vi "UNITEST MAIN v01.2.vi"() -> ()   [LabVIEW 2025]
uses:
  controls/LAB-IQ UI Data.ctl
  HEAVE vi's/Heave Write enum.ctl
  487e97dd-ad82-4ea8-9260-f35915b83a37.vi
  fdf22e40-24ec-4bd6-b058-052306f15f2c.vi
  02c5850b-52e8-4ed5-91f8-6f0ad62f4994.vi
  1223eb78-e4c4-4b69-bf80-185c82055158.vi
  e5651a45-6a49-4a3f-b503-ff1eaf449b4a.vi
  support/Message Queue/Enqueue Message (Single).vi
  <vilib>/Utility/error.llb/Error Cluster From Error Code.vi
  <vilib>/ErrorRing/Error Ring.xnode
  support/Message Queue/LAB-IQ Message Queue.lvlib
  support/User Event - Stop/LAB-IQ User Event - Stop.lvlib
  d081153b-36ca-4bc4-8478-749476f82ba4.vi
  HEAVE vi's/Heave Right enum.ctl
panel:
  in  "seconds to wait":dbl=0.0001 format="%#_6p"
  out "error out":errorcluster
  in  "error in (no error)":errorcluster
  out "Heave and Surge Read":string
  in  "min_finetune_floor":dbl=0.15
  in  "min_deadband_floor":dbl=0.05
  in  "fine_tune_pct":dbl=100.0
  out "Start Test Temp":bool
  in  "STOP":bool
  in  "AppLoadSeq scratch":bool
  out "Pulse delta":dbl
  in  "Fine Tune Zone":dbl=10.0
  in  "PID Delay (sec)":dbl=1.0 format="%#_6p"
  in  "Max_pos_limit":dbl=50000000.0
  in  "Min_pos_limit":dbl
  in  "i_limit":dbl=10.0
  in  "Max Step Linit":dbl=10.0
  in  "Init Step":dbl=10.0
  in  "pct_scale":dbl=100.0
  in  "Deadband":dbl=0.1
  in  "Kd":dbl
  in  "Ki":dbl
  in  "Kp":dbl=1.0
  out "Current Position":dbl
  in  "Set Load":dbl
  in  "Current Load":dbl
  in  "Manual Write Heave & Surge":bool
  out "Heave and Surge Write":string
  in  "Heave Loop Delay":dbl
  in  "Heave PID Speed":dbl=15.0
  in  "Surge Jog Speed":dbl=1.0 format="%.4f"
  in  "Heave Jog Speed":dbl=15.0
  in  "SPARE 4":u8
  in  "SPARE 3":u8
  in  "SPARE 2":u8
  in  "SPARE 1":u8
  out "Spare 15":u8
  out "Spare 14":u8
  out "Spare 13":u8
  out "Spare 12":u8
  out "Spare 11":u8
  out "Spare 10":u8
  out "Spare 9":u8
  out "Spare 8":u8
  out "Spare 7":u8
  out "Spare 6":u8
  out "Spare 5":u8
  out "Spare 4":u8
  out "Spare 3":u8
  out "Spare 2":u8
  out "Spare 1":u8
  out "Node Id":u8
  out "Read Heave Temp":bool
  out "fwMinor":u8
  out "fwMajor":u8
  out "faultCode":u16
  out "SURGE POSE":sgl format="%#.6f"
  out "HEAVE POSE":sgl format="%#.6f"
  out "Homed":u8
  out "State":u8
  out "Ack ID":u16
  in  "SPEED":sgl=10000.0
  in  "Distance":sgl=10000.0
  in  "Mode Command":u8=2
  out "Sequence ID":u16
  out "error out Read":errorcluster
  out "error out Write":errorcluster
  out "Heave and Surge Read":string
  out "Load Cell Temp":bool
  in  "Stop Scratch":bool
  in  "Enter Fixed SRR 2":dbl min=0.0 max=0.0 format="%.3f"
  in  "E.Velocity 2":bool=TRUE caption="SRR"
  out "Message":string="Load Entered is out of range!!!"
  in  "Tab Control 3":T1(tab)
  in  "Tab Control 5":enum32{""}(tab)
  in  "Tab Control 14":T2(tab)=enum."Motor Load"
  in  "Ramp MulFac":dbl=2.0
  in  "pulses LoadDiffRamp(2..10)":dbl=9.0
  in  "PulseControlRamp(diff<=3N)":dbl=5.0 min=1.0 max=1000.0 step=1.0 format="%#.1f"
  in  "SetLoadDeadband(%) Load(0-10N)":dbl=0.1 min=0.0001 max=100.0 step=0.0001 format="%#.6f"
  in  "PID gains out delay (microForce)":T3={"proportional gain (Kc)"=300.0, "integral time (Ti, min)"=0.00011, "derivative time (Td, min)"=0.0} {"derivative time (Td, min)" format="%.3f"; "integral time (Ti, min)" min=1e-05 max=100.0 step=1e-06 format="%.6f"; "proportional gain (Kc)" format="%.3f"}
  in  "Ramp":bool
  in  "Gain 2":dbl=0.016
  in  "pulses LoadDiff(2..10)":dbl=10.0
  in  "pulses LoadDiff(11..50)":dbl=40.0
  in  "PulseControl(diff<=3N)":dbl=1.0 min=1.0 max=1000.0 step=1.0 format="%#.1f"
  out "SetLoadDeadband(%)  2":dbl=1.0 min=0.001 max=100.0 step=0.001 format="%#.6f"
  in  "Dummy Run":bool
  out "Vertical load (N)":dbl format="%#.3f"
  in  "AutoTune":bool
  in  "Offset  3":dbl=1.5
  in  "apply load":bool
  in  "Enter ByPass Load":dbl
  in  "reinit 3":bool=TRUE
  in  "output range delay":cluster{"output high":dbl, "output low":dbl}={"output high"=100.0, "output low"=-100.0} {"output low" format="%.2f"; "output high" format="%.2f"}
  in  "PID gains out delay":T3={"proportional gain (Kc)"=30.0, "integral time (Ti, min)"=0.00101, "derivative time (Td, min)"=0.0} {"derivative time (Td, min)" format="%.3f"; "integral time (Ti, min)" min=1e-05 max=100.0 step=0.0001 format="%.4f"; "proportional gain (Kc)" format="%.3f"}
  in  "Bypass Load":bool
  in  "pulsesSent":dbl=200.0
  out "pulses":dbl
  out "actpid":dbl
  out "gFF Rot 7":cluster{dbl, dbl, dbl}(graph)
  in  "pulses LoadDiff(21..1000)":dbl=40.0
  in  "Delay":dbl=1.5 min=0.001 max=5.0 step=0.001 format="%#.6f"
  in  "deadband":dbl=0.2
  in  "Tab Control 26":enum32{"Page 1", "Page 2"}(tab)
  in  "ClearAll":bool
  out "Mz(Nm)":dbl[](array[numeric])
  out "My(Nm)":dbl[](array[numeric])
  out "Mx(Nm)":dbl[](array[numeric])
  in  "Save Dwell":dbl=0.015 caption="Save Dwell (sec)" min=0.0 max=5.0 step=0.001 format="%.3f"
  out "Mx":dbl[](graph)
  out "My":dbl[](graph)
  out "Mz":dbl[](graph)
  out "Fx(N)":dbl[](graph)
  out "Fy(N)":dbl[](graph)
  out "Fz(N)":dbl[](graph)
  in  "ZeroAll":bool
  in  "Acq Delay (ms)":dbl=10.0
  in  "Burst Delay (ms)":dbl=10.0
  out "model":string
  out "SN":i32
  out "FFx(N)":dbl[](array[numeric])
  in  "Sensor IP":string="192.168.1.100"
  in  "Port":i32=8080
  out "FFy(N)":dbl[](array[numeric])
  out "Load(N)":dbl[](array[numeric])
  out "AE":bool
  in  "delete Handle":bool
  in  "Create Handle":bool=TRUE
  out "ft_data":dbl[](array[numeric])=[1.0, 1.0, 1.0, 1.0, 1.0, 1.0]
  out "ft_range":dbl[](array[numeric])=[1.0, 1.0, 1.0, 1.0, 1.0, 1.0]
  in  "stop 6":bool
  out "running_flag":bool
  out "ft_udp_handle":i32
  out "get-data-return":i32
  out "get-range-return":i32
  out "zero-return":i32
  out "filter-return":i32
  out "initial-return":i32
  out "deleteHandle-result":i32
  in  "Tab Control 19":enum32{"Platform COM", "Config ", "DevInfo"}(tab)=enum."Config "
  in  "SAMPLES":dbl=100.0
  in  "Re-initilaize":bool
  in  "Filter ON/OFF":bool=TRUE
  in  "TracHomeSurgeOffsetCounts 10MM":dbl=505100.0
  in  "TracHomeSwayOffsetCounts 10MM":dbl=1432.0
  in  "Acoustic Emission:":dbl=1.0 min=0.0001 max=200.0 step=0.0001 format="%.4f"
  in  "Apply Filter (FF)":bool
  in  "Filter% 2":dbl=50.0 min=50.0 max=100.0 step=0.1 format="%.1f"
  in  "Apply Filter (Load)":bool=TRUE
  in  "Filter%":dbl=80.0 min=50.0 max=100.0 step=0.1 format="%.1f"
  in  "Sway distance (mm)":dbl=245.0
  in  "Surge distance (mm)":dbl=370.0
  in  "DataSavingLoopDelay(ms)":dbl=15.0
  in  "SAVE  2":bool
  in  "Enter Distance":bool caption="Enter Counts"
  in  "Sway Counts:":dbl=100.0 min=0.0 max=100000000.0 step=1.0 format="%.2f"
  in  "Distance (mm): 3":dbl=100.0 caption="Distance (mm):" min=0.0 max=1500.0 step=0.001 format="%.5f"
  in  "Surge Counts:":dbl=100.0 min=0.0 max=100000000.0 step=1.0 format="%.1f"
  in  "Distance (mm): 2":dbl=100.0 caption="Distance (mm):" min=0.0 max=1500.0 step=0.0001 format="%.3f"
  in  "Distance (mm):":dbl=100.0 min=0.0 max=1500.0 step=0.001 format="%.5f"
  in  "Heave Counts:":dbl=100.0 min=0.0 max=100000000.0 step=1.0
  in  "LRMHomeSurgeOffsetCounts":dbl=307197.0
  in  "LRMHomeSwayOffsetCounts":dbl=26880.0
  in  "TracHomeSurgeOffsetCounts 20MM":dbl=505100.0
  in  "TracHomeSwayOffsetCounts 20MM":dbl=1432.0
  in  "RotHomeSwayOffsetCounts":dbl=14656.0
  in  "RotHomeSurgeOffsetCounts":dbl=311465.0
  in  "Heave distance":dbl=340.0
  out "Zmm":dbl=1600.0
  out "Heave Pulses/mm":dbl=1600.0
  out "Surge Pulses/mm":dbl=1600.0
  out "Sway Pulses/mm":dbl=320.0
  in  "Heave Pitch":dbl=4.0
  in  "Surge Pitch":dbl=3.0
  in  "Sway Pitch":dbl=2.0
  in  "Heave PPR":dbl=6400.0
  in  "Surge PPR":dbl=6400.0
  in  "Sway PPR":dbl=6400.0
  in  "GUI":T4(tab)
  in  "Platform Settings":bool caption="Password"
  in  "Configure":bool caption="Password"
  in  "Home":bool caption="Password"
  in  "EXIT":bool
  in  "Analysis":bool caption="Password"
  in  "service 2":bool caption="Password"
  in  "MainPage":T5(tab)=enum."HOME"
  in  "Select Load Head":bool
  in  "Notes :":string
  in  "FILE":string
  in  "Sample ID :":string
  in  "Operator ID :":string
  in  "Operator Name :":string
  in  "Auto":bool caption="Power Status"
  out "mm/s  Surge":dbl=7.0 caption="Jog" min=0.001 max=50.0 step=0.0001 format="%.2f"
  in  "Update Surge Speed":bool
  out "Drive Error":string
  in  "Disable Axis Jog Soft Limits":bool
  out "mm/s  Sway":dbl=7.0 caption="Jog" min=0.001 max=50.0 step=0.0001 format="%.2f"
  out "Sway and Surge COM Status":bool=TRUE caption="Load COM Status"
  out "Heave COM Status":bool=TRUE caption="Load COM Status"
  in  "Enable Platform":bool
  in  "Surge Forward Main":bool
  in  "Surge Backward Main":bool
  in  "Sway Right Main":bool
  in  "Sway Left Main":bool
  in  "Heave Down Main":bool
  in  "Heave Up main":bool
  in  "Update Sway Speed":bool
  in  "Update Heave Speed":bool
  out "mm/s Heave":dbl=7.0 caption="Jog" min=0.001 max=30.0 step=0.0001 format="%.2f"
  in  "mm/sec":dbl=1.0 caption="Jog" min=0.001 max=50.0 step=0.001 format="%.2f"
  in  "mm":dbl=0.001 caption="Jog" min=0.001 max=200.0 step=0.0001 format="%#.3f"
  in  "Surface Analysis":bool
  in  "Imaging":bool
  in  "Image Analysis":bool
  in  "Post Analysis":bool
  in  "SSP 0.75":bool
  in  "SSP 0.5":bool
  in  "SSP 0.3":bool
  in  "Warning":enum32{"Page 2"}(tab)
  in  "gui GIF":enum32{"Check", "Deca", "kilo", "Micro"}(tab)
  out "Communication is established":bool=TRUE caption="Load COM Status"
  in  "Reference Sample":u16(ring) items=["None", "Brass", "Aluminium", "Mild Steel"]
  out "Load Cell Communication Slide":u8(slide)=1 min=1 max=10 step=1 scale=0.0..10.0
  in  "com 3":bool
  out "com":bool
  out "DecaForce COM Status":bool caption="Load COM Status"
  in  "Loading Mode":u16(ring) items=["Constant", "Ramp", "Steps", "Indentation"]
  in  "Enter the CoF Trip":dbl=1.0
  in  "Enter the Friction Force Trip":dbl=520.0 min=500.0 max=500.0 step=1.0 format="%#.1f"
  in  "Enter the Normal load Trip":dbl=520.0 min=500.0 max=500.0 step=0.001 format="%.3f"
  in  "KiloForce":bool
  in  "DecaForce":bool
  in  "MicroForce":bool
  in  "LHBack":bool
  in  "LHNext":bool
  in  "Load Selection":T6(tab)
  in  "Enter the Load  (N)":dbl=2.0 min=2.0 max=50.0 step=0.1 format="%#.4f"
  in  "Enter the Final Load (N)":dbl=1.0 min=0.0 max=500.0 step=1.0 format="%#.0f"
  in  "Update":bool
  in  "Enter the Loading Rate (N/min)":dbl=60.0 min=60.0 max=1200.0 step=0.1 format="%.2f"
  out "Warning 2":bool
  in  "Stribeck Table  For loading":string[][](table)=[["", "", ""], ["", "", ""], ["", "", ""], ["", "", ""]]
  in  "Stribeck table":bool
  in  "seq":bool=TRUE
  in  "Clear 3":bool
  in  "Indentation":string[][](table)=[["Detection", "5", "2"], ["Unload", "0", "5"], ["Load", "10", "2"], ["Unload", "0", "5"], ["Detection", "5", "2"], ["Unload", "0", "5"]]
  in  "Multipoint":bool caption="Singlepoint"
  in  "AppLoad 4":bool
  in  "zNL":bool
  out "NL disp":dbl caption="Normal Load ( N )" min=-2000.0 max=2000.0 step=0.0001 format="%.1f"
  in  "Traction":bool
  in  "Surge Forward MM":bool
  in  "Surge Backward MM":bool
  in  "M3 Image":enum32{"Page 1", "Page 2"}(tab)
  in  "String 39":string="Jog heave to bring the upper sample closer to the lower sample within 1mm."
  in  "Sway Left MM":bool
  in  "Sway Right MM":bool
  in  "Disable Axis Jog Soft Limits":bool
  in  "mm":dbl=0.001 caption="Jog" min=0.001 max=5.0 step=0.0001 format="%#.3f"
  in  "Heave Down MM":bool
  in  "Heave Up MM":bool
  in  "Wear Track Diameter (mm)":dbl=5.0 caption="Wear Track Diameter (mm):" min=1.0 max=30.0 step=1.0 format="%.2f"
  in  "Set WTD":bool
  in  "HomeScratch":bool
  in  "HomeRot":bool
  in  "PlaceModule":bool
  in  "Motion Mode:":u16(ring) items=["Uniform Rotation", "Angular Oscillation", "Stribeck ", "Steps"]
  in  "LR Sway":bool
  in  "Rot Hor":bool
  in  "Rot Ver":bool
  in  "Scratch":bool
  in  "LR Cam":bool
  in  "MMBack":bool
  in  "MMNext":bool
  in  "Rotary Module Selection":T7(tab)
  in  "SPEED SELECTION :":enum32{"Speed in RPM", "Speed in m/sec"}(radio)=enum."Speed in m/sec"
  in  "TEST SELECTION":enum32{"Time", "Cycle"}(radio)
  in  "Enter the Speed(mm/sec)":dbl=1.0 min=0.1 max=10.0 step=0.1 format="%.1f"
  in  "Enter the Speed(RPM)":dbl=45.0 min=5.0 max=300.0 step=1.0
  in  "Enter the Frequency (Hz)":dbl=1.0 min=0.1 max=10.0 step=0.1 format="%.1f"
  in  "Enter the Angle (Deg)":dbl=45.0 min=5.0 max=300.0 step=1.0
  in  "Angular Oscillation Set":bool
  in  "Rotary Tab":enum32{"Page 1", "Page 2"}(tab)
  out "e.v/ssr 2":enum32{"E.V", "SSR"}(tab)
  in  "Enter the Final E.Velocity (m/s) 2":dbl=1.0 min=0.001 max=4.0 step=0.001 format="%.3f"
  in  "Enter initial E.Velocity (m/s) 2":dbl=2.0 min=0.001 max=4.0 step=0.001 format="%.3f"
  in  "Enter Fixed E.Velocity 2":dbl=1.0 min=0.001 max=2.0 step=0.001 format="%.3f"
  in  "Enter Final SRR 2":dbl=1.0 min=0.001 max=1.0 step=0.001 format="%.2f"
  in  "Enter initial SRR 2":dbl=1.0 min=0.001 max=1.0 step=0.001 format="%.2f"
  out "Final Speed (RPM) 3":dbl=1.0 min=0.1 max=3000.0 step=0.1 format="%.1f"
  out "Initial Speed (RPM) 2":dbl=100.0 min=0.1 max=3000.0 step=0.1 format="%.1f"
  in  "Enter the Final Velocity (m/s) 3":dbl=1.0 min=0.001 max=2.0 step=0.001 format="%.3f"
  in  "Enter initial Velocity (m/s)  3":dbl=2.0 min=0.001 max=2.0 step=0.001 format="%.3f"
  out "Ramp Up 2":bool caption="Ramp Down"
  in  "File Path :  2":path
  in  "Import 2":bool
  in  "Save 2":bool
  in  "SPEED SELECTION : rotary":enum32{"Speed in Rpm", "Speed in m/sec"}(radio)=enum."Speed in m/sec"
  in  "calculate rotary":bool
  in  "String 45":string="File Path Location : C:-->LAB-IQ 150 --> User Defined\n                                       Protocol-->File.txt"
  in  "Step Speed":enum32{"Step Speed", "Step (load-Speed)"}(tab)
  in  "StepTable For Speed":string[][](table)=[["", "", ""], ["", "", ""], ["", "", ""], ["", "", ""]]
  in  "StepTable For Load-Speed":string[][](table)=[["", "", ""], ["", "", ""], ["", "", ""], ["", "", ""]]
  in  "StepTable For Speed 3":string[][](table)=[["", "", ""], ["", "", ""], ["", "", ""], ["", "", ""]]
  in  "Motion Direction:  3":u16(ring) items=["Clockwise", "Counter Clockwise"]
  out "Humidity  Status  3":bool caption="Communication Status"
  out "Low Temp  Status  2":bool caption="Communication Status"
  out "TK4 status 2":bool caption="Communication Status"
  in  "String 40":string="Before selecting Acoustic make sure the sensor output pin is connected to A4."
  in  "Stage Temperature":dbl[](array[numeric])=[150.0, 230.0, 300.0, 350.0, 400.0, 450.0, 500.0]
  in  "Sample Temperature":dbl[](array[numeric])=[100.0, 150.0, 200.0, 250.0, 300.0, 350.0, 400.0]
  in  "Humidity (Amb)":bool
  in  "Clear List":bool
  out "Sensors Picked":string
  in  "Add to list":bool
  in  "Wear":bool
  in  "Vibration":bool
  in  "Humidity (Chamber)":bool
  in  "Temperature (Chamber)":bool
  in  "ECR":bool
  in  "Temperature (Amb)":bool
  in  "Microphone":bool
  in  "Acoustic Emission 3":bool
  in  "SNext":bool
  in  "APBack":bool
  in  "Enter the Temperature (°C):":dbl
  in  "Enter the Stage \nTemperature (°C):":dbl=20.0 min=20.0 max=150.0 step=1.0 format="%#.0f"
  in  "Enter the Humidity (%Rh):":dbl=30.0 min=30.0 max=85.0 step=1.0
  in  "Low Temp":bool
  in  "High Temp":bool
  in  "Humidity":bool
  in  "Main Screen Tab":T8(tab)
  in  "ClrLog":bool
  out "Trip Log":string
  in  "Start Test":bool
  out "Test status":bool caption="Test Status"
  out "AR Led":bool caption="AR"
  out "Data":bool=TRUE
  out "Health":bool=TRUE
  out "Sway COM Status":bool=TRUE caption="Load COM Status"
  out "Heave COM Status":bool=TRUE caption="Load COM Status"
  in  "Grp Tab":enum32{"Rot/LRM", "FBT"}(tab)
  in  "Sub Graph":T9(tab)
  in  "Speed Reset Graph":bool
  in  "Speed Tab":enum32{" Rotary Disc", "MTM Ball", "MTM Disc"}(tab)
  out "speed mm/sec":dbl(graph)=0.13298760003255525
  out "MTM BALL SPEED":dbl(graph)=0.13298760003255525
  out "MTM DISC  SPEED":dbl(graph)=0.13298760003255525
  in  "Temperature Reset":bool
  out "Temperature (deg c)":dbl(graph)=0.13298760003255525
  in  "ECR RESET":bool
  out "ECR":dbl(graph)=0.13298760003255525
  out "Acoustic Emission (mV)":dbl min=0.0 max=5000.0 step=0.1
  in  "Aqucostic Reset Graph":bool
  out "gACQUOS":dbl(graph)=0.13298760003255525
  in  "Humidity Reset Graph":bool
  out "HumrGp":dbl(graph)=0.13298760003255525
  out "SD (mm)":dbl caption="Sliding Distance ( mm )" min=-200.0 max=200.0 step=0.1 format="%.4f"
  in  "Siliding distance Reset Graph":bool
  out "SDGp":dbl(graph)=0.13298760003255525
  out "Hymidity":bool
  in  "Humidity Disable trip":bool=TRUE
  in  "CoF Trip  2":dbl=540.0 min=100.0 max=540.0 step=1.0
  out "Depth Trip":dbl=600.0
  in  "Depth Trip":bool=TRUE
  out "Weart Deapth":bool
  in  "Depth Reset Graph":bool
  out "Weart":bool
  in  "Depthz":bool
  out "Depth (µm)":dbl min=-200.0 max=200.0 step=0.1 format="%.1f"
  out "WearGp":dbl(graph)=0.13298760003255525
  out "NL Trip 2":dbl=600.0
  out "Load pid":bool
  in  "Load Disable Trip":bool=TRUE
  in  "Load Reset Graph":bool
  out "NL Display 4":dbl caption="Normal Load ( N )" min=-2000.0 max=2000.0 step=0.0001 format="%.1f"
  out "Main Chart 3":cluster{dbl, "NL disp":dbl, dbl}(graph)
  in  "FF Tab":T10(tab)
  in  "COF Reset Graph":bool
  in  "COF Disable Trip":bool=TRUE
  out "COF TRIP":dbl=600.0
  out "COF MAIN CHART":cluster{dbl, "NL disp":dbl, dbl}(graph)
  out "Friction Force (N)":dbl min=-2000.0 max=2000.0 step=0.0001 format="%.1f"
  in  "FF Reset Graph":bool
  in  "FF Disable Trip":bool=TRUE
  out "FF TRIP":dbl=600.0
  out "FF MAIN CHART":cluster{dbl, "NL disp":dbl, dbl}(graph)
  in  "BACK":bool
  out "Ambient \nTemperature":dbl min=0.0 max=5000.0 step=0.1 format="%.1f"
  out "Ambient\n Humidity":dbl min=0.0 max=5000.0 step=0.1 format="%.2f"
  out "NL disp 2":dbl caption="Normal Load ( N )" min=-2000.0 max=2000.0 step=0.0001 format="%.1f"
  out "Set Humidity":dbl caption="Set Humidity  (% Rh)" min=-2000.0 max=2000.0 step=1.0 format="%.1f"
  out "humidity disp":dbl caption="Humidity (% Rh)" min=-2000.0 max=2000.0 step=1.0 format="%.1f"
  in  "Humidity On":bool
  in  "zNL 2":bool
  out "NLt":bool
  in  "Load En":bool
  out "Freq (Hz)":dbl min=0.0 max=5000.0 step=0.1 format="%.4f"
  out "HumCOMStatus":bool caption="Communication Status"
  out "Load Communication":bool
  in  "Temp Tabs":enum32{"Low Temp", "High Temp"}(tab)=enum."High Temp"
  out "Controller  Status":bool
  out "ChamberTemp":dbl format="%#.1f"
  in  "SetTmp":dbl=-190.0 caption="Set Temperature (Deg C)" min=-190.0 max=100.0 step=1.0 format="%.1f"
  in  "Cooling":bool
  in  "Heater":bool
  out "TK4 status":bool caption="Controller  Status"
  out "ChamberTemp":dbl format="%#.1f"
  in  "SetTmp":dbl caption="Set Temperature (Deg C)" min=0.0 max=1000.0 step=1.0 format="%.1f"
  in  "Set Load (N)":dbl=100.0 min=0.01 max=1500.0 step=0.01 format="%.1f"
  in  "Time Tab":enum32{"cycles", "duration"}(tab)=enum."duration"
  out "Test Duration 4":dbl=600.0 caption="Test Duration\n(HH:MM:SS)" min=0.0083 max=180000.0 step=0.0001 format="%<%H:%M:%S>t"
  out "TEST CYCLE":dbl min=0.0 max=5000.0 step=0.01 format="%.2f"
  in  "TOTAL CYCLES":dbl min=0.0 max=5000.0 step=0.1 format="%.4f"
  out "Time ( HH:MM:SS ) 2":dbl min=0.0 max=144000.0 step=1.0 format="%<%H:%M:%S>t"
  in  "Test Duration":dbl=600.0 caption="Test Duration\n(HH:MM:SS)" min=0.0083 max=180000.0 step=0.0001 format="%<%H:%M:%S>t"
  in  "Main Speed Tab":enum32{"ROTARY", "TRACTION"}(tab)
  in  "SPEED TAB":enum32{"RPM", "m/sec"}(tab)
  out "Speed (RPM)":dbl min=0.0 max=5000.0 step=0.1 format="%.1f"
  out "Set Speed":dbl caption="Set Speed (RPM)" min=0.0 max=1500.0 step=0.1 format="%.1f"
  out "Speed (m/sec)":dbl min=0.0 max=5000.0 step=0.001 format="%.4f"
  out "Set Speed (m/sec)":dbl min=0.0 max=1500.0 step=0.001 format="%.4f"
  in  "MTM MOTOR DISPLAY":enum32{"MTM RPM", "MTM m/sec"}(tab)
  out "Disc Speed (RPM)":dbl min=0.0 max=1500.0 step=0.1 format="%.1f"
  out "Ball Speed (RPM)":dbl min=0.0 max=1500.0 step=0.1 format="%.1f"
  out "Disc Speed (m/sec)":dbl min=0.0 max=1500.0 step=0.1 format="%.1f"
  out "Ball Speed (m/sec)":dbl min=0.0 max=1500.0 step=0.1 format="%.1f"
  in  "Angle and Frequency":enum32{"angular", "lrm"}(tab)
  out "Angle (Deg)":dbl min=0.0 max=5000.0 step=0.01 format="%.2f"
  out "Stroke (mm)":dbl min=0.0 max=5000.0 step=0.01 format="%.2f"
  in  "Analysis Home":bool
  in  "Password":string
  in  "Home Service":bool
  in  "Advanced Setting":bool
  in  "About Tab":enum32{"Primary"}(tab)
  in  "ECR Port:":refnum<visa-resource-name>="COM10"
  in  "Ramp Port:":refnum<visa-resource-name>="COM10"
  in  "Installation/Replacement completed":bool
  in  "Loahead":bool
  in  "Heave and Surge COM Port:":refnum<visa-resource-name>="COM9"
  in  "Sway COM Port:":refnum<visa-resource-name>="COM10"
  in  "Temp Modbus:":refnum<visa-resource-name>="COM14"
  in  "Humidity Port:":refnum<visa-resource-name>="COM10"
  in  "Edit Gain Constants":bool
  in  "Save Gain Constants":bool
  in  "Service About":bool
  # "load Aquisition off"
  # "load Aquisition On"
  # "Configuration"
  # "Limits for Heave Surge and Sway"
  # "Modules Offset Parameters"
  # "Counts-Distance Calculator"
  # "File Name :"
  # "Ensure the traction module is aligned\n horizontally with the stage before ENABLE."
  # "SET JOG SPEED"
  # "JOG MODE"
  # "Module Selection"
  # "Positioning Control"
  # "Connect the controller\ncable to M3"
  # "Environment"
  # "Sensors"
  # "Data Points"
  # "Data Points"
  # "Data Points"
  # "Data Points"
  # "ohms"
  # "Data Points"
  # "Data Points"
  # "Data Points"
  # "LAB-IQ 150 / UNITEST / WO2456 / UT150  v05 / AUGUST 2025"
  # "NOTE: This operation needs to be done only when the machine is ON."
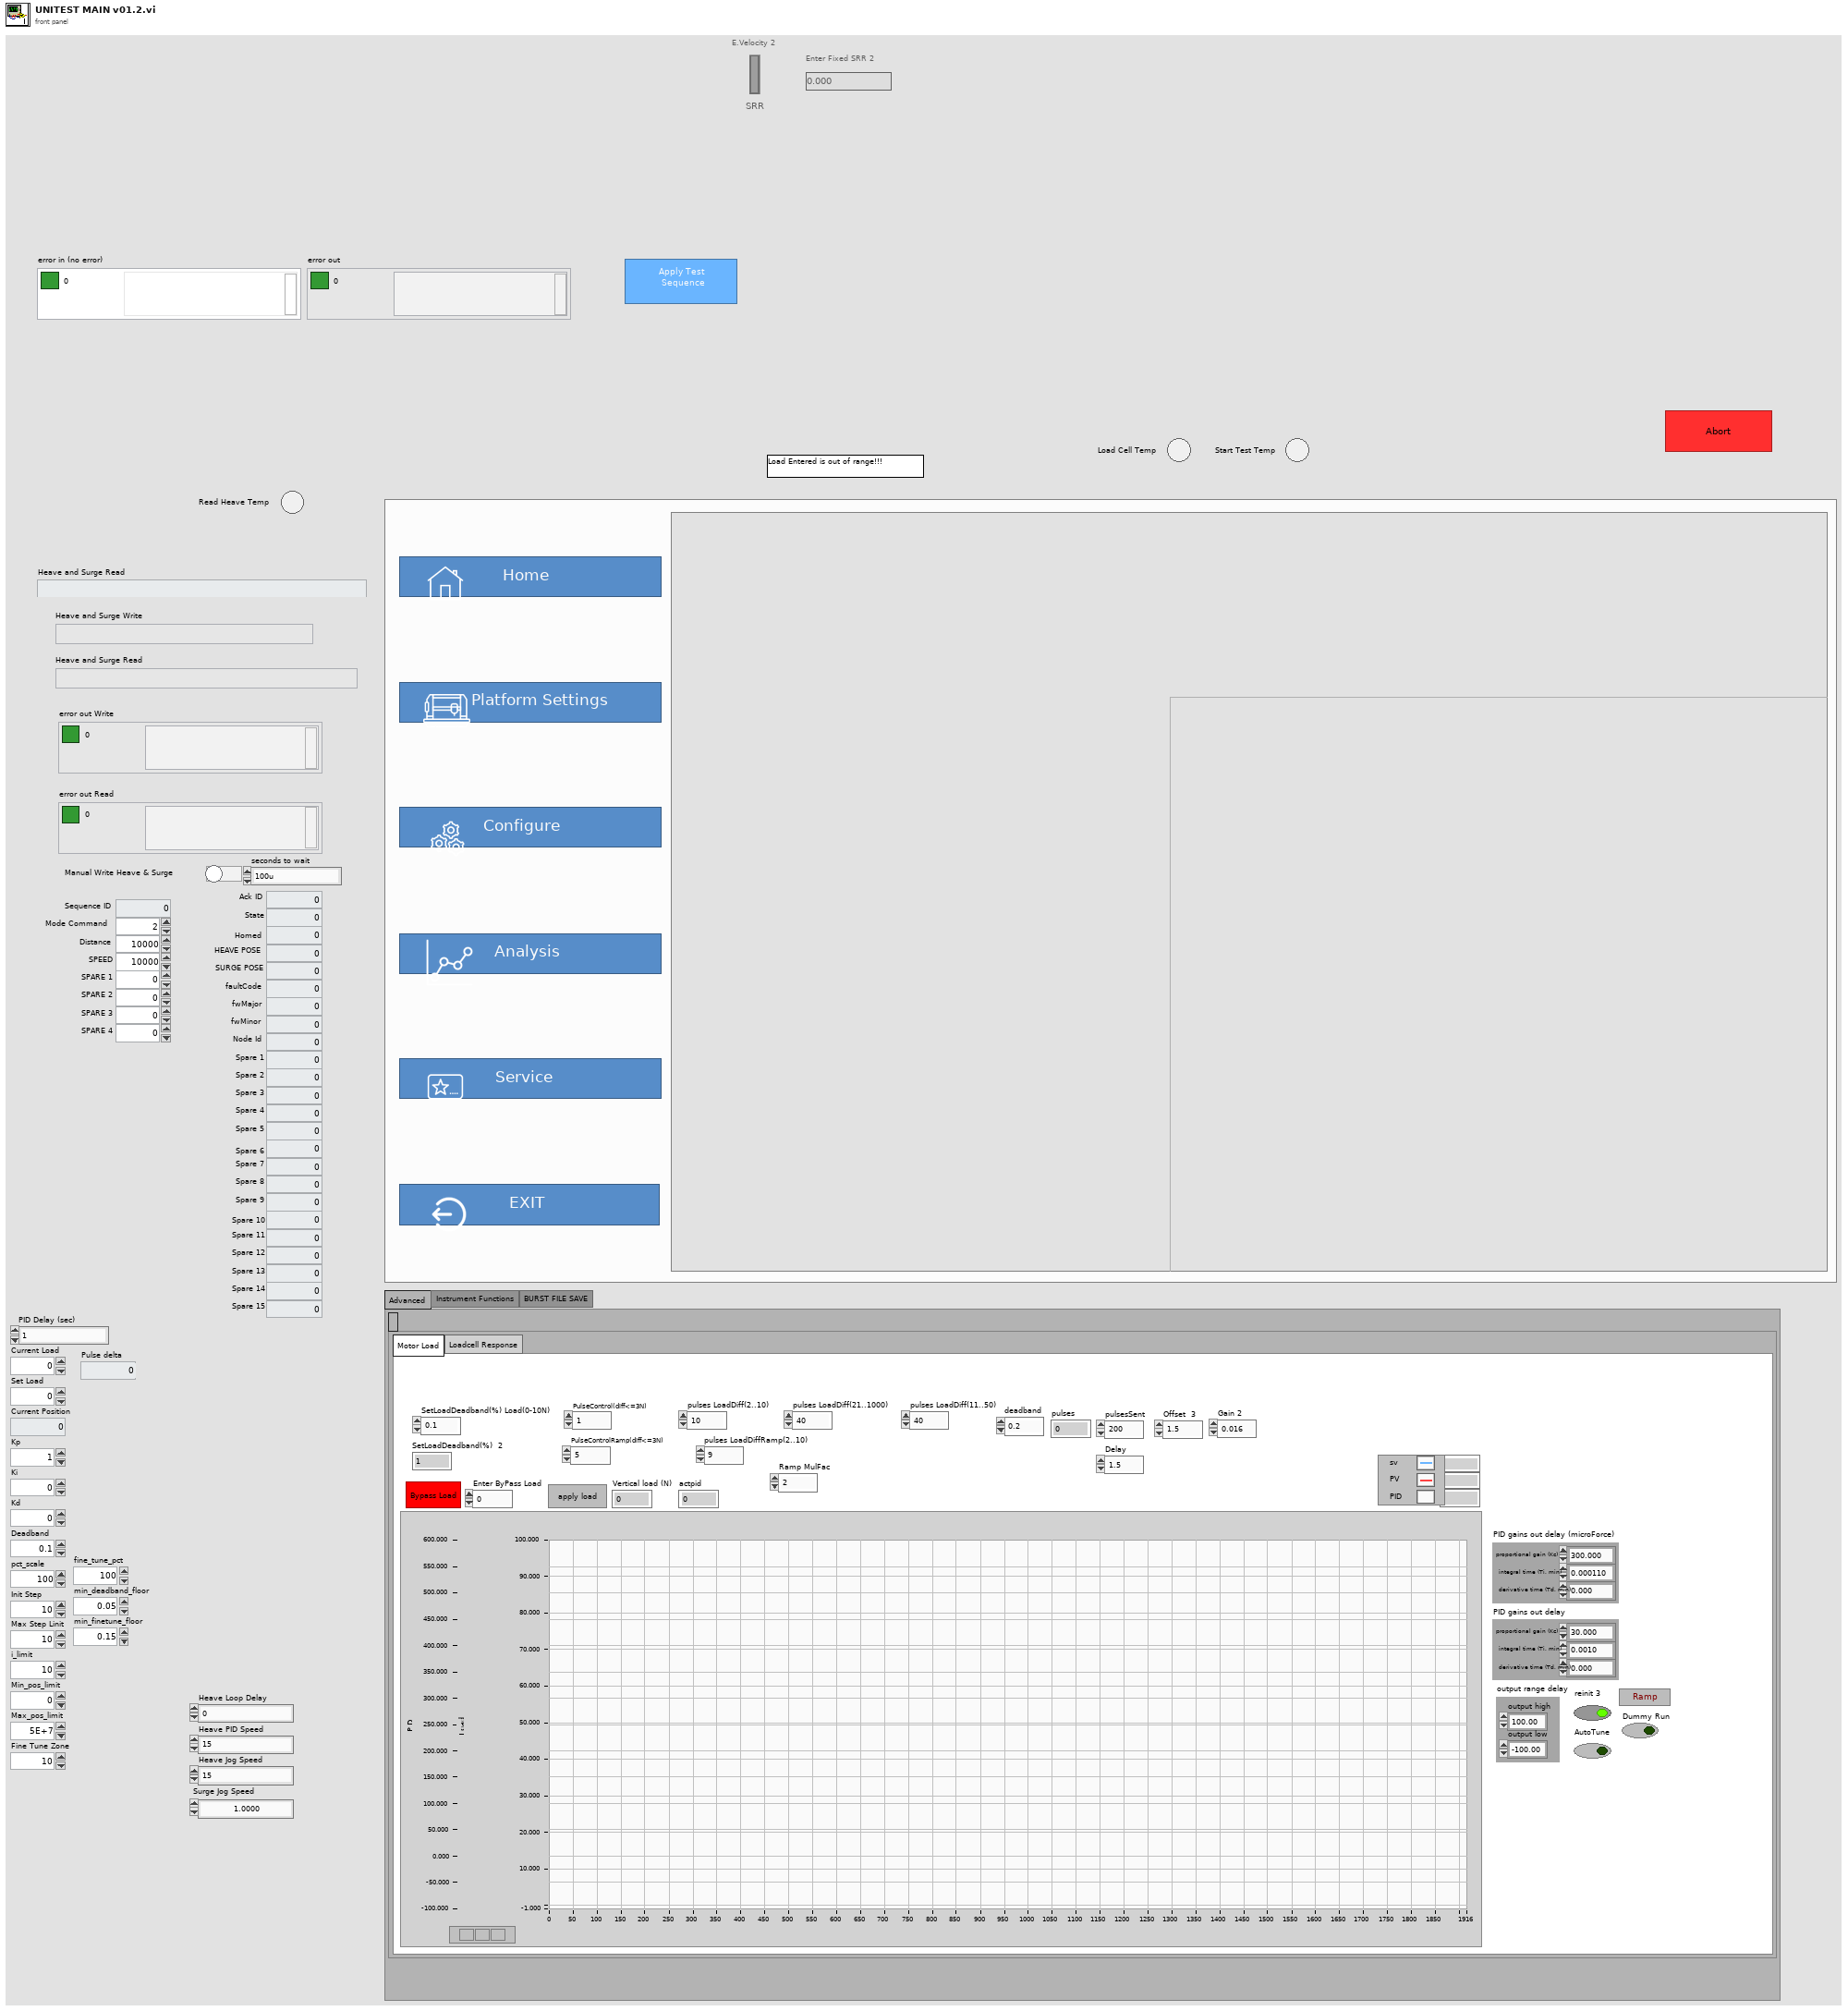
[diagram p1: front panel]
types:
  T1 = enum32{"Advanced", "Motor", "Depth_graph", "UIO Communicator", "Add to list parametrs", "Instrument Functions", "BURST FILE SAVE"}
  T2 = enum32{"LRM heating", "FBT_Heating", "Motor Load", "Loadcell Response", "Voice Load", "Step loading and speed ", "Depth"}
  T3 = cluster{"proportional gain (Kc)":dbl, "integral time (Ti, min)":dbl, "derivative time (Td, min)":dbl}
  T4 = enum32{"Setup", "Load Head", "Motion Module", "Environment", "Begin"}
  T5 = enum32{"Details", "PlatformSetting", "Analysis", "HOME"}
  T6 = enum32{"Constant", "Ramp", "Step", "Indentation"}
  T7 = enum32{"Uniform Rotation", "Angular Oscillation", "Speed Ramp", "Speed Step"}
  T8 = enum32{"  Acquire  ", "Compare Files Rot", "About", "Service"}
  T9 = enum32{"Speed", "Temperature", "ECR", "Acoustic Emission", "Humidity", "Sliding Distance"}
  T10 = enum32{"Coefficient of Friction ", "Friction Force (N)"}
  T11 = typedef "Heave Write enum.ctl" = enum16{"INIT", "WRITE", "CLOSE", "REINIT"}
  T12 = typedef "LAB-IQ UI Data.ctl" = cluster{"Main Home Screen":cluster{"GUI":refnum<vi>, "Platform Settings":refnum<vi>, "Configure":refnum<vi>, "Home":refnum<vi>, "EXIT":refnum<vi>, "service 2":refnum<vi>, "MainPage":refnum<vi>, "Analysis":refnum<vi>}, "Platform Settings":cluster{"mm/s  Surge":refnum<vi>, "Update Surge Speed":refnum<vi>, "Drive Error":refnum<vi>, "Disable Axis Jog Soft Limits":refnum<vi>, "mm/s  Sway":refnum<vi>, "Sway and Surge COM Status":refnum<vi>, "Heave COM Status":refnum<vi>, "Enable Platform":refnum<vi>, "Surge Forward Main":refnum<vi>, "Sway Right Main":refnum<vi>, "Sway Left Main":refnum<vi>, "Heave Down Main":refnum<vi>, "Heave Up main":refnum<vi>, "Update Sway Speed":refnum<vi>, "Update Heave Speed":refnum<vi>, "mm/s Heave":refnum<vi>, "mm/sec":refnum<vi>, "mm":refnum<vi>, "Surge Backward Main":refnum<vi>}, "Analysis Screen":cluster{"Analysis Home":refnum<vi>, "Surface Analysis":refnum<vi>, "Imaging":refnum<vi>, "Image Analysis":refnum<vi>, "Post Analysis":refnum<vi>}, "Config Screen":cluster{"Select Load Head":refnum<vi>, "Notes :":refnum<vi>, "FILE":refnum<vi>, "Sample ID :":refnum<vi>, "Operator ID :":refnum<vi>, "Operator Name :":refnum<vi>, "Auto":refnum<vi>}, "Motion Module":cluster{"zNL":refnum<vi>, "NL disp":refnum<vi>, "Rotary Tab":refnum<vi>, "Motion Direction:  3":refnum<vi>, "E.Velocity 2":refnum<vi>, "e.v/ssr 2":refnum<vi>, "Enter Fixed E.Velocity 2":refnum<vi>, "Enter Final SRR 2":refnum<vi>, "Enter initial SRR 2":refnum<vi>, "Enter Fixed SRR 2":refnum<vi>, "Enter the Final E.Velocity (m/s) 2":refnum<vi>, "Enter initial E.Velocity (m/s) 2":refnum<vi>, "Final Speed (RPM) 3":refnum<vi>, "Initial Speed (RPM) 2":refnum<vi>, "Enter the Final Velocity (m/s) 3":refnum<vi>, "Enter initial Velocity (m/s)  3":refnum<vi>, "Ramp Up 2":refnum<vi>, "TEST SELECTION":refnum<vi>, "SPEED SELECTION : ":refnum<vi>, "Angular Oscillation Set":refnum<vi>, "Traction":refnum<vi>, "Step Speed":refnum<vi>, "StepTable For Load-Speed":refnum<vi>, "StepTable For Speed":refnum<vi>, "Surge Forward MM":refnum<vi>, "Surge Backward MM":refnum<vi>, "M3 Image":refnum<vi>, "String 39":refnum<vi>, "Sway Left MM":refnum<vi>, "Sway Right MM":refnum<vi>, "Disable Axis Jog Soft Limits":refnum<vi>, "mm":refnum<vi>, "Heave Down MM":refnum<vi>, "Heave Up MM":refnum<vi>, "Wear Track Diameter (mm)":refnum<vi>, "Set WTD":refnum<vi>, "HomeScratch":refnum<vi>, "HomeRot":refnum<vi>, "PlaceModule":refnum<vi>, "Enter the Angle (Deg)":refnum<vi>, "Enter the Frequency (Hz)":refnum<vi>, "Motion Mode:":refnum<vi>, "LR Sway":refnum<vi>, "Rot Hor":refnum<vi>, "Scratch":refnum<vi>, "LR Cam":refnum<vi>, "MMBack":refnum<vi>, "MMNext":refnum<vi>, "Rot Ver":refnum<vi>, "Rotary Module Selection":refnum<vi>, "calculate rotary":refnum<vi>, "SPEED SELECTION : rotary":refnum<vi>, "Import 2":refnum<vi>, "Save 2":refnum<vi>, "File Path :  2":refnum<vi>, "String 45":refnum<vi>, "StepTable For Speed 3":refnum<vi>, "Enter the Speed(mm/sec)":refnum<vi>, "Enter the Speed(RPM)":refnum<vi>}, "Environmental control":cluster{"Humidity  Status  3":refnum<vi>, "Low Temp  Status  2":refnum<vi>, "TK4 status 2":refnum<vi>, "Stage Temperature":refnum<vi>, "Sample Temperature":refnum<vi>, "Humidity (Amb)":refnum<vi>, "Clear List":refnum<vi>, "Add to list":refnum<vi>, "Wear":refnum<vi>, "Vibration":refnum<vi>, "Humidity (Chamber)":refnum<vi>, "Temperature (Chamber)":refnum<vi>, "ECR ":refnum<vi>, "Temperature (Amb)":refnum<vi>, "Microphone":refnum<vi>, "Acoustic Emission 3":refnum<vi>, "SNext":refnum<vi>, "APBack":refnum<vi>, "Enter the Temperature (°C):":refnum<vi>, "Enter the Stage \nTemperature (°C):":refnum<vi>, "Enter the Humidity (%Rh):":refnum<vi>, "Low Temp":refnum<vi>, "High Temp":refnum<vi>, "Humidity":refnum<vi>, "Sensors Picked":refnum<vi>}, "About Screen":cluster{"Password":refnum<vi>, "Home Service":refnum<vi>, "Advanced Setting":refnum<vi>, "About Tab":refnum<vi>, "ECR Port:":refnum<vi>, "Ramp Port:":refnum<vi>, "Installation/Replacement completed":refnum<vi>, "Loahead":refnum<vi>, "Heave and Surge COM Port:":refnum<vi>, "Sway COM Port:":refnum<vi>, "Temp Modbus:":refnum<vi>, "Humidity Port:":refnum<vi>, "Edit Gain Constants":refnum<vi>, "Save Gain Constants":refnum<vi>}, "Main Screen":cluster{"Main Screen Tab":refnum<vi>, "Angle and Frequency":refnum<vi>, "Stroke (mm)":refnum<vi>, "Angle (Deg)":refnum<vi>, "Main Speed Tab":refnum<vi>, "MTM MOTOR DISPLAY":refnum<vi>, "Disc Speed (m/sec)":refnum<vi>, "Ball Speed (m/sec)":refnum<vi>, "Disc Speed (RPM)":refnum<vi>, "Ball Speed (RPM)":refnum<vi>, "SPEED TAB":refnum<vi>, "Speed (m/sec)":refnum<vi>, "Set Speed (m/sec)":refnum<vi>, "Speed (RPM)":refnum<vi>, "Set Speed":refnum<vi>, "Time Tab":refnum<vi>, "Time ( HH:MM:SS ) 2":refnum<vi>, "Test Duration":refnum<vi>, "Test Duration 4":refnum<vi>, "TEST CYCLE":refnum<vi>, "TOTAL CYCLES":refnum<vi>, "Set Load (N)":refnum<vi>, "Temp Tabs":refnum<vi>, "Heater":refnum<vi>, "TK4 status":refnum<vi>, "ChamberTemp":refnum<vi>, "SetTmp":refnum<vi>, "Controller  Status":refnum<vi>, "ChamberTemp 2":refnum<vi>, "SetTmp 2":refnum<vi>, "Controller  Status 2":refnum<vi>, "ChamberTemp 3":refnum<vi>, "SetTmp 3":refnum<vi>, "Cooling":refnum<vi>, "Load Communication":refnum<vi>, "Ambient \nTemperature":refnum<vi>, "HumCOMStatus":refnum<vi>, "Ambient\n Humidity":refnum<vi>, "Freq (Hz)":refnum<vi>, "Load En":refnum<vi>, "NLt":refnum<vi>, "zNL 2":refnum<vi>, "Humidity On":refnum<vi>, "humidity disp":refnum<vi>, "Set Humidity":refnum<vi>, "NL disp 2":refnum<vi>, "Humidity On 2":refnum<vi>, "humidity disp 2":refnum<vi>, "Set Humidity 2":refnum<vi>, "NL disp 3":refnum<vi>, "AppLoadSeq scratch":refnum<vi>, "Stop Scratch":refnum<vi>, "ClrLog":refnum<vi>, "Trip Log":refnum<vi>, "STOP":refnum<vi>, "Start Test":refnum<vi>, "Test status":refnum<vi>, "AR Led":refnum<vi>, "Data":refnum<vi>, "Health":refnum<vi>, "Sway COM Status":refnum<vi>, "Heave COM Status":refnum<vi>, "Grp Tab":refnum<vi>, "Sub Graph":refnum<vi>, "SD (mm)":refnum<vi>, "Siliding distance Reset Graph":refnum<vi>, "SDGp":refnum<vi>, "Humidity Reset Graph":refnum<vi>, "HumrGp":refnum<vi>, "Acoustic Emission (mV)":refnum<vi>, "Aqucostic Reset Graph":refnum<vi>, "gACQUOS":refnum<vi>, "ECR RESET":refnum<vi>, "ECR":refnum<vi>, "Temperature Reset":refnum<vi>, "Acoustic Emission (mV) 2":refnum<vi>, "Aqucostic Reset Graph 2":refnum<vi>, "gACQUOS 2":refnum<vi>, "ECR RESET 2":refnum<vi>, "ECR 2":refnum<vi>, "Temperature Reset 2":refnum<vi>, "Temperature (deg c)":refnum<vi>, "Speed Reset Graph":refnum<vi>, "Speed Tab":refnum<vi>, "MTM DISC  SPEED":refnum<vi>, "MTM BALL SPEED":refnum<vi>, "speed mm/sec":refnum<vi>, "Hymidity":refnum<vi>, "Humidity Disable trip":refnum<vi>, "CoF Trip  2":refnum<vi>, "Depth Trip":refnum<vi>, "Weart Deapth":refnum<vi>, "Depth Reset Graph":refnum<vi>, "Weart":refnum<vi>, "Depthz":refnum<vi>, "Depth (µm)":refnum<vi>, "WearGp":refnum<vi>, "NL Trip 2":refnum<vi>, "Load pid":refnum<vi>, "Load Disable Trip":refnum<vi>, "Load Reset Graph":refnum<vi>, "NL Display 4":refnum<vi>, "Main Chart 3":refnum<vi>, "BACK":refnum<vi>, "Depth Trip 2":refnum<vi>, "COF TRIP ":refnum<vi>, "Friction Force (N)":refnum<vi>, "FF Reset Graph":refnum<vi>, "FF Disable Trip":refnum<vi>, "FF TRIP":refnum<vi>, "FF MAIN CHART":refnum<vi>, "COF Disable Trip":refnum<vi>, "COF Reset Graph":refnum<vi>, "COF MAIN CHART":refnum<vi>, "FF Tab":refnum<vi>, "Start Test Temp":refnum<vi>}, "Loading":cluster{"Indentation":refnum<vi>, "Reference Sample":refnum<vi>, "Load Cell Communication Slide":refnum<vi>, "com 3":refnum<vi>, "com":refnum<vi>, "DecaForce COM Status":refnum<vi>, "Update":refnum<vi>, "Clear 3":refnum<vi>, "seq":refnum<vi>, "Stribeck table":refnum<vi>, "Stribeck Table  For loading":refnum<vi>, "Loading Mode":refnum<vi>, "Enter the Final Load (N)":refnum<vi>, "Enter the CoF Trip":refnum<vi>, "Enter the Friction Force Trip":refnum<vi>, "Enter the Normal load Trip":refnum<vi>, "Enter the Load  (N)":refnum<vi>, "KiloForce":refnum<vi>, "DecaForce ":refnum<vi>, "MicroForce":refnum<vi>, "LHBack":refnum<vi>, "LHNext":refnum<vi>, "Enter the Loading Rate (N/min)":refnum<vi>, "Message":refnum<vi>, "Warning 2":refnum<vi>, "SSP 0.75":refnum<vi>, "SSP 0.5":refnum<vi>, "SSP 0.3":refnum<vi>, "Warning":refnum<vi>, "gui GIF":refnum<vi>, "Communication is established":refnum<vi>, "AppLoad 4":refnum<vi>, "Multipoint":refnum<vi>, "Load Selection":refnum<vi>}, "PID":cluster{"Ramp MulFac":refnum<vi>, "pulses LoadDiffRamp(2..10)":refnum<vi>, "PulseControlRamp(diff<=3N)":refnum<vi>, "SetLoadDeadband(%) Load(0-10N)":refnum<vi>, "PID gains out delay (microForce)":refnum<vi>, "Ramp":refnum<vi>, "Gain 2":refnum<vi>, "pulses LoadDiff(2..10)":refnum<vi>, "pulses LoadDiff(11..50)":refnum<vi>, "PulseControl(diff<=3N)":refnum<vi>, "SetLoadDeadband(%)  2":refnum<vi>, "Dummy Run":refnum<vi>, "Vertical load (N)":refnum<vi>, "AutoTune":refnum<vi>, "Offset 3 ":refnum<vi>, "apply load":refnum<vi>, "Offset  3":refnum<vi>, "apply load 2":refnum<vi>, "Enter ByPass Load":refnum<vi>, "reinit 3":refnum<vi>, "output range delay":refnum<vi>, "PID gains out delay":refnum<vi>, "Bypass Load":refnum<vi>, "pulsesSent":refnum<vi>, "pulses ":refnum<vi>, "actpid":refnum<vi>, "gFF Rot":refnum<vi>, "pulses LoadDiff(21..1000)":refnum<vi>, "Delay":refnum<vi>, "deadband":refnum<vi>}, "Config Parameters":cluster{"Tab Control 3":refnum<vi>, "Tab Control 19":refnum<vi>, "SAMPLES":refnum<vi>, "Re-initilaize":refnum<vi>, "Filter ON/OFF":refnum<vi>, "TracHomeSurgeOffsetCounts 10MM":refnum<vi>, "TracHomeSwayOffsetCounts 10MM":refnum<vi>, "Acoustic Emission:":refnum<vi>, "Apply Filter (FF)":refnum<vi>, "Filter% 2":refnum<vi>, "Apply Filter (Load)":refnum<vi>, "Filter% ":refnum<vi>, "Sway distance (mm)":refnum<vi>, "Surge distance (mm)":refnum<vi>, "DataSavingLoopDelay(ms)":refnum<vi>, "SAVE 2":refnum<vi>, "Enter Distance":refnum<vi>, "Sway Counts:":refnum<vi>, "Distance (mm): 3":refnum<vi>, "Surge Counts:":refnum<vi>, "Distance (mm): 2":refnum<vi>, "Distance (mm):":refnum<vi>, "Heave Counts:":refnum<vi>, "LRMHomeSurgeOffsetCounts":refnum<vi>, "LRMHomeSwayOffsetCounts":refnum<vi>, "TracHomeSurgeOffsetCounts 20MM":refnum<vi>, "TracHomeSwayOffsetCounts 20MM":refnum<vi>, "RotHomeSwayOffsetCounts":refnum<vi>, "RotHomeSurgeOffsetCounts":refnum<vi>, "Heave distance":refnum<vi>, "Zmm":refnum<vi>, "Heave Pulses/mm":refnum<vi>, "Surge Pulses/mm":refnum<vi>, "Sway Pulses/mm":refnum<vi>, "Heave Pitch":refnum<vi>, "Surge Pitch":refnum<vi>, "Sway Pitch":refnum<vi>, "Heave PPR":refnum<vi>, "Surge PPR":refnum<vi>, "Sway PPR":refnum<vi>, "Tab Control 5":refnum<vi>, "Tab Control 14":refnum<vi>, "Tab Control 26":refnum<vi>, "AE":refnum<vi>, "Heave Loop Delay":refnum<vi>, "Heave PID Speed":refnum<vi>, "Surge Jog Speed":refnum<vi>, "Heave Jog Speed":refnum<vi>}, "Loading Com Port":cluster{"ClearAll":refnum<vi>, "Mz(Nm)":refnum<vi>, "My(Nm)":refnum<vi>, "Mx(Nm)":refnum<vi>, "Save Dwell":refnum<vi>, "Mx ":refnum<vi>, "My ":refnum<vi>, "Mz":refnum<vi>, "Fx(N)":refnum<vi>, "Fy(N)":refnum<vi>, "Fz(N)":refnum<vi>, "ZeroAll":refnum<vi>, "Acq Delay (ms)":refnum<vi>, "Burst Delay (ms)":refnum<vi>, "model":refnum<vi>, "SN":refnum<vi>, "FFx(N)":refnum<vi>, "Sensor IP":refnum<vi>, "Port":refnum<vi>, "FFy(N)":refnum<vi>, "Load(N)":refnum<vi>, "delete Handle":refnum<vi>, "Create Handle":refnum<vi>, "ft_data":refnum<vi>, "ft_range":refnum<vi>, "ft_data 2":refnum<vi>, "stop 6":refnum<vi>, "running_flag":refnum<vi>, "ft_udp_handle":refnum<vi>, "get-data-return":refnum<vi>, "get-range-return":refnum<vi>, "zero-return":refnum<vi>, "filter-return":refnum<vi>, "initial-return":refnum<vi>, "deleteHandle-result":refnum<vi>, "Load Cell Temp":refnum<vi>}, "Heave AND Surge":cluster{"SURGE POSE":refnum<vi>, "error out Read":refnum<vi>, "HEAVE POSE":refnum<vi>, "State":refnum<vi>, "Homed":refnum<vi>, "Sequence ID":refnum<vi>, "error out Write":refnum<vi>, "faultCode":refnum<vi>, "Ack ID":refnum<vi>, "SPEED":refnum<vi>, "Distance":refnum<vi>, "Mode Command":refnum<vi>, "Heave and Surge Read":refnum<vi>, "Read Heave Temp":refnum<vi>, "Spare 15":refnum<vi>, "Spare 14":refnum<vi>, "Spare 13":refnum<vi>, "Spare 12":refnum<vi>, "Spare 11":refnum<vi>, "Spare 10":refnum<vi>, "Spare 9":refnum<vi>, "Spare 8":refnum<vi>, "Spare 7":refnum<vi>, "Spare 6":refnum<vi>, "Spare 5":refnum<vi>, "Spare 4":refnum<vi>, "Spare 2":refnum<vi>, "Spare 1":refnum<vi>, "Node Id":refnum<vi>, "Spare 3":refnum<vi>, "SPARE 4":refnum<vi>, "SPARE 3":refnum<vi>, "SPARE 2":refnum<vi>, "SPARE 1":refnum<vi>, "fwMajor":refnum<vi>, "fwMinor":refnum<vi>, "Manual Write":refnum<vi>, "Heave and Surge Write":refnum<vi>}, "New PID LOGIC":cluster{"Fine Tune Zone":refnum<vi>, "PID SDelay":refnum<vi>, "Max_pos_limit":refnum<vi>, "Min_pos_limit":refnum<vi>, "i_limit":refnum<vi>, "pct_scale":refnum<vi>, "Deadband":refnum<vi>, "Kd":refnum<vi>, "Ki":refnum<vi>, "Kp":refnum<vi>, "Current Position":refnum<vi>, "Set Load":refnum<vi>, "Current Load":refnum<vi>, "Pulse delta":refnum<vi>, "Init Step":refnum<vi>, "Max Step Linit":refnum<vi>}}
  T13 = typedef "init queue out loop.ctl" = cluster{"UI Loop":refnum<queue>, "LOAD COM LOOP ":refnum<queue>, "SWAY MOTOR COM LOOP":refnum<queue>, "HEAVE MOTOR COM LOOP":refnum<queue>, "TEMPERATURE COM LOOP":refnum<queue>, "RAMP MOTOR COM LOOP":refnum<queue>, "ECR PORT":refnum<queue>, "HUMIDITY COM PORT":refnum<queue>, "PROGRAM LOOP":refnum<queue>, "MONITOR LOOP":refnum<queue>, "REPORT":refnum<queue>, "LOAD PID":refnum<queue>}
  T14 = typedef "Heave Right enum.ctl" = enum16{"INIT", "READ", "CLOSE", "REINIT", ""}
  T15 = enum8{"Enabled", "Disabled", "Disabled and Grayed Out"}
  T16 = enum16{"INIT", "SETLOWPASSFILTER", "SETZERO", "GETSENSORINFO", "GETRANGE", "ZEROALL", "READDATA", "UNINITIAL", "DELETEHANDLE"}
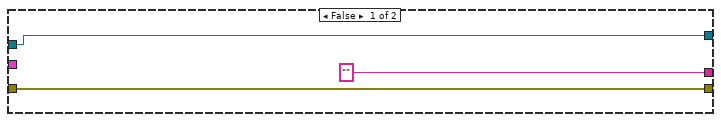
[diagram p2: hidden frame]
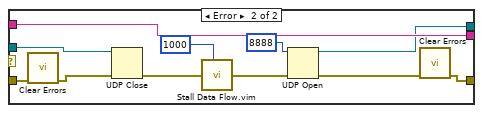
[diagram p3: hidden frame]
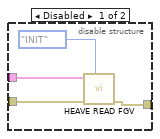
[diagram p4: hidden frame]
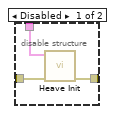
[diagram p5: hidden frame]
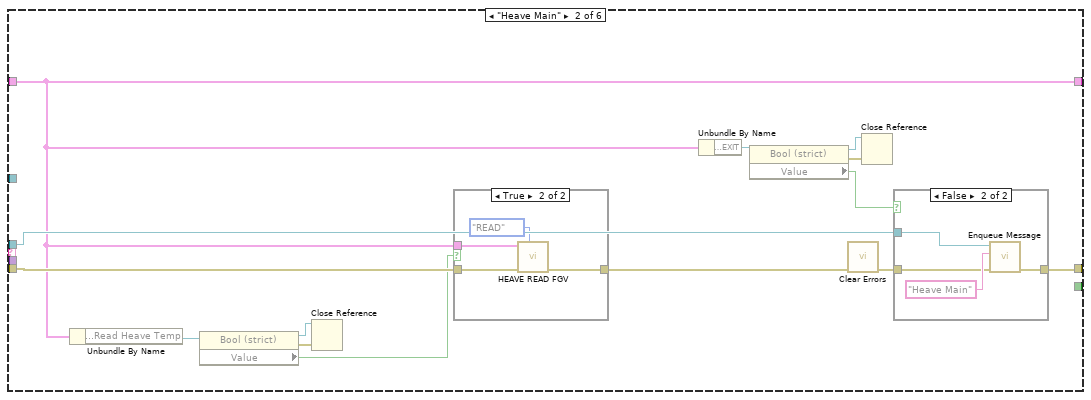
[diagram p6: hidden frame]
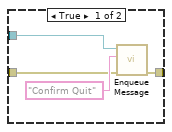
[diagram p8: hidden frame]
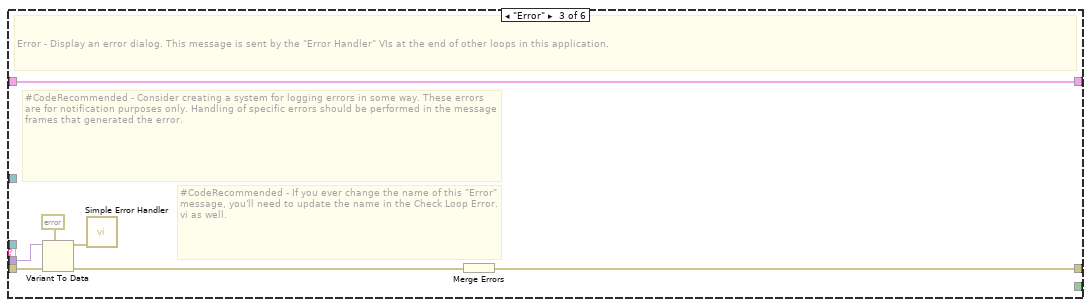
[diagram p9: hidden frame]
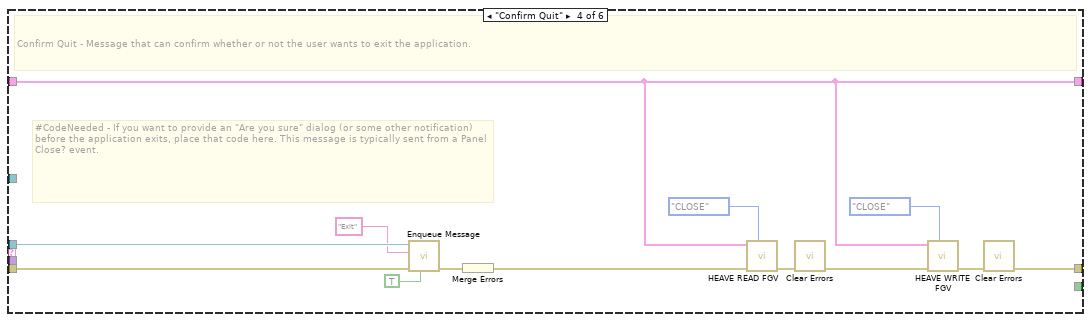
[diagram p10: hidden frame]
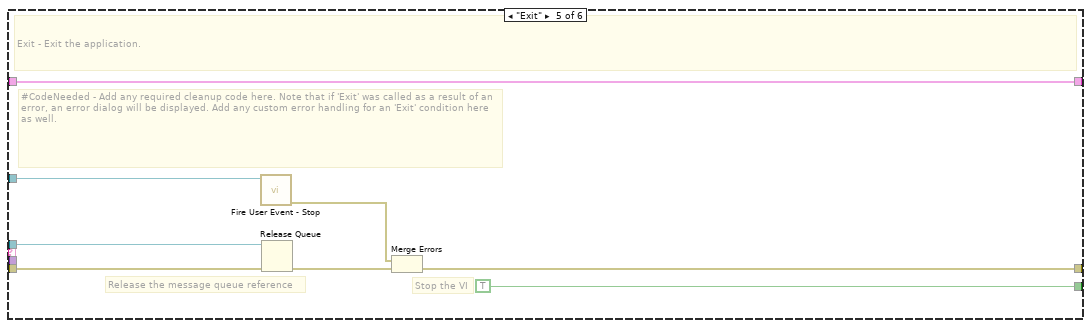
[diagram p11: hidden frame]
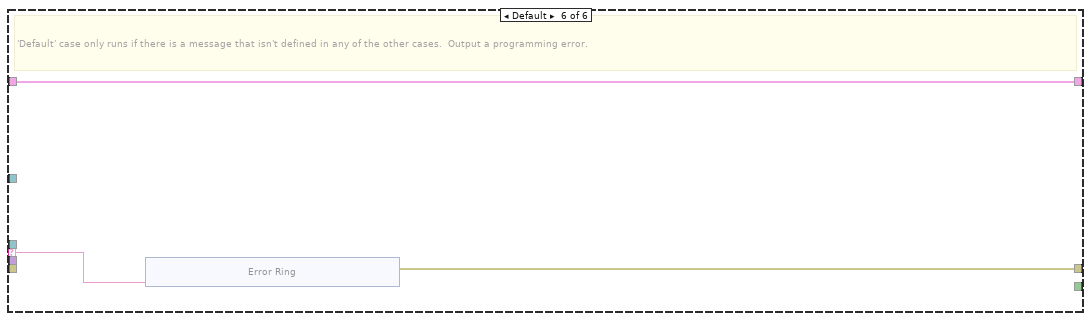
[diagram p12: hidden frame]
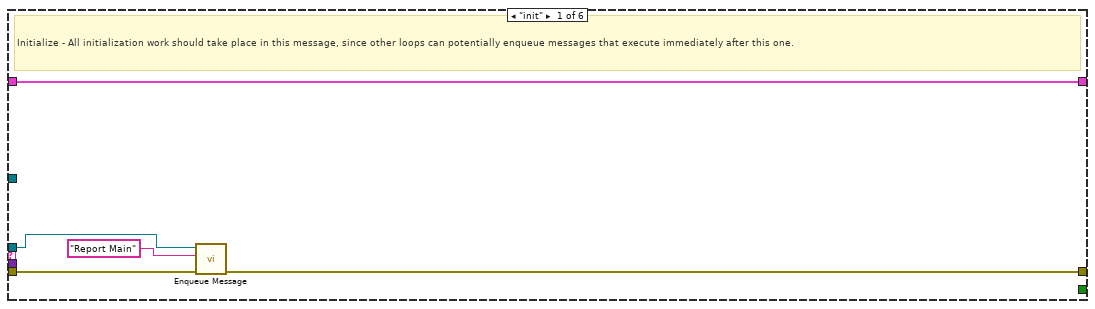
[diagram p14: hidden frame]
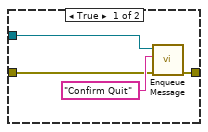
[diagram p15: hidden frame]
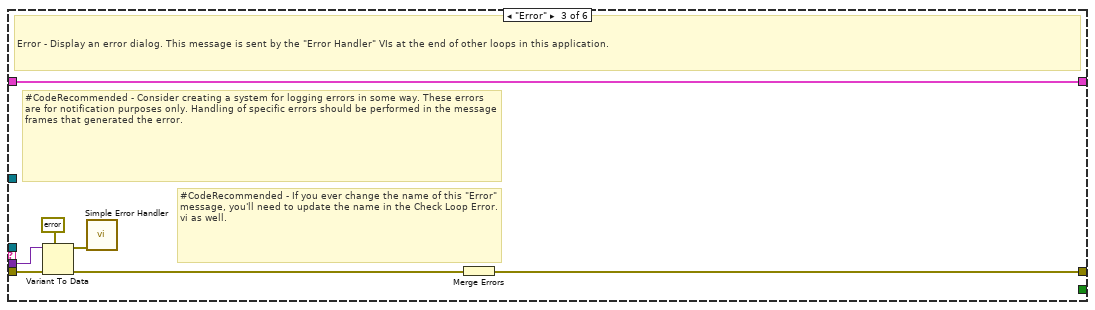
[diagram p16: hidden frame]
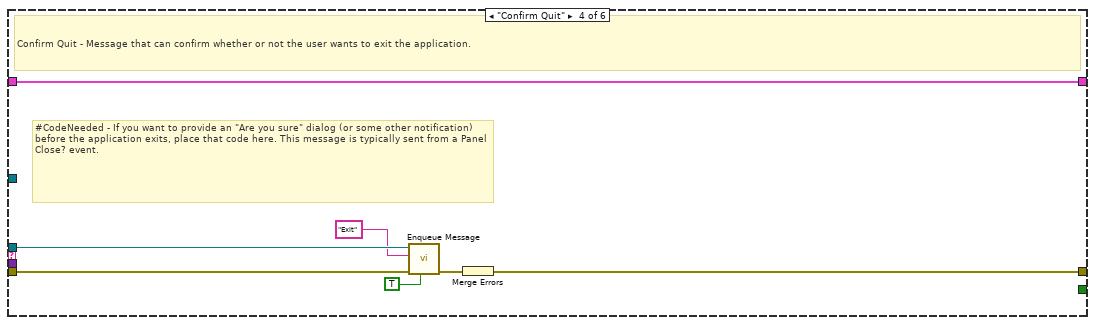
[diagram p17: hidden frame]
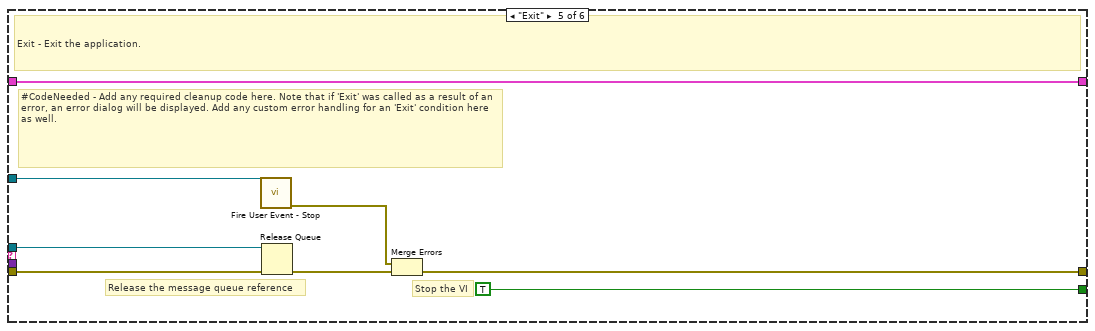
[diagram p18: hidden frame]
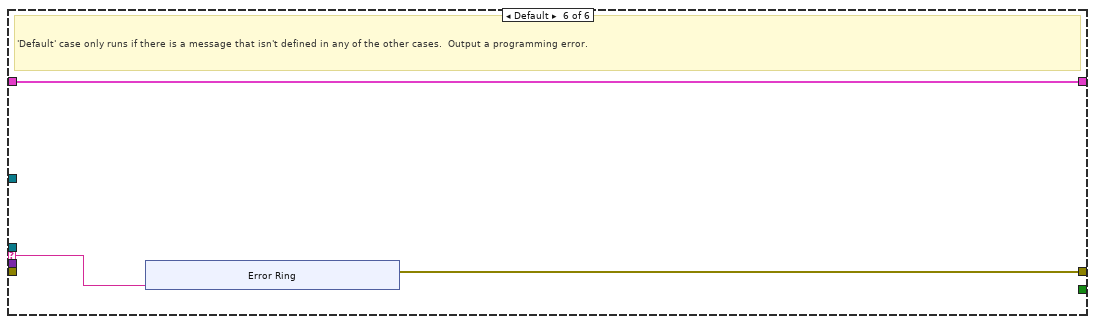
[diagram p19: hidden frame]
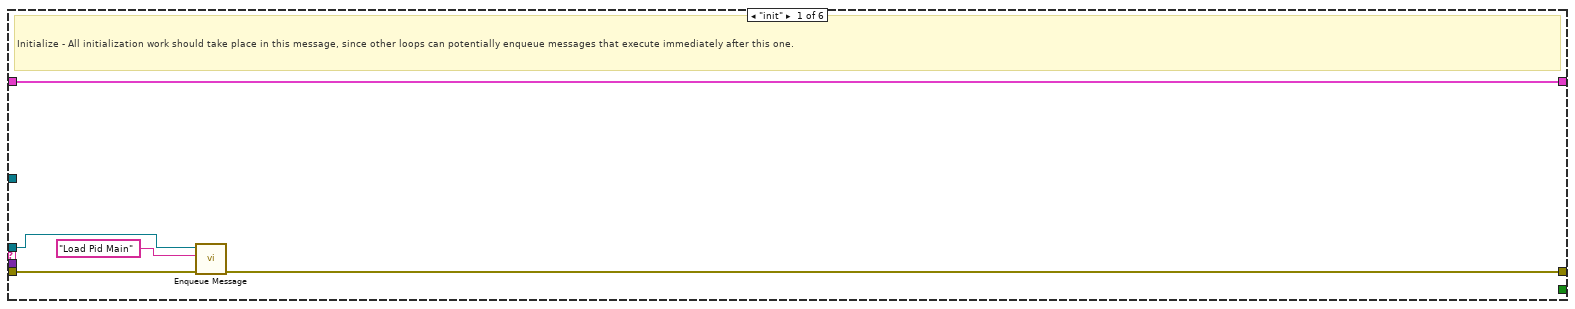
[diagram p20: hidden frame]
diagram:
  w7 = "" ("HEAVE OUT")
  w14 = -1  # max queue size
  (unwired) string[] ["PID DELAY (sec)", "Kp", "Ki", "Kd", "Deaadband", "pct_scale", "Init_step", "i_limit", "Max Step Limit", "i_limit", "Min_pos_limit", "Max_pos_limit", "Fine_tune_zone"]
  # "Start Test"
  n1 = flat-sequence {
    tunnel: [w67] -> w54
    tunnel: T12 {"Main Home Screen"={"GUI"=refnum, "Platform Settings"=refnum, "Configure"=refnum, "Home"=refnum, "EXIT"=refnum, "service 2"=refnum, "MainPage"=refnum, "Analysis"=refnum}, "Platform Settings"={"mm/s  Surge"=refnum, "Update Surge Speed"=refnum, "Drive Error"=refnum, "Disable Axis Jog Soft Limits"=refnum, "mm/s  Sway"=refnum, "Sway and Surge COM Status"=refnum, "Heave COM Status"=refnum, "Enable Platform"=refnum, "Surge Forward Main"=refnum, "Sway Right Main"=refnum, "Sway Left Main"=refnum, "Heave Down Main"=refnum, "Heave Up main"=refnum, "Update Sway Speed"=refnum, "Update Heave Speed"=refnum, "mm/s Heave"=refnum, "mm/sec"=refnum, "mm"=refnum, "Surge Backward Main"=refnum}, "Analysis Screen"={"Analysis Home"=refnum, "Surface Analysis"=refnum, "Imaging"=refnum, "Image Analysis"=refnum, "Post Analysis"=refnum}, "Config Screen"={"Select Load Head"=refnum, "Notes :"=refnum, "FILE"=refnum, "Sample ID :"=refnum, "Operator ID :"=refnum, "Operator Name :"=refnum, "Auto"=refnum}, "Motion Module"={"zNL"=refnum, "NL disp"=refnum, "Rotary Tab"=refnum, "Motion Direction:  3"=refnum, "E.Velocity 2"=refnum, "e.v/ssr 2"=refnum, "Enter Fixed E.Velocity 2"=refnum, "Enter Final SRR 2"=refnum, "Enter initial SRR 2"=refnum, "Enter Fixed SRR 2"=refnum, "Enter the Final E.Velocity (m/s) 2"=refnum, "Enter initial E.Velocity (m/s) 2"=refnum, "Final Speed (RPM) 3"=refnum, "Initial Speed (RPM) 2"=refnum, "Enter the Final Velocity (m/s) 3"=refnum, "Enter initial Velocity (m/s)  3"=refnum, "Ramp Up 2"=refnum, "TEST SELECTION"=refnum, "SPEED SELECTION : "=refnum, "Angular Oscillation Set"=refnum, "Traction"=refnum, "Step Speed"=refnum, "StepTable For Load-Speed"=refnum, "StepTable For Speed"=refnum, "Surge Forward MM"=refnum, "Surge Backward MM"=refnum, "M3 Image"=refnum, "String 39"=refnum, "Sway Left MM"=refnum, "Sway Right MM"=refnum, "Disable Axis Jog Soft Limits"=refnum, "mm"=refnum, "Heave Down MM"=refnum, "Heave Up MM"=refnum, "Wear Track Diameter (mm)"=refnum, "Set WTD"=refnum, "HomeScratch"=refnum, "HomeRot"=refnum, "PlaceModule"=refnum, "Enter the Angle (Deg)"=refnum, "Enter the Frequency (Hz)"=refnum, "Motion Mode:"=refnum, "LR Sway"=refnum, "Rot Hor"=refnum, "Scratch"=refnum, "LR Cam"=refnum, "MMBack"=refnum, "MMNext"=refnum, "Rot Ver"=refnum, "Rotary Module Selection"=refnum, "calculate rotary"=refnum, "SPEED SELECTION : rotary"=refnum, "Import 2"=refnum, "Save 2"=refnum, "File Path :  2"=refnum, "String 45"=refnum, "StepTable For Speed 3"=refnum, "Enter the Speed(mm/sec)"=refnum, "Enter the Speed(RPM)"=refnum}, "Environmental control"={"Humidity  Status  3"=refnum, "Low Temp  Status  2"=refnum, "TK4 status 2"=refnum, "Stage Temperature"=refnum, "Sample Temperature"=refnum, "Humidity (Amb)"=refnum, "Clear List"=refnum, "Add to list"=refnum, "Wear"=refnum, "Vibration"=refnum, "Humidity (Chamber)"=refnum, "Temperature (Chamber)"=refnum, "ECR "=refnum, "Temperature (Amb)"=refnum, "Microphone"=refnum, "Acoustic Emission 3"=refnum, "SNext"=refnum, "APBack"=refnum, "Enter the Temperature (°C):"=refnum, "Enter the Stage \nTemperature (°C):"=refnum, "Enter the Humidity (%Rh):"=refnum, "Low Temp"=refnum, "High Temp"=refnum, "Humidity"=refnum, "Sensors Picked"=refnum}, "About Screen"={"Password"=refnum, "Home Service"=refnum, "Advanced Setting"=refnum, "About Tab"=refnum, "ECR Port:"=refnum, "Ramp Port:"=refnum, "Installation/Replacement completed"=refnum, "Loahead"=refnum, "Heave and Surge COM Port:"=refnum, "Sway COM Port:"=refnum, "Temp Modbus:"=refnum, "Humidity Port:"=refnum, "Edit Gain Constants"=refnum, "Save Gain Constants"=refnum}, "Main Screen"={"Main Screen Tab"=refnum, "Angle and Frequency"=refnum, "Stroke (mm)"=refnum, "Angle (Deg)"=refnum, "Main Speed Tab"=refnum, "MTM MOTOR DISPLAY"=refnum, "Disc Speed (m/sec)"=refnum, "Ball Speed (m/sec)"=refnum, "Disc Speed (RPM)"=refnum, "Ball Speed (RPM)"=refnum, "SPEED TAB"=refnum, "Speed (m/sec)"=refnum, "Set Speed (m/sec)"=refnum, "Speed (RPM)"=refnum, "Set Speed"=refnum, "Time Tab"=refnum, "Time ( HH:MM:SS ) 2"=refnum, "Test Duration"=refnum, "Test Duration 4"=refnum, "TEST CYCLE"=refnum, "TOTAL CYCLES"=refnum, "Set Load (N)"=refnum, "Temp Tabs"=refnum, "Heater"=refnum, "TK4 status"=refnum, "ChamberTemp"=refnum, "SetTmp"=refnum, "Controller  Status"=refnum, "ChamberTemp 2"=refnum, "SetTmp 2"=refnum, "Controller  Status 2"=refnum, "ChamberTemp 3"=refnum, "SetTmp 3"=refnum, "Cooling"=refnum, "Load Communication"=refnum, "Ambient \nTemperature"=refnum, "HumCOMStatus"=refnum, "Ambient\n Humidity"=refnum, "Freq (Hz)"=refnum, "Load En"=refnum, "NLt"=refnum, "zNL 2"=refnum, "Humidity On"=refnum, "humidity disp"=refnum, "Set Humidity"=refnum, "NL disp 2"=refnum, "Humidity On 2"=refnum, "humidity disp 2"=refnum, "Set Humidity 2"=refnum, "NL disp 3"=refnum, "AppLoadSeq scratch"=refnum, "Stop Scratch"=refnum, "ClrLog"=refnum, "Trip Log"=refnum, "STOP"=refnum, "Start Test"=refnum, "Test status"=refnum, "AR Led"=refnum, "Data"=refnum, "Health"=refnum, "Sway COM Status"=refnum, "Heave COM Status"=refnum, "Grp Tab"=refnum, "Sub Graph"=refnum, "SD (mm)"=refnum, "Siliding distance Reset Graph"=refnum, "SDGp"=refnum, "Humidity Reset Graph"=refnum, "HumrGp"=refnum, "Acoustic Emission (mV)"=refnum, "Aqucostic Reset Graph"=refnum, "gACQUOS"=refnum, "ECR RESET"=refnum, "ECR"=refnum, "Temperature Reset"=refnum, "Acoustic Emission (mV) 2"=refnum, "Aqucostic Reset Graph 2"=refnum, "gACQUOS 2"=refnum, "ECR RESET 2"=refnum, "ECR 2"=refnum, "Temperature Reset 2"=refnum, "Temperature (deg c)"=refnum, "Speed Reset Graph"=refnum, "Speed Tab"=refnum, "MTM DISC  SPEED"=refnum, "MTM BALL SPEED"=refnum, "speed mm/sec"=refnum, "Hymidity"=refnum, "Humidity Disable trip"=refnum, "CoF Trip  2"=refnum, "Depth Trip"=refnum, "Weart Deapth"=refnum, "Depth Reset Graph"=refnum, "Weart"=refnum, "Depthz"=refnum, "Depth (µm)"=refnum, "WearGp"=refnum, "NL Trip 2"=refnum, "Load pid"=refnum, "Load Disable Trip"=refnum, "Load Reset Graph"=refnum, "NL Display 4"=refnum, "Main Chart 3"=refnum, "BACK"=refnum, "Depth Trip 2"=refnum, "COF TRIP "=refnum, "Friction Force (N)"=refnum, "FF Reset Graph"=refnum, "FF Disable Trip"=refnum, "FF TRIP"=refnum, "FF MAIN CHART"=refnum, "COF Disable Trip"=refnum, "COF Reset Graph"=refnum, "COF MAIN CHART"=refnum, "FF Tab"=refnum, "Start Test Temp"=refnum}, "Loading"={"Indentation"=refnum, "Reference Sample"=refnum, "Load Cell Communication Slide"=refnum, "com 3"=refnum, "com"=refnum, "DecaForce COM Status"=refnum, "Update"=refnum, "Clear 3"=refnum, "seq"=refnum, "Stribeck table"=refnum, "Stribeck Table  For loading"=refnum, "Loading Mode"=refnum, "Enter the Final Load (N)"=refnum, "Enter the CoF Trip"=refnum, "Enter the Friction Force Trip"=refnum, "Enter the Normal load Trip"=refnum, "Enter the Load  (N)"=refnum, "KiloForce"=refnum, "DecaForce "=refnum, "MicroForce"=refnum, "LHBack"=refnum, "LHNext"=refnum, "Enter the Loading Rate (N/min)"=refnum, "Message"=refnum, "Warning 2"=refnum, "SSP 0.75"=refnum, "SSP 0.5"=refnum, "SSP 0.3"=refnum, "Warning"=refnum, "gui GIF"=refnum, "Communication is established"=refnum, "AppLoad 4"=refnum, "Multipoint"=refnum, "Load Selection"=refnum}, "PID"={"Ramp MulFac"=refnum, "pulses LoadDiffRamp(2..10)"=refnum, "PulseControlRamp(diff<=3N)"=refnum, "SetLoadDeadband(%) Load(0-10N)"=refnum, "PID gains out delay (microForce)"=refnum, "Ramp"=refnum, "Gain 2"=refnum, "pulses LoadDiff(2..10)"=refnum, "pulses LoadDiff(11..50)"=refnum, "PulseControl(diff<=3N)"=refnum, "SetLoadDeadband(%)  2"=refnum, "Dummy Run"=refnum, "Vertical load (N)"=refnum, "AutoTune"=refnum, "Offset 3 "=refnum, "apply load"=refnum, "Offset  3"=refnum, "apply load 2"=refnum, "Enter ByPass Load"=refnum, "reinit 3"=refnum, "output range delay"=refnum, "PID gains out delay"=refnum, "Bypass Load"=refnum, "pulsesSent"=refnum, "pulses "=refnum, "actpid"=refnum, "gFF Rot"=refnum, "pulses LoadDiff(21..1000)"=refnum, "Delay"=refnum, "deadband"=refnum}, "Config Parameters"={"Tab Control 3"=refnum, "Tab Control 19"=refnum, "SAMPLES"=refnum, "Re-initilaize"=refnum, "Filter ON/OFF"=refnum, "TracHomeSurgeOffsetCounts 10MM"=refnum, "TracHomeSwayOffsetCounts 10MM"=refnum, "Acoustic Emission:"=refnum, "Apply Filter (FF)"=refnum, "Filter% 2"=refnum, "Apply Filter (Load)"=refnum, "Filter% "=refnum, "Sway distance (mm)"=refnum, "Surge distance (mm)"=refnum, "DataSavingLoopDelay(ms)"=refnum, "SAVE 2"=refnum, "Enter Distance"=refnum, "Sway Counts:"=refnum, "Distance (mm): 3"=refnum, "Surge Counts:"=refnum, "Distance (mm): 2"=refnum, "Distance (mm):"=refnum, "Heave Counts:"=refnum, "LRMHomeSurgeOffsetCounts"=refnum, "LRMHomeSwayOffsetCounts"=refnum, "TracHomeSurgeOffsetCounts 20MM"=refnum, "TracHomeSwayOffsetCounts 20MM"=refnum, "RotHomeSwayOffsetCounts"=refnum, "RotHomeSurgeOffsetCounts"=refnum, "Heave distance"=refnum, "Zmm"=refnum, "Heave Pulses/mm"=refnum, "Surge Pulses/mm"=refnum, "Sway Pulses/mm"=refnum, "Heave Pitch"=refnum, "Surge Pitch"=refnum, "Sway Pitch"=refnum, "Heave PPR"=refnum, "Surge PPR"=refnum, "Sway PPR"=refnum, "Tab Control 5"=refnum, "Tab Control 14"=refnum, "Tab Control 26"=refnum, "AE"=refnum, "Heave Loop Delay"=refnum, "Heave PID Speed"=refnum, "Surge Jog Speed"=refnum, "Heave Jog Speed"=refnum}, "Loading Com Port"={"ClearAll"=refnum, "Mz(Nm)"=refnum, "My(Nm)"=refnum, "Mx(Nm)"=refnum, "Save Dwell"=refnum, "Mx "=refnum, "My "=refnum, "Mz"=refnum, "Fx(N)"=refnum, "Fy(N)"=refnum, "Fz(N)"=refnum, "ZeroAll"=refnum, "Acq Delay (ms)"=refnum, "Burst Delay (ms)"=refnum, "model"=refnum, "SN"=refnum, "FFx(N)"=refnum, "Sensor IP"=refnum, "Port"=refnum, "FFy(N)"=refnum, "Load(N)"=refnum, "delete Handle"=refnum, "Create Handle"=refnum, "ft_data"=refnum, "ft_range"=refnum, "ft_data 2"=refnum, "stop 6"=refnum, "running_flag"=refnum, "ft_udp_handle"=refnum, "get-data-return"=refnum, "get-range-return"=refnum, "zero-return"=refnum, "filter-return"=refnum, "initial-return"=refnum, "deleteHandle-result"=refnum, "Load Cell Temp"=refnum}, "Heave AND Surge"={"SURGE POSE"=refnum, "error out Read"=refnum, "HEAVE POSE"=refnum, "State"=refnum, "Homed"=refnum, "Sequence ID"=refnum, "error out Write"=refnum, "faultCode"=refnum, "Ack ID"=refnum, "SPEED"=refnum, "Distance"=refnum, "Mode Command"=refnum, "Heave and Surge Read"=refnum, "Read Heave Temp"=refnum, "Spare 15"=refnum, "Spare 14"=refnum, "Spare 13"=refnum, "Spare 12"=refnum, "Spare 11"=refnum, "Spare 10"=refnum, "Spare 9"=refnum, "Spare 8"=refnum, "Spare 7"=refnum, "Spare 6"=refnum, "Spare 5"=refnum, "Spare 4"=refnum, "Spare 2"=refnum, "Spare 1"=refnum, "Node Id"=refnum, "Spare 3"=refnum, "SPARE 4"=refnum, "SPARE 3"=refnum, "SPARE 2"=refnum, "SPARE 1"=refnum, "fwMajor"=refnum, "fwMinor"=refnum, "Manual Write"=refnum, "Heave and Surge Write"=refnum}, "New PID LOGIC"={"Fine Tune Zone"=refnum, "PID SDelay"=refnum, "Max_pos_limit"=refnum, "Min_pos_limit"=refnum, "i_limit"=refnum, "pct_scale"=refnum, "Deadband"=refnum, "Kd"=refnum, "Ki"=refnum, "Kp"=refnum, "Current Position"=refnum, "Set Load"=refnum, "Current Load"=refnum, "Pulse delta"=refnum, "Init Step"=refnum, "Max Step Linit"=refnum}} ("Data Cluster") -> [w66]
    tunnel: w54 -> [w96]
    tunnel: [w76] -> w53
    tunnel: w53 -> [w103]
    tunnel: [w97] -> w52
    tunnel: w52 -> [w112]
    tunnel: [w111] -> w51
    tunnel: w51 -> [w148]
    tunnel: [w147] -> w49
    tunnel: w49 -> [w209]
    tunnel: [w208] -> w48
    tunnel: w48 -> [w236]
    tunnel: [w235] -> w47
    tunnel: w47 -> [w252]
    tunnel: [w251] -> w46
    tunnel: w46 -> [w357]
    tunnel: [w356] -> w21
    tunnel: w21 -> [w387]
    tunnel: [w386] -> w20
    tunnel: w20 -> [w437]
    tunnel: [w436] -> w19
    tunnel: w19 -> [w474]
    tunnel: [w473] -> w18
    tunnel: w18 -> [w514]
    tunnel: [w513] -> w16
    tunnel: [w531] -> w6
    tunnel: w16 -> [w532]
    frame #0 {
      n2 = control-ref of="GUI"() -> (w75:refnum<vi>)
      n3 = control-ref of="MainPage"() -> (w69:refnum<vi>)
      n4 = control-ref of="Platform Settings"() -> (w74:refnum<vi>)
      n5 = control-ref of="Configure"() -> (w73:refnum<vi>)
      n6 = control-ref of="Home"() -> (w72:refnum<vi>)
      n7 = control-ref of="EXIT"() -> (w71:refnum<vi>)
      n8 = control-ref of="service 2"() -> (w70:refnum<vi>)
      n9 = control-ref of="Analysis"() -> (w68:refnum<vi>)
      n10 = Bundle By Name(cluster=w66, "Main Home Screen.GUI"=w75, "Main Home Screen.Platform Settings"=w74, "Main Home Screen.Configure"=w73, "Main Home Screen.Home"=w72, "Main Home Screen.EXIT"=w71, "Main Home Screen.service 2"=w70, "Main Home Screen.MainPage"=w69, "Main Home Screen.Analysis"=w68) -> (w67:T12)
    }
    frame #1 {
      n11 = control-ref of="Sway Right Main"() -> (w86:refnum<vi>)
      n12 = control-ref of="Sway Left Main"() -> (w85:refnum<vi>)
      n13 = control-ref of="Heave Down Main"() -> (w84:refnum<vi>)
      n14 = control-ref of="Heave Up main"() -> (w83:refnum<vi>)
      n15 = control-ref of="Update Sway Speed"() -> (w82:refnum<vi>)
      n16 = control-ref of="Update Heave Speed"() -> (w81:refnum<vi>)
      n17 = control-ref of="Surge Backward Main"() -> (w77:refnum<vi>)
      n18 = control-ref of="Update Surge Speed"() -> (w94:refnum<vi>)
      n19 = control-ref of="Disable Axis Jog Soft Limits"() -> (w92:refnum<vi>)
      n20 = control-ref of="Sway and Surge COM Status"() -> (w90:refnum<vi>)
      n21 = control-ref of="Heave COM Status"() -> (w89:refnum<vi>)
      n22 = control-ref of="Enable Platform"() -> (w88:refnum<vi>)
      n23 = control-ref of="Surge Forward Main"() -> (w87:refnum<vi>)
      n24 = control-ref of="mm/s Heave"() -> (w80:refnum<vi>)
      n25 = control-ref of="mm/sec"() -> (w79:refnum<vi>)
      n26 = control-ref of="mm"() -> (w78:refnum<vi>)
      n27 = control-ref of="mm/s  Surge"() -> (w95:refnum<vi>)
      n28 = control-ref of="mm/s  Sway"() -> (w91:refnum<vi>)
      n29 = control-ref of="Drive Error"() -> (w93:refnum<vi>)
      n30 = Bundle By Name(cluster=w96, "Platform Settings.mm/s  Surge"=w95, "Platform Settings.Update Surge Speed"=w94, "Platform Settings.Drive Error"=w93, "Platform Settings.Disable Axis Jog Soft Limits"=w92, "Platform Settings.mm/s  Sway"=w91, "Platform Settings.Sway and Surge COM Status"=w90, "Platform Settings.Heave COM Status"=w89, "Platform Settings.Enable Platform"=w88, "Platform Settings.Surge Forward Main"=w87, "Platform Settings.Sway Right Main"=w86, "Platform Settings.Sway Left Main"=w85, "Platform Settings.Heave Down Main"=w84, "Platform Settings.Heave Up main"=w83, "Platform Settings.Update Sway Speed"=w82, "Platform Settings.Update Heave Speed"=w81, "Platform Settings.mm/s Heave"=w80, "Platform Settings.mm/sec"=w79, "Platform Settings.mm"=w78, "Platform Settings.Surge Backward Main"=w77) -> (w76:T12)
    }
    frame #2 {
      n31 = control-ref of="Analysis Home"() -> (w102:refnum<vi>)
      n32 = control-ref of="Surface Analysis"() -> (w101:refnum<vi>)
      n33 = control-ref of="Imaging"() -> (w100:refnum<vi>)
      n34 = control-ref of="Image Analysis"() -> (w99:refnum<vi>)
      n35 = control-ref of="Post Analysis"() -> (w98:refnum<vi>)
      n36 = Bundle By Name(cluster=w103, "Analysis Screen.Analysis Home"=w102, "Analysis Screen.Surface Analysis"=w101, "Analysis Screen.Imaging"=w100, "Analysis Screen.Image Analysis"=w99, "Analysis Screen.Post Analysis"=w98) -> (w97:T12)
    }
    frame #3 {
      n37 = control-ref of="Select Load Head"() -> (w110:refnum<vi>)
      n38 = control-ref of="Auto"() -> (w104:refnum<vi>)
      n39 = control-ref of="Notes :"() -> (w109:refnum<vi>)
      n40 = control-ref of="FILE"() -> (w108:refnum<vi>)
      n41 = control-ref of="Sample ID :"() -> (w107:refnum<vi>)
      n42 = control-ref of="Operator ID :"() -> (w106:refnum<vi>)
      n43 = control-ref of="Operator Name :"() -> (w105:refnum<vi>)
      n44 = Bundle By Name(cluster=w112, "Config Screen.Select Load Head"=w110, "Config Screen.Notes :"=w109, "Config Screen.FILE"=w108, "Config Screen.Sample ID :"=w107, "Config Screen.Operator ID :"=w106, "Config Screen.Operator Name :"=w105, "Config Screen.Auto"=w104) -> (w111:T12)
    }
    frame #4 {
      n45 = control-ref of="Warning"() -> (w140:refnum<vi>)
      n46 = control-ref of="gui GIF"() -> (w139:refnum<vi>)
      n47 = control-ref of="Load Selection"() -> (w113:refnum<vi>)
      n48 = control-ref of="Warning 2"() -> (w144:refnum<vi>)
      n49 = control-ref of="SSP 0.75"() -> (w143:refnum<vi>)
      n50 = control-ref of="SSP 0.5"() -> (w142:refnum<vi>)
      n51 = control-ref of="SSP 0.3"() -> (w141:refnum<vi>)
      n52 = control-ref of="Communication is established"() -> (w138:refnum<vi>)
      n53 = control-ref of="AppLoad 4"() -> (w137:refnum<vi>)
      n54 = control-ref of="Multipoint"() -> (w136:refnum<vi>)
      n55 = control-ref of="com 3"() -> (w132:refnum<vi>)
      n56 = control-ref of="com"() -> (w131:refnum<vi>)
      n57 = control-ref of="DecaForce COM Status"() -> (w130:refnum<vi>)
      n58 = control-ref of="Update"() -> (w129:refnum<vi>)
      n59 = control-ref of="Clear 3"() -> (w128:refnum<vi>)
      n60 = control-ref of="seq"() -> (w127:refnum<vi>)
      n61 = control-ref of="Stribeck table"() -> (w126:refnum<vi>)
      n62 = control-ref of="KiloForce"() -> (w118:refnum<vi>)
      n63 = control-ref of="DecaForce"() -> (w117:refnum<vi>)
      n64 = control-ref of="MicroForce"() -> (w116:refnum<vi>)
      n65 = control-ref of="LHBack"() -> (w115:refnum<vi>)
      n66 = control-ref of="LHNext"() -> (w114:refnum<vi>)
      n67 = control-ref of="Enter the Loading Rate (N/min)"() -> (w146:refnum<vi>)
      n68 = control-ref of="Enter the Final Load (N)"() -> (w123:refnum<vi>)
      n69 = control-ref of="Enter the CoF Trip"() -> (w122:refnum<vi>)
      n70 = control-ref of="Enter the Friction Force Trip"() -> (w121:refnum<vi>)
      n71 = control-ref of="Enter the Normal load Trip"() -> (w120:refnum<vi>)
      n72 = control-ref of="Enter the Load  (N)"() -> (w119:refnum<vi>)
      n73 = control-ref of="Message"() -> (w145:refnum<vi>)
      n74 = control-ref of="Indentation"() -> (w135:refnum<vi>)
      n75 = control-ref of="Stribeck Table  For loading"() -> (w125:refnum<vi>)
      n76 = control-ref of="Reference Sample"() -> (w134:refnum<vi>)
      n77 = control-ref of="Load Cell Communication Slide"() -> (w133:refnum<vi>)
      n78 = control-ref of="Loading Mode"() -> (w124:refnum<vi>)
      n79 = Bundle By Name(cluster=w148, "Loading.Enter the Loading Rate (N/min)"=w146, "Loading.Message"=w145, "Loading.Warning 2"=w144, "Loading.SSP 0.75"=w143, "Loading.SSP 0.5"=w142, "Loading.SSP 0.3"=w141, "Loading.Warning"=w140, "Loading.gui GIF"=w139, "Loading.Communication is established"=w138, "Loading.AppLoad 4"=w137, "Loading.Multipoint"=w136, "Loading.Indentation"=w135, "Loading.Reference Sample"=w134, "Loading.Load Cell Communication Slide"=w133, "Loading.com 3"=w132, "Loading.com"=w131, "Loading.DecaForce COM Status"=w130, "Loading.Update"=w129, "Loading.Clear 3"=w128, "Loading.seq"=w127, "Loading.Stribeck table"=w126, "Loading.Stribeck Table  For loading"=w125, "Loading.Loading Mode"=w124, "Loading.Enter the Final Load (N)"=w123, "Loading.Enter the CoF Trip"=w122, "Loading.Enter the Friction Force Trip"=w121, "Loading.Enter the Normal load Trip"=w120, "Loading.Enter the Load  (N)"=w119, "Loading.KiloForce"=w118, "Loading.DecaForce"=w117, "Loading.MicroForce"=w116, "Loading.LHBack"=w115, "Loading.LHNext"=w114, "Loading.Load Selection"=w113) -> (w147:T12)
    }
    frame #5 {
      n80 = control-ref of="TEST SELECTION"() -> (w190:refnum<vi>)
      n81 = control-ref of="SPEED SELECTION :"() -> (w189:refnum<vi>)
      n82 = control-ref of="SPEED SELECTION : rotary"() -> (w156:refnum<vi>)
      n83 = control-ref of="Rotary Tab"() -> (w205:refnum<vi>)
      n84 = control-ref of="e.v/ssr 2"() -> (w202:refnum<vi>)
      n85 = control-ref of="Step Speed"() -> (w186:refnum<vi>)
      n86 = control-ref of="M3 Image"() -> (w181:refnum<vi>)
      n87 = control-ref of="Rotary Module Selection"() -> (w158:refnum<vi>)
      n88 = control-ref of="zNL"() -> (w207:refnum<vi>)
      n89 = control-ref of="E.Velocity 2"() -> (w203:refnum<vi>)
      n90 = control-ref of="Ramp Up 2"() -> (w191:refnum<vi>)
      n91 = control-ref of="Angular Oscillation Set"() -> (w188:refnum<vi>)
      n92 = control-ref of="Traction"() -> (w187:refnum<vi>)
      n93 = control-ref of="Surge Forward MM"() -> (w183:refnum<vi>)
      n94 = control-ref of="Surge Backward MM"() -> (w182:refnum<vi>)
      n95 = control-ref of="Sway Left MM"() -> (w179:refnum<vi>)
      n96 = control-ref of="Sway Right MM"() -> (w178:refnum<vi>)
      n97 = control-ref of="Disable Axis Jog Soft Limits"() -> (w177:refnum<vi>)
      n98 = control-ref of="Heave Down MM"() -> (w175:refnum<vi>)
      n99 = control-ref of="Heave Up MM"() -> (w174:refnum<vi>)
      n100 = control-ref of="Set WTD"() -> (w172:refnum<vi>)
      n101 = control-ref of="HomeScratch"() -> (w171:refnum<vi>)
      n102 = control-ref of="HomeRot"() -> (w170:refnum<vi>)
      n103 = control-ref of="PlaceModule"() -> (w169:refnum<vi>)
      n104 = control-ref of="LR Sway"() -> (w165:refnum<vi>)
      n105 = control-ref of="Rot Hor"() -> (w164:refnum<vi>)
      n106 = control-ref of="Scratch"() -> (w163:refnum<vi>)
      n107 = control-ref of="LR Cam"() -> (w162:refnum<vi>)
      n108 = control-ref of="MMBack"() -> (w161:refnum<vi>)
      n109 = control-ref of="MMNext"() -> (w160:refnum<vi>)
      n110 = control-ref of="Rot Ver"() -> (w159:refnum<vi>)
      n111 = control-ref of="calculate rotary"() -> (w157:refnum<vi>)
      n112 = control-ref of="Import 2"() -> (w155:refnum<vi>)
      n113 = control-ref of="Save 2"() -> (w154:refnum<vi>)
      n114 = control-ref of="NL disp"() -> (w206:refnum<vi>)
      n115 = control-ref of="Enter Fixed E.Velocity 2"() -> (w201:refnum<vi>)
      n116 = control-ref of="Enter Final SRR 2"() -> (w200:refnum<vi>)
      n117 = control-ref of="Enter initial SRR 2"() -> (w199:refnum<vi>)
      n118 = control-ref of="Enter Fixed SRR 2"() -> (w198:refnum<vi>)
      n119 = control-ref of="Enter the Final E.Velocity (m/s) 2"() -> (w197:refnum<vi>)
      n120 = control-ref of="Enter initial E.Velocity (m/s) 2"() -> (w196:refnum<vi>)
      n121 = control-ref of="Final Speed (RPM) 3"() -> (w195:refnum<vi>)
      n122 = control-ref of="Initial Speed (RPM) 2"() -> (w194:refnum<vi>)
      n123 = control-ref of="Enter the Final Velocity (m/s) 3"() -> (w193:refnum<vi>)
      n124 = control-ref of="Enter initial Velocity (m/s)  3"() -> (w192:refnum<vi>)
      n125 = control-ref of="mm"() -> (w176:refnum<vi>)
      n126 = control-ref of="Wear Track Diameter (mm)"() -> (w173:refnum<vi>)
      n127 = control-ref of="Enter the Angle (Deg)"() -> (w168:refnum<vi>)
      n128 = control-ref of="Enter the Frequency (Hz)"() -> (w167:refnum<vi>)
      n129 = control-ref of="Enter the Speed(mm/sec)"() -> (w150:refnum<vi>)
      n130 = control-ref of="Enter the Speed(RPM)"() -> (w149:refnum<vi>)
      n131 = control-ref of="String 39"() -> (w180:refnum<vi>)
      n132 = control-ref of="String 45"() -> (w152:refnum<vi>)
      n133 = control-ref of="StepTable For Load-Speed"() -> (w185:refnum<vi>)
      n134 = control-ref of="StepTable For Speed"() -> (w184:refnum<vi>)
      n135 = control-ref of="Motion Direction:  3"() -> (w204:refnum<vi>)
      n136 = control-ref of="Motion Mode:"() -> (w166:refnum<vi>)
      n137 = control-ref of="StepTable For Speed 3"() -> (w151:refnum<vi>)
      n138 = control-ref of="File Path :  2"() -> (w153:refnum<vi>)
      n139 = Bundle By Name(cluster=w209, "Motion Module.zNL"=w207, "Motion Module.NL disp"=w206, "Motion Module.Rotary Tab"=w205, "Motion Module.Motion Direction:  3"=w204, "Motion Module.E.Velocity 2"=w203, "Motion Module.e.v/ssr 2"=w202, "Motion Module.Enter Fixed E.Velocity 2"=w201, "Motion Module.Enter Final SRR 2"=w200, "Motion Module.Enter initial SRR 2"=w199, "Motion Module.Enter Fixed SRR 2"=w198, "Motion Module.Enter the Final E.Velocity (m/s) 2"=w197, "Motion Module.Enter initial E.Velocity (m/s) 2"=w196, "Motion Module.Final Speed (RPM) 3"=w195, "Motion Module.Initial Speed (RPM) 2"=w194, "Motion Module.Enter the Final Velocity (m/s) 3"=w193, "Motion Module.Enter initial Velocity (m/s)  3"=w192, "Motion Module.Ramp Up 2"=w191, "Motion Module.TEST SELECTION"=w190, "Motion Module.SPEED SELECTION :"=w189, "Motion Module.Angular Oscillation Set"=w188, "Motion Module.Traction"=w187, "Motion Module.Step Speed"=w186, "Motion Module.StepTable For Load-Speed"=w185, "Motion Module.StepTable For Speed"=w184, "Motion Module.Surge Forward MM"=w183, "Motion Module.Surge Backward MM"=w182, "Motion Module.M3 Image"=w181, "Motion Module.String 39"=w180, "Motion Module.Sway Left MM"=w179, "Motion Module.Sway Right MM"=w178, "Motion Module.Disable Axis Jog Soft Limits"=w177, "Motion Module.mm"=w176, "Motion Module.Heave Down MM"=w175, "Motion Module.Heave Up MM"=w174, "Motion Module.Wear Track Diameter (mm)"=w173, "Motion Module.Set WTD"=w172, "Motion Module.HomeScratch"=w171, "Motion Module.HomeRot"=w170, "Motion Module.PlaceModule"=w169, "Motion Module.Enter the Angle (Deg)"=w168, "Motion Module.Enter the Frequency (Hz)"=w167, "Motion Module.Motion Mode:"=w166, "Motion Module.LR Sway"=w165, "Motion Module.Rot Hor"=w164, "Motion Module.Scratch"=w163, "Motion Module.LR Cam"=w162, "Motion Module.MMBack"=w161, "Motion Module.MMNext"=w160, "Motion Module.Rot Ver"=w159, "Motion Module.Rotary Module Selection"=w158, "Motion Module.calculate rotary"=w157, "Motion Module.SPEED SELECTION : rotary"=w156, "Motion Module.Import 2"=w155, "Motion Module.Save 2"=w154, "Motion Module.File Path :  2"=w153, "Motion Module.String 45"=w152, "Motion Module.StepTable For Speed 3"=w151, "Motion Module.Enter the Speed(mm/sec)"=w150, "Motion Module.Enter the Speed(RPM)"=w149) -> (w208:T12)
    }
    frame #6 {
      n140 = control-ref of="Add to list"() -> (w227:refnum<vi>)
      n141 = control-ref of="Wear"() -> (w226:refnum<vi>)
      n142 = control-ref of="Vibration"() -> (w225:refnum<vi>)
      n143 = control-ref of="Humidity (Chamber)"() -> (w224:refnum<vi>)
      n144 = control-ref of="Temperature (Chamber)"() -> (w223:refnum<vi>)
      n145 = control-ref of="ECR"() -> (w222:refnum<vi>)
      n146 = control-ref of="Temperature (Amb)"() -> (w221:refnum<vi>)
      n147 = control-ref of="Microphone"() -> (w220:refnum<vi>)
      n148 = control-ref of="Acoustic Emission 3"() -> (w219:refnum<vi>)
      n149 = control-ref of="SNext"() -> (w218:refnum<vi>)
      n150 = control-ref of="APBack"() -> (w217:refnum<vi>)
      n151 = control-ref of="Low Temp"() -> (w213:refnum<vi>)
      n152 = control-ref of="High Temp"() -> (w212:refnum<vi>)
      n153 = control-ref of="Humidity"() -> (w211:refnum<vi>)
      n154 = control-ref of="Humidity  Status  3"() -> (w234:refnum<vi>)
      n155 = control-ref of="Low Temp  Status  2"() -> (w233:refnum<vi>)
      n156 = control-ref of="TK4 status 2"() -> (w232:refnum<vi>)
      n157 = control-ref of="Humidity (Amb)"() -> (w229:refnum<vi>)
      n158 = control-ref of="Clear List"() -> (w228:refnum<vi>)
      n159 = control-ref of="Enter the Temperature (°C):"() -> (w216:refnum<vi>)
      n160 = control-ref of="Enter the Stage \nTemperature (°C):"() -> (w215:refnum<vi>)
      n161 = control-ref of="Enter the Humidity (%Rh):"() -> (w214:refnum<vi>)
      n162 = control-ref of="Sensors Picked"() -> (w210:refnum<vi>)
      n163 = control-ref of="Stage Temperature"() -> (w231:refnum<vi>)
      n164 = control-ref of="Sample Temperature"() -> (w230:refnum<vi>)
      n165 = Bundle By Name(cluster=w236, "Environmental control.Humidity  Status  3"=w234, "Environmental control.Low Temp  Status  2"=w233, "Environmental control.TK4 status 2"=w232, "Environmental control.Stage Temperature"=w231, "Environmental control.Sample Temperature"=w230, "Environmental control.Humidity (Amb)"=w229, "Environmental control.Clear List"=w228, "Environmental control.Add to list"=w227, "Environmental control.Wear"=w226, "Environmental control.Vibration"=w225, "Environmental control.Humidity (Chamber)"=w224, "Environmental control.Temperature (Chamber)"=w223, "Environmental control.ECR"=w222, "Environmental control.Temperature (Amb)"=w221, "Environmental control.Microphone"=w220, "Environmental control.Acoustic Emission 3"=w219, "Environmental control.SNext"=w218, "Environmental control.APBack"=w217, "Environmental control.Enter the Temperature (°C):"=w216, "Environmental control.Enter the Stage \nTemperature (°C):"=w215, "Environmental control.Enter the Humidity (%Rh):"=w214, "Environmental control.Low Temp"=w213, "Environmental control.High Temp"=w212, "Environmental control.Humidity"=w211, "Environmental control.Sensors Picked"=w210) -> (w235:T12)
    }
    frame #7 {
      n166 = control-ref of="ECR Port:"() -> (w246:refnum<vi>)
      n167 = control-ref of="Ramp Port:"() -> (w245:refnum<vi>)
      n168 = control-ref of="Heave and Surge COM Port:"() -> (w242:refnum<vi>)
      n169 = control-ref of="Sway COM Port:"() -> (w241:refnum<vi>)
      n170 = control-ref of="Temp Modbus:"() -> (w240:refnum<vi>)
      n171 = control-ref of="Humidity Port:"() -> (w239:refnum<vi>)
      n172 = control-ref of="About Tab"() -> (w247:refnum<vi>)
      n173 = control-ref of="Home Service"() -> (w249:refnum<vi>)
      n174 = control-ref of="Advanced Setting"() -> (w248:refnum<vi>)
      n175 = control-ref of="Installation/Replacement completed"() -> (w244:refnum<vi>)
      n176 = control-ref of="Loahead"() -> (w243:refnum<vi>)
      n177 = control-ref of="Edit Gain Constants"() -> (w238:refnum<vi>)
      n178 = control-ref of="Save Gain Constants"() -> (w237:refnum<vi>)
      n179 = control-ref of="Password"() -> (w250:refnum<vi>)
      n180 = Bundle By Name(cluster=w252, "About Screen.Password"=w250, "About Screen.Home Service"=w249, "About Screen.Advanced Setting"=w248, "About Screen.About Tab"=w247, "About Screen.ECR Port:"=w246, "About Screen.Ramp Port:"=w245, "About Screen.Installation/Replacement completed"=w244, "About Screen.Loahead"=w243, "About Screen.Heave and Surge COM Port:"=w242, "About Screen.Sway COM Port:"=w241, "About Screen.Temp Modbus:"=w240, "About Screen.Humidity Port:"=w239, "About Screen.Edit Gain Constants"=w238, "About Screen.Save Gain Constants"=w237) -> (w251:T12)
    }
    frame #8 {
      n181 = control-ref of="SDGp"() -> (w296:refnum<vi>)
      n182 = control-ref of="HumrGp"() -> (w294:refnum<vi>)
      n183 = control-ref of="gACQUOS"() -> (w291:refnum<vi>)
      n184 = control-ref of="ECR"() -> (w289:refnum<vi>)
      n185 = control-ref of="Temperature (deg c)"() -> (w287:refnum<vi>)
      n186 = control-ref of="MTM DISC  SPEED"() -> (w284:refnum<vi>)
      n187 = control-ref of="MTM BALL SPEED"() -> (w283:refnum<vi>)
      n188 = control-ref of="speed mm/sec"() -> (w282:refnum<vi>)
      n189 = control-ref of="WearGp"() -> (w272:refnum<vi>)
      n190 = control-ref of="Main Chart 3"() -> (w266:refnum<vi>)
      n191 = control-ref of="FF MAIN CHART"() -> (w258:refnum<vi>)
      n192 = control-ref of="COF MAIN CHART"() -> (w255:refnum<vi>)
      n193 = control-ref of="Main Screen Tab"() -> (w355:refnum<vi>)
      n194 = control-ref of="Angle and Frequency"() -> (w354:refnum<vi>)
      n195 = control-ref of="Main Speed Tab"() -> (w351:refnum<vi>)
      n196 = control-ref of="MTM MOTOR DISPLAY"() -> (w350:refnum<vi>)
      n197 = control-ref of="SPEED TAB"() -> (w345:refnum<vi>)
      n198 = control-ref of="Time Tab"() -> (w340:refnum<vi>)
      n199 = control-ref of="Temp Tabs"() -> (w333:refnum<vi>)
      n200 = control-ref of="Grp Tab"() -> (w300:refnum<vi>)
      n201 = control-ref of="Sub Graph"() -> (w299:refnum<vi>)
      n202 = control-ref of="Speed Tab"() -> (w285:refnum<vi>)
      n203 = control-ref of="FF Tab"() -> (w254:refnum<vi>)
      n204 = control-ref of="Heater"() -> (w332:refnum<vi>)
      n205 = control-ref of="TK4 status"() -> (w331:refnum<vi>)
      n206 = control-ref of="Controller  Status"() -> (w328:refnum<vi>)
      n207 = control-ref of="Cooling"() -> (w325:refnum<vi>)
      n208 = control-ref of="Load Communication"() -> (w324:refnum<vi>)
      n209 = control-ref of="HumCOMStatus"() -> (w322:refnum<vi>)
      n210 = control-ref of="Load En"() -> (w319:refnum<vi>)
      n211 = control-ref of="NLt"() -> (w318:refnum<vi>)
      n212 = control-ref of="zNL 2"() -> (w317:refnum<vi>)
      n213 = control-ref of="Humidity On"() -> (w316:refnum<vi>)
      n214 = control-ref of="AppLoadSeq scratch"() -> (w312:refnum<vi>)
      n215 = control-ref of="Stop Scratch"() -> (w311:refnum<vi>)
      n216 = control-ref of="ClrLog"() -> (w310:refnum<vi>)
      n217 = control-ref of="STOP"() -> (w308:refnum<vi>)
      n218 = control-ref of="Start Test"() -> (w307:refnum<vi>)
      n219 = control-ref of="Test status"() -> (w306:refnum<vi>)
      n220 = control-ref of="AR Led"() -> (w305:refnum<vi>)
      n221 = control-ref of="Data"() -> (w304:refnum<vi>)
      n222 = control-ref of="Health"() -> (w303:refnum<vi>)
      n223 = control-ref of="Sway COM Status"() -> (w302:refnum<vi>)
      n224 = control-ref of="Heave COM Status"() -> (w301:refnum<vi>)
      n225 = control-ref of="Siliding distance Reset Graph"() -> (w297:refnum<vi>)
      n226 = control-ref of="Humidity Reset Graph"() -> (w295:refnum<vi>)
      n227 = control-ref of="Aqucostic Reset Graph"() -> (w292:refnum<vi>)
      n228 = control-ref of="ECR RESET"() -> (w290:refnum<vi>)
      n229 = control-ref of="Temperature Reset"() -> (w288:refnum<vi>)
      n230 = control-ref of="Speed Reset Graph"() -> (w286:refnum<vi>)
      n231 = control-ref of="Hymidity"() -> (w281:refnum<vi>)
      n232 = control-ref of="Humidity Disable trip"() -> (w280:refnum<vi>)
      n233 = control-ref of="Weart Deapth"() -> (w277:refnum<vi>)
      n234 = control-ref of="Depth Reset Graph"() -> (w276:refnum<vi>)
      n235 = control-ref of="Weart"() -> (w275:refnum<vi>)
      n236 = control-ref of="Depthz"() -> (w274:refnum<vi>)
      n237 = control-ref of="Load pid"() -> (w270:refnum<vi>)
      n238 = control-ref of="Load Disable Trip"() -> (w269:refnum<vi>)
      n239 = control-ref of="Load Reset Graph"() -> (w268:refnum<vi>)
      n240 = control-ref of="BACK"() -> (w265:refnum<vi>)
      n241 = control-ref of="FF Reset Graph"() -> (w261:refnum<vi>)
      n242 = control-ref of="FF Disable Trip"() -> (w260:refnum<vi>)
      n243 = control-ref of="COF Disable Trip"() -> (w257:refnum<vi>)
      n244 = control-ref of="COF Reset Graph"() -> (w256:refnum<vi>)
      n245 = control-ref of="Start Test Temp"() -> (w253:refnum<vi>)
      n246 = control-ref of="Depth Trip"() -> (w264:refnum<vi>)
      n247 = control-ref of="Stroke (mm)"() -> (w353:refnum<vi>)
      n248 = control-ref of="Angle (Deg)"() -> (w352:refnum<vi>)
      n249 = control-ref of="Disc Speed (m/sec)"() -> (w349:refnum<vi>)
      n250 = control-ref of="Ball Speed (m/sec)"() -> (w348:refnum<vi>)
      n251 = control-ref of="Disc Speed (RPM)"() -> (w347:refnum<vi>)
      n252 = control-ref of="Ball Speed (RPM)"() -> (w346:refnum<vi>)
      n253 = control-ref of="Speed (m/sec)"() -> (w344:refnum<vi>)
      n254 = control-ref of="Set Speed (m/sec)"() -> (w343:refnum<vi>)
      n255 = control-ref of="Speed (RPM)"() -> (w342:refnum<vi>)
      n256 = control-ref of="Set Speed"() -> (w341:refnum<vi>)
      n257 = control-ref of="Time ( HH:MM:SS ) 2"() -> (w339:refnum<vi>)
      n258 = control-ref of="Test Duration"() -> (w338:refnum<vi>)
      n259 = control-ref of="Test Duration 4"() -> (w337:refnum<vi>)
      n260 = control-ref of="TEST CYCLE"() -> (w336:refnum<vi>)
      n261 = control-ref of="TOTAL CYCLES"() -> (w335:refnum<vi>)
      n262 = control-ref of="Set Load (N)"() -> (w334:refnum<vi>)
      n263 = control-ref of="ChamberTemp"() -> (w330:refnum<vi>)
      n264 = control-ref of="SetTmp"() -> (w329:refnum<vi>)
      n265 = control-ref of="ChamberTemp"() -> (w327:refnum<vi>)
      n266 = control-ref of="SetTmp"() -> (w326:refnum<vi>)
      n267 = control-ref of="Ambient \nTemperature"() -> (w323:refnum<vi>)
      n268 = control-ref of="Ambient\n Humidity"() -> (w321:refnum<vi>)
      n269 = control-ref of="Freq (Hz)"() -> (w320:refnum<vi>)
      n270 = control-ref of="humidity disp"() -> (w315:refnum<vi>)
      n271 = control-ref of="Set Humidity"() -> (w314:refnum<vi>)
      n272 = control-ref of="NL disp 2"() -> (w313:refnum<vi>)
      n273 = control-ref of="SD (mm)"() -> (w298:refnum<vi>)
      n274 = control-ref of="Acoustic Emission (mV)"() -> (w293:refnum<vi>)
      n275 = control-ref of="CoF Trip  2"() -> (w279:refnum<vi>)
      n276 = control-ref of="Depth Trip"() -> (w278:refnum<vi>)
      n277 = control-ref of="Depth (µm)"() -> (w273:refnum<vi>)
      n278 = control-ref of="NL Trip 2"() -> (w271:refnum<vi>)
      n279 = control-ref of="NL Display 4"() -> (w267:refnum<vi>)
      n280 = control-ref of="COF TRIP"() -> (w263:refnum<vi>)
      n281 = control-ref of="Friction Force (N)"() -> (w262:refnum<vi>)
      n282 = control-ref of="FF TRIP"() -> (w259:refnum<vi>)
      n283 = control-ref of="Trip Log"() -> (w309:refnum<vi>)
      n284 = Bundle By Name(cluster=w357, "Main Screen.Main Screen Tab"=w355, "Main Screen.Angle and Frequency"=w354, "Main Screen.Stroke (mm)"=w353, "Main Screen.Angle (Deg)"=w352, "Main Screen.Main Speed Tab"=w351, "Main Screen.MTM MOTOR DISPLAY"=w350, "Main Screen.Disc Speed (m/sec)"=w349, "Main Screen.Ball Speed (m/sec)"=w348, "Main Screen.Disc Speed (RPM)"=w347, "Main Screen.Ball Speed (RPM)"=w346, "Main Screen.SPEED TAB"=w345, "Main Screen.Speed (m/sec)"=w344, "Main Screen.Set Speed (m/sec)"=w343, "Main Screen.Speed (RPM)"=w342, "Main Screen.Set Speed"=w341, "Main Screen.Time Tab"=w340, "Main Screen.Time ( HH:MM:SS ) 2"=w339, "Main Screen.Test Duration"=w338, "Main Screen.Test Duration 4"=w337, "Main Screen.TEST CYCLE"=w336, "Main Screen.TOTAL CYCLES"=w335, "Main Screen.Set Load (N)"=w334, "Main Screen.Temp Tabs"=w333, "Main Screen.Heater"=w332, "Main Screen.TK4 status"=w331, "Main Screen.ChamberTemp"=w330, "Main Screen.SetTmp"=w329, "Main Screen.Controller  Status"=w328, "Main Screen.ChamberTemp 2"=w327, "Main Screen.SetTmp 2"=w326, "Main Screen.Cooling"=w325, "Main Screen.Load Communication"=w324, "Main Screen.Ambient \nTemperature"=w323, "Main Screen.HumCOMStatus"=w322, "Main Screen.Ambient\n Humidity"=w321, "Main Screen.Freq (Hz)"=w320, "Main Screen.Load En"=w319, "Main Screen.NLt"=w318, "Main Screen.zNL 2"=w317, "Main Screen.Humidity On"=w316, "Main Screen.humidity disp"=w315, "Main Screen.Set Humidity"=w314, "Main Screen.NL disp 2"=w313, "Main Screen.AppLoadSeq scratch"=w312, "Main Screen.Stop Scratch"=w311, "Main Screen.ClrLog"=w310, "Main Screen.Trip Log"=w309, "Main Screen.STOP"=w308, "Main Screen.Start Test"=w307, "Main Screen.Test status"=w306, "Main Screen.AR Led"=w305, "Main Screen.Data"=w304, "Main Screen.Health"=w303, "Main Screen.Sway COM Status"=w302, "Main Screen.Heave COM Status"=w301, "Main Screen.Grp Tab"=w300, "Main Screen.Sub Graph"=w299, "Main Screen.SD (mm)"=w298, "Main Screen.Siliding distance Reset Graph"=w297, "Main Screen.SDGp"=w296, "Main Screen.Humidity Reset Graph"=w295, "Main Screen.HumrGp"=w294, "Main Screen.Acoustic Emission (mV)"=w293, "Main Screen.Aqucostic Reset Graph"=w292, "Main Screen.gACQUOS"=w291, "Main Screen.ECR RESET"=w290, "Main Screen.ECR"=w289, "Main Screen.Temperature Reset"=w288, "Main Screen.Temperature (deg c)"=w287, "Main Screen.Speed Reset Graph"=w286, "Main Screen.Speed Tab"=w285, "Main Screen.MTM DISC  SPEED"=w284, "Main Screen.MTM BALL SPEED"=w283, "Main Screen.speed mm/sec"=w282, "Main Screen.Hymidity"=w281, "Main Screen.Humidity Disable trip"=w280, "Main Screen.CoF Trip  2"=w279, "Main Screen.Depth Trip"=w278, "Main Screen.Weart Deapth"=w277, "Main Screen.Depth Reset Graph"=w276, "Main Screen.Weart"=w275, "Main Screen.Depthz"=w274, "Main Screen.Depth (µm)"=w273, "Main Screen.WearGp"=w272, "Main Screen.NL Trip 2"=w271, "Main Screen.Load pid"=w270, "Main Screen.Load Disable Trip"=w269, "Main Screen.Load Reset Graph"=w268, "Main Screen.NL Display 4"=w267, "Main Screen.Main Chart 3"=w266, "Main Screen.BACK"=w265, "Main Screen.Depth Trip 2"=w264, "Main Screen.COF TRIP"=w263, "Main Screen.Friction Force (N)"=w262, "Main Screen.FF Reset Graph"=w261, "Main Screen.FF Disable Trip"=w260, "Main Screen.FF TRIP"=w259, "Main Screen.FF MAIN CHART"=w258, "Main Screen.COF Disable Trip"=w257, "Main Screen.COF Reset Graph"=w256, "Main Screen.COF MAIN CHART"=w255, "Main Screen.FF Tab"=w254, "Main Screen.Start Test Temp"=w253) -> (w356:T12)
    }
    frame #9 {
      n285 = control-ref of="gFF Rot 7"() -> (w361:refnum<vi>)
      n286 = control-ref of="Ramp"() -> (w380:refnum<vi>)
      n287 = control-ref of="Dummy Run"() -> (w374:refnum<vi>)
      n288 = control-ref of="AutoTune"() -> (w372:refnum<vi>)
      n289 = control-ref of="apply load"() -> (w370:refnum<vi>)
      n290 = control-ref of="reinit 3"() -> (w368:refnum<vi>)
      n291 = control-ref of="Bypass Load"() -> (w365:refnum<vi>)
      n292 = control-ref of="PID gains out delay (microForce)"() -> (w381:refnum<vi>)
      n293 = control-ref of="output range delay"() -> (w367:refnum<vi>)
      n294 = control-ref of="PID gains out delay"() -> (w366:refnum<vi>)
      n295 = control-ref of="Ramp MulFac"() -> (w385:refnum<vi>)
      n296 = control-ref of="pulses LoadDiffRamp(2..10)"() -> (w384:refnum<vi>)
      n297 = control-ref of="PulseControlRamp(diff<=3N)"() -> (w383:refnum<vi>)
      n298 = control-ref of="SetLoadDeadband(%) Load(0-10N)"() -> (w382:refnum<vi>)
      n299 = control-ref of="Gain 2"() -> (w379:refnum<vi>)
      n300 = control-ref of="pulses LoadDiff(2..10)"() -> (w378:refnum<vi>)
      n301 = control-ref of="pulses LoadDiff(11..50)"() -> (w377:refnum<vi>)
      n302 = control-ref of="PulseControl(diff<=3N)"() -> (w376:refnum<vi>)
      n303 = control-ref of="SetLoadDeadband(%)  2"() -> (w375:refnum<vi>)
      n304 = control-ref of="Vertical load (N)"() -> (w373:refnum<vi>)
      n305 = control-ref of="Offset  3"() -> (w371:refnum<vi>)
      n306 = control-ref of="Enter ByPass Load"() -> (w369:refnum<vi>)
      n307 = control-ref of="pulsesSent"() -> (w364:refnum<vi>)
      n308 = control-ref of="pulses"() -> (w363:refnum<vi>)
      n309 = control-ref of="actpid"() -> (w362:refnum<vi>)
      n310 = control-ref of="pulses LoadDiff(21..1000)"() -> (w360:refnum<vi>)
      n311 = control-ref of="Delay"() -> (w359:refnum<vi>)
      n312 = control-ref of="deadband"() -> (w358:refnum<vi>)
      n313 = Bundle By Name(cluster=w387, "PID.Ramp MulFac"=w385, "PID.pulses LoadDiffRamp(2..10)"=w384, "PID.PulseControlRamp(diff<=3N)"=w383, "PID.SetLoadDeadband(%) Load(0-10N)"=w382, "PID.PID gains out delay (microForce)"=w381, "PID.Ramp"=w380, "PID.Gain 2"=w379, "PID.pulses LoadDiff(2..10)"=w378, "PID.pulses LoadDiff(11..50)"=w377, "PID.PulseControl(diff<=3N)"=w376, "PID.SetLoadDeadband(%)  2"=w375, "PID.Dummy Run"=w374, "PID.Vertical load (N)"=w373, "PID.AutoTune"=w372, "PID.Offset 3"=w371, "PID.apply load"=w370, "PID.Enter ByPass Load"=w369, "PID.reinit 3"=w368, "PID.output range delay"=w367, "PID.PID gains out delay"=w366, "PID.Bypass Load"=w365, "PID.pulsesSent"=w364, "PID.pulses"=w363, "PID.actpid"=w362, "PID.gFF Rot"=w361, "PID.pulses LoadDiff(21..1000)"=w360, "PID.Delay"=w359, "PID.deadband"=w358) -> (w386:T12)
    }
    frame #10 {
      n314 = control-ref of="Tab Control 3"() -> (w435:refnum<vi>)
      n315 = control-ref of="Tab Control 19"() -> (w434:refnum<vi>)
      n316 = control-ref of="Tab Control 5"() -> (w395:refnum<vi>)
      n317 = control-ref of="Tab Control 14"() -> (w394:refnum<vi>)
      n318 = control-ref of="Tab Control 26"() -> (w393:refnum<vi>)
      n319 = control-ref of="Re-initilaize"() -> (w432:refnum<vi>)
      n320 = control-ref of="Filter ON/OFF"() -> (w431:refnum<vi>)
      n321 = control-ref of="Apply Filter (FF)"() -> (w427:refnum<vi>)
      n322 = control-ref of="Apply Filter (Load)"() -> (w425:refnum<vi>)
      n323 = control-ref of="SAVE  2"() -> (w420:refnum<vi>)
      n324 = control-ref of="Enter Distance"() -> (w419:refnum<vi>)
      n325 = control-ref of="AE"() -> (w392:refnum<vi>)
      n326 = control-ref of="Heave Loop Delay"() -> (w391:refnum<vi>)
      n327 = control-ref of="Heave PID Speed"() -> (w390:refnum<vi>)
      n328 = control-ref of="Surge Jog Speed"() -> (w389:refnum<vi>)
      n329 = control-ref of="Heave Jog Speed"() -> (w388:refnum<vi>)
      n330 = control-ref of="SAMPLES"() -> (w433:refnum<vi>)
      n331 = control-ref of="TracHomeSurgeOffsetCounts 10MM"() -> (w430:refnum<vi>)
      n332 = control-ref of="TracHomeSwayOffsetCounts 10MM"() -> (w429:refnum<vi>)
      n333 = control-ref of="Acoustic Emission:"() -> (w428:refnum<vi>)
      n334 = control-ref of="Filter% 2"() -> (w426:refnum<vi>)
      n335 = control-ref of="Filter%"() -> (w424:refnum<vi>)
      n336 = control-ref of="Sway distance (mm)"() -> (w423:refnum<vi>)
      n337 = control-ref of="Surge distance (mm)"() -> (w422:refnum<vi>)
      n338 = control-ref of="DataSavingLoopDelay(ms)"() -> (w421:refnum<vi>)
      n339 = control-ref of="Sway Counts:"() -> (w418:refnum<vi>)
      n340 = control-ref of="Distance (mm): 3"() -> (w417:refnum<vi>)
      n341 = control-ref of="Surge Counts:"() -> (w416:refnum<vi>)
      n342 = control-ref of="Distance (mm): 2"() -> (w415:refnum<vi>)
      n343 = control-ref of="Distance (mm):"() -> (w414:refnum<vi>)
      n344 = control-ref of="Heave Counts:"() -> (w413:refnum<vi>)
      n345 = control-ref of="LRMHomeSurgeOffsetCounts"() -> (w412:refnum<vi>)
      n346 = control-ref of="LRMHomeSwayOffsetCounts"() -> (w411:refnum<vi>)
      n347 = control-ref of="TracHomeSurgeOffsetCounts 20MM"() -> (w410:refnum<vi>)
      n348 = control-ref of="TracHomeSwayOffsetCounts 20MM"() -> (w409:refnum<vi>)
      n349 = control-ref of="RotHomeSwayOffsetCounts"() -> (w408:refnum<vi>)
      n350 = control-ref of="RotHomeSurgeOffsetCounts"() -> (w407:refnum<vi>)
      n351 = control-ref of="Heave distance"() -> (w406:refnum<vi>)
      n352 = control-ref of="Zmm"() -> (w405:refnum<vi>)
      n353 = control-ref of="Heave Pulses/mm"() -> (w404:refnum<vi>)
      n354 = control-ref of="Surge Pulses/mm"() -> (w403:refnum<vi>)
      n355 = control-ref of="Sway Pulses/mm"() -> (w402:refnum<vi>)
      n356 = control-ref of="Heave Pitch"() -> (w401:refnum<vi>)
      n357 = control-ref of="Surge Pitch"() -> (w400:refnum<vi>)
      n358 = control-ref of="Sway Pitch"() -> (w399:refnum<vi>)
      n359 = control-ref of="Heave PPR"() -> (w398:refnum<vi>)
      n360 = control-ref of="Surge PPR"() -> (w397:refnum<vi>)
      n361 = control-ref of="Sway PPR"() -> (w396:refnum<vi>)
      n362 = Bundle By Name(cluster=w437, "Config Parameters.Tab Control 3"=w435, "Config Parameters.Tab Control 19"=w434, "Config Parameters.SAMPLES"=w433, "Config Parameters.Re-initilaize"=w432, "Config Parameters.Filter ON/OFF"=w431, "Config Parameters.TracHomeSurgeOffsetCounts 10MM"=w430, "Config Parameters.TracHomeSwayOffsetCounts 10MM"=w429, "Config Parameters.Acoustic Emission:"=w428, "Config Parameters.Apply Filter (FF)"=w427, "Config Parameters.Filter% 2"=w426, "Config Parameters.Apply Filter (Load)"=w425, "Config Parameters.Filter%"=w424, "Config Parameters.Sway distance (mm)"=w423, "Config Parameters.Surge distance (mm)"=w422, "Config Parameters.DataSavingLoopDelay(ms)"=w421, "Config Parameters.SAVE 2"=w420, "Config Parameters.Enter Distance"=w419, "Config Parameters.Sway Counts:"=w418, "Config Parameters.Distance (mm): 3"=w417, "Config Parameters.Surge Counts:"=w416, "Config Parameters.Distance (mm): 2"=w415, "Config Parameters.Distance (mm):"=w414, "Config Parameters.Heave Counts:"=w413, "Config Parameters.LRMHomeSurgeOffsetCounts"=w412, "Config Parameters.LRMHomeSwayOffsetCounts"=w411, "Config Parameters.TracHomeSurgeOffsetCounts 20MM"=w410, "Config Parameters.TracHomeSwayOffsetCounts 20MM"=w409, "Config Parameters.RotHomeSwayOffsetCounts"=w408, "Config Parameters.RotHomeSurgeOffsetCounts"=w407, "Config Parameters.Heave distance"=w406, "Config Parameters.Zmm"=w405, "Config Parameters.Heave Pulses/mm"=w404, "Config Parameters.Surge Pulses/mm"=w403, "Config Parameters.Sway Pulses/mm"=w402, "Config Parameters.Heave Pitch"=w401, "Config Parameters.Surge Pitch"=w400, "Config Parameters.Sway Pitch"=w399, "Config Parameters.Heave PPR"=w398, "Config Parameters.Surge PPR"=w397, "Config Parameters.Sway PPR"=w396, "Config Parameters.Tab Control 5"=w395, "Config Parameters.Tab Control 14"=w394, "Config Parameters.Tab Control 26"=w393, "Config Parameters.AE"=w392, "Config Parameters.Heave Loop Delay"=w391, "Config Parameters.Heave PID Speed"=w390, "Config Parameters.Surge Jog Speed"=w389, "Config Parameters.Heave Jog Speed"=w388) -> (w436:T12)
    }
    frame #11 {
      n363 = control-ref of="Mx"() -> (w467:refnum<vi>)
      n364 = control-ref of="My"() -> (w466:refnum<vi>)
      n365 = control-ref of="Mz"() -> (w465:refnum<vi>)
      n366 = control-ref of="Fx(N)"() -> (w464:refnum<vi>)
      n367 = control-ref of="Fy(N)"() -> (w463:refnum<vi>)
      n368 = control-ref of="Fz(N)"() -> (w462:refnum<vi>)
      n369 = control-ref of="Load Cell Temp"() -> (w438:refnum<vi>)
      n370 = control-ref of="ClearAll"() -> (w472:refnum<vi>)
      n371 = control-ref of="ZeroAll"() -> (w461:refnum<vi>)
      n372 = control-ref of="delete Handle"() -> (w451:refnum<vi>)
      n373 = control-ref of="Create Handle"() -> (w450:refnum<vi>)
      n374 = control-ref of="stop 6"() -> (w447:refnum<vi>)
      n375 = control-ref of="running_flag"() -> (w446:refnum<vi>)
      n376 = control-ref of="Save Dwell"() -> (w468:refnum<vi>)
      n377 = control-ref of="Acq Delay (ms)"() -> (w460:refnum<vi>)
      n378 = control-ref of="Burst Delay (ms)"() -> (w459:refnum<vi>)
      n379 = control-ref of="SN"() -> (w457:refnum<vi>)
      n380 = control-ref of="Port"() -> (w454:refnum<vi>)
      n381 = control-ref of="ft_udp_handle"() -> (w445:refnum<vi>)
      n382 = control-ref of="get-data-return"() -> (w444:refnum<vi>)
      n383 = control-ref of="get-range-return"() -> (w443:refnum<vi>)
      n384 = control-ref of="zero-return"() -> (w442:refnum<vi>)
      n385 = control-ref of="filter-return"() -> (w441:refnum<vi>)
      n386 = control-ref of="initial-return"() -> (w440:refnum<vi>)
      n387 = control-ref of="deleteHandle-result"() -> (w439:refnum<vi>)
      n388 = control-ref of="model"() -> (w458:refnum<vi>)
      n389 = control-ref of="Sensor IP"() -> (w455:refnum<vi>)
      n390 = control-ref of="Mz(Nm)"() -> (w471:refnum<vi>)
      n391 = control-ref of="My(Nm)"() -> (w470:refnum<vi>)
      n392 = control-ref of="Mx(Nm)"() -> (w469:refnum<vi>)
      n393 = control-ref of="FFx(N)"() -> (w456:refnum<vi>)
      n394 = control-ref of="FFy(N)"() -> (w453:refnum<vi>)
      n395 = control-ref of="Load(N)"() -> (w452:refnum<vi>)
      n396 = control-ref of="ft_data"() -> (w449:refnum<vi>)
      n397 = control-ref of="ft_range"() -> (w448:refnum<vi>)
      n398 = Bundle By Name(cluster=w474, "Loading Com Port.ClearAll"=w472, "Loading Com Port.Mz(Nm)"=w471, "Loading Com Port.My(Nm)"=w470, "Loading Com Port.Mx(Nm)"=w469, "Loading Com Port.Save Dwell"=w468, "Loading Com Port.Mx"=w467, "Loading Com Port.My"=w466, "Loading Com Port.Mz"=w465, "Loading Com Port.Fx(N)"=w464, "Loading Com Port.Fy(N)"=w463, "Loading Com Port.Fz(N)"=w462, "Loading Com Port.ZeroAll"=w461, "Loading Com Port.Acq Delay (ms)"=w460, "Loading Com Port.Burst Delay (ms)"=w459, "Loading Com Port.model"=w458, "Loading Com Port.SN"=w457, "Loading Com Port.FFx(N)"=w456, "Loading Com Port.Sensor IP"=w455, "Loading Com Port.Port"=w454, "Loading Com Port.FFy(N)"=w453, "Loading Com Port.Load(N)"=w452, "Loading Com Port.delete Handle"=w451, "Loading Com Port.Create Handle"=w450, "Loading Com Port.ft_data"=w449, "Loading Com Port.ft_range"=w448, "Loading Com Port.stop 6"=w447, "Loading Com Port.running_flag"=w446, "Loading Com Port.ft_udp_handle"=w445, "Loading Com Port.get-data-return"=w444, "Loading Com Port.get-range-return"=w443, "Loading Com Port.zero-return"=w442, "Loading Com Port.filter-return"=w441, "Loading Com Port.initial-return"=w440, "Loading Com Port.deleteHandle-result"=w439, "Loading Com Port.Load Cell Temp"=w438) -> (w473:T12)
    }
    frame #12 {
      n399 = control-ref of="Manual Write Heave & Surge"() -> (w476:refnum<vi>)
      n400 = control-ref of="Read Heave Temp"() -> (w499:refnum<vi>)
      n401 = control-ref of="error out Read"() -> (w511:refnum<vi>)
      n402 = control-ref of="error out Write"() -> (w506:refnum<vi>)
      n403 = control-ref of="SURGE POSE"() -> (w512:refnum<vi>)
      n404 = control-ref of="HEAVE POSE"() -> (w510:refnum<vi>)
      n405 = control-ref of="State"() -> (w509:refnum<vi>)
      n406 = control-ref of="Homed"() -> (w508:refnum<vi>)
      n407 = control-ref of="Sequence ID"() -> (w507:refnum<vi>)
      n408 = control-ref of="faultCode"() -> (w505:refnum<vi>)
      n409 = control-ref of="Ack ID"() -> (w504:refnum<vi>)
      n410 = control-ref of="SPEED"() -> (w503:refnum<vi>)
      n411 = control-ref of="Distance"() -> (w502:refnum<vi>)
      n412 = control-ref of="Mode Command"() -> (w501:refnum<vi>)
      n413 = control-ref of="SPARE 2"() -> (w498:refnum<vi>)
      n414 = control-ref of="SPARE 1"() -> (w497:refnum<vi>)
      n415 = control-ref of="Spare 15"() -> (w496:refnum<vi>)
      n416 = control-ref of="Spare 14"() -> (w495:refnum<vi>)
      n417 = control-ref of="Spare 13"() -> (w494:refnum<vi>)
      n418 = control-ref of="Spare 12"() -> (w493:refnum<vi>)
      n419 = control-ref of="Spare 11"() -> (w492:refnum<vi>)
      n420 = control-ref of="Spare 10"() -> (w491:refnum<vi>)
      n421 = control-ref of="Spare 9"() -> (w490:refnum<vi>)
      n422 = control-ref of="Spare 8"() -> (w489:refnum<vi>)
      n423 = control-ref of="Spare 7"() -> (w488:refnum<vi>)
      n424 = control-ref of="Spare 6"() -> (w487:refnum<vi>)
      n425 = control-ref of="Spare 5"() -> (w486:refnum<vi>)
      n426 = control-ref of="Spare 4"() -> (w485:refnum<vi>)
      n427 = control-ref of="Spare 3"() -> (w484:refnum<vi>)
      n428 = control-ref of="Spare 2"() -> (w483:refnum<vi>)
      n429 = control-ref of="Spare 1"() -> (w482:refnum<vi>)
      n430 = control-ref of="Node Id"() -> (w481:refnum<vi>)
      n431 = control-ref of="SPARE 3"() -> (w480:refnum<vi>)
      n432 = control-ref of="SPARE 4"() -> (w479:refnum<vi>)
      n433 = control-ref of="fwMajor"() -> (w478:refnum<vi>)
      n434 = control-ref of="fwMinor"() -> (w477:refnum<vi>)
      n435 = control-ref of="Heave and Surge Write"() -> (w475:refnum<vi>)
      n436 = control-ref of="Heave and Surge Read"() -> (w500:refnum<vi>)
      n437 = Bundle By Name(cluster=w514, "Heave AND Surge.SURGE POSE"=w512, "Heave AND Surge.error out Read"=w511, "Heave AND Surge.HEAVE POSE"=w510, "Heave AND Surge.State"=w509, "Heave AND Surge.Homed"=w508, "Heave AND Surge.Sequence ID"=w507, "Heave AND Surge.error out Write"=w506, "Heave AND Surge.faultCode"=w505, "Heave AND Surge.Ack ID"=w504, "Heave AND Surge.SPEED"=w503, "Heave AND Surge.Distance"=w502, "Heave AND Surge.Mode Command"=w501, "Heave AND Surge.Heave and Surge Read"=w500, "Heave AND Surge.Read Heave Temp"=w499, "Heave AND Surge.SPARE 2"=w498, "Heave AND Surge.SPARE 1"=w497, "Heave AND Surge.Spare 15"=w496, "Heave AND Surge.Spare 14"=w495, "Heave AND Surge.Spare 13"=w494, "Heave AND Surge.Spare 12"=w493, "Heave AND Surge.Spare 11"=w492, "Heave AND Surge.Spare 10"=w491, "Heave AND Surge.Spare 9"=w490, "Heave AND Surge.Spare 8"=w489, "Heave AND Surge.Spare 7"=w488, "Heave AND Surge.Spare 6"=w487, "Heave AND Surge.Spare 5"=w486, "Heave AND Surge.Spare 4"=w485, "Heave AND Surge.Spare 3"=w484, "Heave AND Surge.Spare 2"=w483, "Heave AND Surge.Spare 1"=w482, "Heave AND Surge.Node Id"=w481, "Heave AND Surge.SPARE 3"=w480, "Heave AND Surge.SPARE 4"=w479, "Heave AND Surge.fwMajor"=w478, "Heave AND Surge.fwMinor"=w477, "Heave AND Surge.Manual Write"=w476, "Heave AND Surge.Heave and Surge Write"=w475) -> (w513:T12)
    }
    frame #13 {
      n438 = control-ref of="Fine Tune Zone"() -> (w530:refnum<vi>)
      n439 = control-ref of="PID Delay (sec)"() -> (w529:refnum<vi>)
      n440 = control-ref of="Max_pos_limit"() -> (w528:refnum<vi>)
      n441 = control-ref of="Min_pos_limit"() -> (w527:refnum<vi>)
      n442 = control-ref of="i_limit"() -> (w526:refnum<vi>)
      n443 = control-ref of="pct_scale"() -> (w517:refnum<vi>)
      n444 = control-ref of="Deadband"() -> (w525:refnum<vi>)
      n445 = control-ref of="Kd"() -> (w524:refnum<vi>)
      n446 = control-ref of="Ki"() -> (w523:refnum<vi>)
      n447 = control-ref of="Kp"() -> (w522:refnum<vi>)
      n448 = control-ref of="Current Position"() -> (w521:refnum<vi>)
      n449 = control-ref of="Set Load"() -> (w520:refnum<vi>)
      n450 = control-ref of="Current Load"() -> (w519:refnum<vi>)
      n451 = control-ref of="Pulse delta"() -> (w518:refnum<vi>)
      n452 = control-ref of="Init Step"() -> (w516:refnum<vi>)
      n453 = control-ref of="Max Step Linit"() -> (w515:refnum<vi>)
      n454 = Bundle By Name(cluster=w532, "New PID LOGIC.Fine Tune Zone"=w530, "New PID LOGIC.PID SDelay"=w529, "New PID LOGIC.Max_pos_limit"=w528, "New PID LOGIC.Min_pos_limit"=w527, "New PID LOGIC.i_limit"=w526, "New PID LOGIC.pct_scale"=w517, "New PID LOGIC.Deadband"=w525, "New PID LOGIC.Kd"=w524, "New PID LOGIC.Ki"=w523, "New PID LOGIC.Kp"=w522, "New PID LOGIC.Current Position"=w521, "New PID LOGIC.Set Load"=w520, "New PID LOGIC.Current Load"=w519, "New PID LOGIC.Pulse delta"=w518, "New PID LOGIC.Init Step"=w516, "New PID LOGIC.Max Step Linit"=w515) -> (w531:T12)
    }
  }
  n455 = call <userlib>:"Fit VI window to Largest Dec.vi"() -> ("error out"=w42:errorcluster, "dup VI Ref"=w39:refnum<vi>)  [unwired: 6 in]
  n456 = invoke on="Invoke Node" class="VI" method="FP.Run-Time Position.Maximized"(reference=w39, error in=w42) -> (error out=w41:errorcluster)  [unwired: 2 in, 3 out]
  n457 = call <vilib>:"Clear Errors.vi"("error in (no error)"=w41) -> ("error out"=w40:errorcluster)  [unwired: 5 in, 1 out]
  n458 = control-ref of="This VI"() -> (w45:refnum<vi>)
  n459 = invoke on="Invoke Node" class="VI" method="Default Vals.Reinit All"(reference=w45, error in=w40) -> (reference out=w43:refnum<vi>, error out=w44:errorcluster)  [unwired: 1 in, 1 out]
  n460 = Close Reference(reference=w43, error in (no error)=w44) -> (error out=w38:errorcluster)
  n461 = call "Create User Event - Stop.vi"("error in (no error)"=w38) -> ("error out"=w13:errorcluster, "User Event - Stop"=w25:refnum<user-event>)  [unwired: 9 in]
  n462 = call "main screen queue out Unitest.vi"("error in (no error)"=w13) -> ("error out"=w65:errorcluster, "output Queue"=w37:T13)  [unwired: 9 in]
  n463 = Unbundle By Name(w37) -> ("UI Loop"=w63:refnum<queue>)
  n464 = Unbundle By Name(w37) -> ("LOAD COM LOOP"=w35:refnum<queue>)
  n465 = Unbundle By Name(w37) -> ("SWAY MOTOR COM LOOP"=w34:refnum<queue>)
  n466 = Unbundle By Name(w37) -> ("HEAVE MOTOR COM LOOP"=w17:refnum<queue>)
  n467 = Unbundle By Name(w37) -> ("TEMPERATURE COM LOOP"=w32:refnum<queue>)
  n468 = Unbundle By Name(w37) -> ("RAMP MOTOR COM LOOP"=w29:refnum<queue>)
  n469 = Unbundle By Name(w37) -> ("ECR PORT"=w28:refnum<queue>)
  n470 = Unbundle By Name(w37) -> ("HUMIDITY COM PORT"=w27:refnum<queue>)
  n471 = Unbundle By Name(w37) -> ("PROGRAM LOOP"=w26:refnum<queue>)
  n472 = Unbundle By Name(w37) -> ("MONITOR LOOP"=w24:refnum<queue>)
  n473 = Unbundle By Name(w37) -> ("LOAD PID"=w23:refnum<queue>)
  n474 = Unbundle By Name(w37) -> ("REPORT"=w22:refnum<queue>)
  n475 = register-events(w25) -> (reference out=w57:refnum<event-registration>, error out=w55:errorcluster)  [unwired: 2 in]
  n476 = Merge Errors(w55, w65) -> (w56:errorcluster)
  n477 = while {
    tunnel: w63 -> [w540]
    shift-right: [w538] -> w60
    shift-left: w57 -> [w539]
    tunnel: [w534] -> w58
    stop <- w536 stop-if-true
    # "Event Handling Loop"
    n478 = event shown="[35] \"STOP\": Value Change" {
      selector: w539 -> [_ _ _ _ _ _ _ _ _ _ _ _ _ _ _ _ _ _ _ _ _ _ _ _ _ _ _ _ _ _ _ _ _ _ _ _ _ _ _]
      dyn-events: [_ _ _ _ _ _ _ _ _ _ _ _ _ _ _ _ _ _ _ _ _ _ _ _ _ _ _ _ _ _ _ _ _ _ _ _ _ _ _] -> w538
      timeout: 100 -> [_ _ _ _ _ _ _ _ _ _ _ _ _ _ _ _ _ _ _ _ _ _ _ _ _ _ _ _ _ _ _ _ _ _ _ _ _ _ _]
      tunnel: [_ _ _ _ _ _ _ _ _ _ _ _ _ _ _ _ _ _ _ _ _ _ _ _ _ _ _ _ _ _ _ _ _ _ _ _ _ _ TRUE ("Discard?")] -> w536
      tunnel: w540 -> [w545 w549 w554 w559 w564 w569 w574 w579 w584 w589 w594 w599 w604 w609 w614 w619 w624 w629 w634 w639 w644 w649 w654 w659 w664 w669 w674 w679 w684 w689 w694 w699 w704 w709 w714 w719 w722 w727 w729]
      tunnel: [w544 w547 w552 w557 w562 w567 w572 w577 w582 w587 w592 w597 w602 w607 w612 w617 w622 w627 w632 w637 w642 w647 w652 w657 w662 w667 w672 w677 w682 w687 w692 w697 w702 w707 w712 w717 _ w726 _] -> w537
      tunnel: [w543 w548 w553 w558 w563 w568 w573 w578 w583 w588 w593 w598 w603 w608 w613 w618 w623 w628 w633 w638 w643 w648 w653 w658 w663 w668 w673 w678 w683 w688 w693 w698 w703 w708 w713 w718 w722 w725 w729] -> w535
      event Panel Close? {
        n479 = event-data() -> ()  [unwired: 1 in, 1 out]
        n480 = call-poly "Enqueue Message.vi"("Priority Message? (F)"=TRUE, "Message"="Confirm Quit", "Message Queue"=w545) -> ("error out"=w544:errorcluster, "dup Message Queue"=w543:refnum<queue>)  [unwired: 7 in]
        n481 = event-data("Discard?"=TRUE) -> ()  [unwired: 1 in, 1 out]
      }
      event Timeout {
        n482 = event-data() -> ()  [unwired: 1 in, 1 out]
        n483 = call-poly "Enqueue Message.vi"("Priority Message? (F)"=TRUE, "Message"="Time Out", "Message Queue"=w549) -> ("error out"=w547:errorcluster, "dup Message Queue"=w548:refnum<queue>)  [unwired: 7 in]
      }
      event "SAVE  2": Value Change {
        n484 = event-data() -> ()  [unwired: 1 in, 1 out]
        n485 = call-poly "Enqueue Message.vi"("Priority Message? (F)"=TRUE, "Message"="Service Save", "Message Queue"=w554) -> ("error out"=w552:errorcluster, "dup Message Queue"=w553:refnum<queue>)  [unwired: 7 in]
      }
      event "Home": Value Change {
        n486 = event-data() -> ()  [unwired: 1 in, 1 out]
        n487 = call-poly "Enqueue Message.vi"("Priority Message? (F)"=TRUE, "Message"="HOME", "Message Queue"=w559) -> ("error out"=w557:errorcluster, "dup Message Queue"=w558:refnum<queue>)  [unwired: 7 in]
      }
      event "Platform Settings": Value Change {
        n488 = event-data() -> ()  [unwired: 1 in, 1 out]
        n489 = call-poly "Enqueue Message.vi"("Priority Message? (F)"=TRUE, "Message"="Platform Setting", "Message Queue"=w564) -> ("error out"=w562:errorcluster, "dup Message Queue"=w563:refnum<queue>)  [unwired: 7 in]
      }
      event "Configure": Value Change {
        n490 = event-data() -> ()  [unwired: 1 in, 1 out]
        n491 = call-poly "Enqueue Message.vi"("Priority Message? (F)"=TRUE, "Message"="Configure", "Message Queue"=w569) -> ("error out"=w567:errorcluster, "dup Message Queue"=w568:refnum<queue>)  [unwired: 7 in]
      }
      event "Analysis": Value Change {
        n492 = event-data() -> ()  [unwired: 1 in, 1 out]
        n493 = call-poly "Enqueue Message.vi"("Priority Message? (F)"=TRUE, "Message"="Analysis", "Message Queue"=w574) -> ("error out"=w572:errorcluster, "dup Message Queue"=w573:refnum<queue>)  [unwired: 7 in]
      }
      event "service 2": Value Change {
        n494 = event-data() -> ()  [unwired: 1 in, 1 out]
        n495 = call-poly "Enqueue Message.vi"("Priority Message? (F)"=TRUE, "Message"="service 2", "Message Queue"=w579) -> ("error out"=w577:errorcluster, "dup Message Queue"=w578:refnum<queue>)  [unwired: 7 in]
      }
      event "Auto": Value Change {
        n496 = event-data() -> ()  [unwired: 1 in, 1 out]
        n497 = call-poly "Enqueue Message.vi"("Priority Message? (F)"=TRUE, "Message"="Auto", "Message Queue"=w584) -> ("error out"=w582:errorcluster, "dup Message Queue"=w583:refnum<queue>)  [unwired: 7 in]
      }
      event "Select Load Head": Value Change {
        n498 = event-data() -> ()  [unwired: 1 in, 1 out]
        n499 = call-poly "Enqueue Message.vi"("Priority Message? (F)"=TRUE, "Message"="Select Load Head", "Message Queue"=w589) -> ("error out"=w587:errorcluster, "dup Message Queue"=w588:refnum<queue>)  [unwired: 7 in]
      }
      event "com 3": Value Change {
        n500 = event-data() -> ()  [unwired: 1 in, 1 out]
        n501 = call-poly "Enqueue Message.vi"("Priority Message? (F)"=TRUE, "Message"="com 3", "Message Queue"=w594) -> ("error out"=w592:errorcluster, "dup Message Queue"=w593:refnum<queue>)  [unwired: 7 in]
      }
      event "Loading Mode": Value Change {
        n502 = event-data() -> ()  [unwired: 1 in, 1 out]
        n503 = call-poly "Enqueue Message.vi"("Priority Message? (F)"=TRUE, "Message"="Loading Mode", "Message Queue"=w599) -> ("error out"=w597:errorcluster, "dup Message Queue"=w598:refnum<queue>)  [unwired: 7 in]
      }
      event "SSP 0.3": Value Change {
        n504 = event-data() -> ()  [unwired: 1 in, 1 out]
        n505 = call-poly "Enqueue Message.vi"("Priority Message? (F)"=TRUE, "Message"="SSP 0.3", "Message Queue"=w604) -> ("error out"=w602:errorcluster, "dup Message Queue"=w603:refnum<queue>)  [unwired: 7 in]
      }
      event "SSP 0.5": Value Change {
        n506 = event-data() -> ()  [unwired: 1 in, 1 out]
        n507 = call-poly "Enqueue Message.vi"("Priority Message? (F)"=TRUE, "Message"="SSP 0.5", "Message Queue"=w609) -> ("error out"=w607:errorcluster, "dup Message Queue"=w608:refnum<queue>)  [unwired: 7 in]
      }
      event "SSP 0.75": Value Change {
        n508 = event-data() -> ()  [unwired: 1 in, 1 out]
        n509 = call-poly "Enqueue Message.vi"("Priority Message? (F)"=TRUE, "Message"="SSP 0.75", "Message Queue"=w614) -> ("error out"=w612:errorcluster, "dup Message Queue"=w613:refnum<queue>)  [unwired: 7 in]
      }
      event "LHBack": Value Change {
        n510 = event-data() -> ()  [unwired: 1 in, 1 out]
        n511 = call-poly "Enqueue Message.vi"("Priority Message? (F)"=TRUE, "Message"="LHBack", "Message Queue"=w619) -> ("error out"=w617:errorcluster, "dup Message Queue"=w618:refnum<queue>)  [unwired: 7 in]
      }
      event "LHNext": Value Change {
        n512 = event-data() -> ()  [unwired: 1 in, 1 out]
        n513 = call-poly "Enqueue Message.vi"("Priority Message? (F)"=TRUE, "Message"="LHNext", "Message Queue"=w624) -> ("error out"=w622:errorcluster, "dup Message Queue"=w623:refnum<queue>)  [unwired: 7 in]
      }
      event "Rot Ver": Value Change {
        n514 = event-data() -> ()  [unwired: 1 in, 1 out]
        n515 = call-poly "Enqueue Message.vi"("Priority Message? (F)"=TRUE, "Message"="Rot Ver", "Message Queue"=w629) -> ("error out"=w627:errorcluster, "dup Message Queue"=w628:refnum<queue>)  [unwired: 7 in]
      }
      event "Scratch": Value Change {
        n516 = event-data() -> ()  [unwired: 1 in, 1 out]
        n517 = call-poly "Enqueue Message.vi"("Priority Message? (F)"=TRUE, "Message"="Scratch", "Message Queue"=w634) -> ("error out"=w632:errorcluster, "dup Message Queue"=w633:refnum<queue>)  [unwired: 7 in]
      }
      event "Motion Mode:": Value Change {
        n518 = event-data() -> ()  [unwired: 1 in, 1 out]
        n519 = call-poly "Enqueue Message.vi"("Priority Message? (F)"=TRUE, "Message"="Motion Mode:", "Message Queue"=w639) -> ("error out"=w637:errorcluster, "dup Message Queue"=w638:refnum<queue>)  [unwired: 7 in]
      }
      event "MMBack": Value Change {
        n520 = event-data() -> ()  [unwired: 1 in, 1 out]
        n521 = call-poly "Enqueue Message.vi"("Priority Message? (F)"=TRUE, "Message"="MMBack", "Message Queue"=w644) -> ("error out"=w642:errorcluster, "dup Message Queue"=w643:refnum<queue>)  [unwired: 7 in]
      }
      event "MMNext": Value Change {
        n522 = event-data() -> ()  [unwired: 1 in, 1 out]
        n523 = call-poly "Enqueue Message.vi"("Priority Message? (F)"=TRUE, "Message"="MMNext", "Message Queue"=w649) -> ("error out"=w647:errorcluster, "dup Message Queue"=w648:refnum<queue>)  [unwired: 7 in]
      }
      event "APBack": Value Change {
        n524 = event-data() -> ()  [unwired: 1 in, 1 out]
        n525 = call-poly "Enqueue Message.vi"("Priority Message? (F)"=TRUE, "Message"="APBack", "Message Queue"=w654) -> ("error out"=w652:errorcluster, "dup Message Queue"=w653:refnum<queue>)  [unwired: 7 in]
      }
      event "SNext": Value Change {
        n526 = event-data() -> ()  [unwired: 1 in, 1 out]
        n527 = call-poly "Enqueue Message.vi"("Priority Message? (F)"=TRUE, "Message"="SNext", "Message Queue"=w659) -> ("error out"=w657:errorcluster, "dup Message Queue"=w658:refnum<queue>)  [unwired: 7 in]
      }
      event "ZeroAll": Value Change {
        n528 = event-data() -> ()  [unwired: 1 in, 1 out]
        n529 = call-poly "Enqueue Message.vi"("Priority Message? (F)"=TRUE, "Message"="ZeroAll", "Message Queue"=w664) -> ("error out"=w662:errorcluster, "dup Message Queue"=w663:refnum<queue>)  [unwired: 7 in]
      }
      event "Enable Platform": Value Change {
        n530 = event-data() -> ()  [unwired: 1 in, 1 out]
        n531 = call-poly "Enqueue Message.vi"("Priority Message? (F)"=TRUE, "Message"="Enable Platform", "Message Queue"=w669) -> ("error out"=w667:errorcluster, "dup Message Queue"=w668:refnum<queue>)  [unwired: 7 in]
      }
      event "Heave Up main": Value Change {
        n532 = event-data() -> ()  [unwired: 1 in, 1 out]
        n533 = call-poly "Enqueue Message.vi"("Priority Message? (F)"=TRUE, "Message"="Heave Up main", "Message Queue"=w674) -> ("error out"=w672:errorcluster, "dup Message Queue"=w673:refnum<queue>)  [unwired: 7 in]
      }
      event "Heave Down Main": Value Change {
        n534 = event-data() -> ()  [unwired: 1 in, 1 out]
        n535 = call-poly "Enqueue Message.vi"("Priority Message? (F)"=TRUE, "Message"="Heave Down Main", "Message Queue"=w679) -> ("error out"=w677:errorcluster, "dup Message Queue"=w678:refnum<queue>)  [unwired: 7 in]
      }
      event "Manual Write Heave & Surge": Value Change {
        n536 = event-data() -> ()  [unwired: 1 in, 1 out]
        n537 = call-poly "Enqueue Message.vi"("Priority Message? (F)"=TRUE, "Message"="Manual Write Heave & Surge", "Message Queue"=w684) -> ("error out"=w682:errorcluster, "dup Message Queue"=w683:refnum<queue>)  [unwired: 7 in]
      }
      event "Surge Backward Main": Value Change {
        n538 = event-data() -> ()  [unwired: 1 in, 1 out]
        n539 = call-poly "Enqueue Message.vi"("Priority Message? (F)"=TRUE, "Message"="Surge Backward Main", "Message Queue"=w689) -> ("error out"=w687:errorcluster, "dup Message Queue"=w688:refnum<queue>)  [unwired: 7 in]
      }
      event "Surge Forward Main": Value Change {
        n540 = event-data() -> ()  [unwired: 1 in, 1 out]
        n541 = call-poly "Enqueue Message.vi"("Priority Message? (F)"=TRUE, "Message"="Surge Forward Main", "Message Queue"=w694) -> ("error out"=w692:errorcluster, "dup Message Queue"=w693:refnum<queue>)  [unwired: 7 in]
      }
      event "Load En": Value Change {
        n542 = event-data() -> ()  [unwired: 1 in, 1 out]
        n543 = call-poly "Enqueue Message.vi"("Priority Message? (F)"=TRUE, "Message"="Load En", "Message Queue"=w699) -> ("error out"=w697:errorcluster, "dup Message Queue"=w698:refnum<queue>)  [unwired: 7 in]
      }
      event "apply load": Value Change {
        n544 = event-data() -> ()  [unwired: 1 in, 1 out]
        n545 = call-poly "Enqueue Message.vi"("Priority Message? (F)"=TRUE, "Message"="apply load", "Message Queue"=w704) -> ("error out"=w702:errorcluster, "dup Message Queue"=w703:refnum<queue>)  [unwired: 7 in]
      }
      event "BACK": Value Change {
        n546 = event-data() -> ()  [unwired: 1 in, 1 out]
        n547 = call-poly "Enqueue Message.vi"("Priority Message? (F)"=TRUE, "Message"="BACK", "Message Queue"=w709) -> ("error out"=w707:errorcluster, "dup Message Queue"=w708:refnum<queue>)  [unwired: 7 in]
      }
      event "Start Test": Value Change {
        n548 = event-data() -> ()  [unwired: 1 in, 1 out]
        n549 = call-poly "Enqueue Message.vi"("Priority Message? (F)"=TRUE, "Message"="Start Test", "Message Queue"=w714) -> ("error out"=w712:errorcluster, "dup Message Queue"=w713:refnum<queue>)  [unwired: 7 in]
      }
      event "STOP": Value Change {
        n550 = event-data() -> ()  [unwired: 1 in, 1 out]
        n551 = call-poly "Enqueue Message.vi"("Priority Message? (F)"=TRUE, "Message"="STOP", "Message Queue"=w719) -> ("error out"=w717:errorcluster, "dup Message Queue"=w718:refnum<queue>)  [unwired: 7 in]
      }
      event Application Instance Close {
        # "#CodeRecommended - When a project closes, all VIs within that project are aborted and leave memory. However, any code placed in this event frame is guaranteed to run to completion, so add any cleanup code that absolutely must happen here."
        n552 = event-data() -> ()  [unwired: 1 in, 1 out]
      }
      event "EXIT": Value Change {
        n553 = event-data() -> ()  [unwired: 1 in, 1 out]
        n554 = call-poly "Enqueue Message.vi"("Priority Message? (F)"=TRUE, "Message"="Exit", "Message Queue"=w727) -> ("error out"=w726:errorcluster, "dup Message Queue"=w725:refnum<queue>)  [unwired: 7 in]
      }
      event User Event {
        # "The Message Handling Loop processed an \"Exit\" message, which fired this event to stop the Event Handling Loop."
        n555 = event-data() -> ()  [unwired: 1 in, 1 out]
      }
    }
    n556 = call "LAB-IQ Error Handler - Event Handling Loop.vi"("error in (no error)"=w537, "Message Queue"=w535) -> ("dup error in"=w534:errorcluster)  [unwired: 8 in, 1 out]
  }
  n557 = disable-structure shown="Disabled" {
    disable-tunnel: [w734 _] -> w31
    disable-tunnel: w6 -> [w733 _]
    disable-tunnel: w25 -> [w732 _]
    disable-tunnel: w17 -> [w731 _]
    disable-tunnel: w13 -> [w730 _]
    frame Disabled {
      n558 = while {
        shift-right: [w745] -> _
        shift-left: w733 -> [w746]
        tunnel: [w739] -> w734
        tunnel: w731 -> [w737]
        tunnel: w730 -> [w736]
        tunnel: w732 -> [w735]
        stop <- w744 stop-if-true
        # "Heave Motor  Handling Loop"
        n559 = call "Dequeue Message.vi"("error in (no error)"=w736, "Message Queue"=w737) -> ("error out"=w743:errorcluster, "Message Data"=w741:variant, "Message"=w742:string, "dup Message Queue"=w740:refnum<queue>)  [unwired: 6 in]
        n560 = case "Message Cases" shown="\"init\"" w742 {
          selector: w742 -> [_ _ _ _ _ w826]
          tunnel: w740 -> [w756 w783 _ w814 w825 _]
          tunnel: w743 -> [w749 w781 w804 w817 w819 _]
          tunnel: [w750 w784 w798 w805 w821 w827] -> w738
          tunnel: w746 -> [w747 w773 w803 w808 w824 w828]
          tunnel: [w747 w773 w803 w808 w824 w828] -> w745
          tunnel: [_ _ _ _ TRUE _] -> w744
          tunnel: w741 -> [_ _ w802 _ _ _]
          tunnel: w735 -> [_ _ _ _ w818 _]
          frame "init" {
            # "Initialize - All initialization work should take place in this message, since other loops can potentially enqueue messages that execute immediately after this one."
            n561 = call "HEAVE WRITE FGV.vi"("Enum - Menu"=Heave_Write_enum."INIT", "error in (no error)"=w749, "main ref"=w747) -> ("error out"=w755:errorcluster)  [unwired: 8 in]
            n562 = call "Stall Data Flow.vim"("value in"=w755, "milliseconds to wait"=u32 1000) -> ("value out"=w753:errorcluster)  [unwired: 1 out]
            n563 = disable-structure shown="Enabled" {
              disable-tunnel: w753 -> [w769 w770]
              disable-tunnel: [w768 w770] -> w748
              disable-tunnel: w747 -> [w767 _]
              frame Disabled {
                n564 = call "Heave Init.vi"("error in (no error)"=w769, "main ref"=w767) -> ("error out"=w768:errorcluster)  [unwired: 9 in]
              }
              frame Enabled {
              }
            }
            n565 = disable-structure shown="Enabled" {
              disable-tunnel: [w760 w763] -> w751
              disable-tunnel: w748 -> [w759 w762]
              disable-tunnel: w747 -> [w758 _]
              frame Disabled {
                n566 = call "HEAVE READ FGV.vi"("Enum - Menu"=Heave_Right_enum."INIT", "error in (no error)"=w759, "main ref"=w758) -> ("error out"=w760:errorcluster)  [unwired: 7 in, 1 out]
              }
              frame Enabled {
                n567 = UDP Open(8:w762, 9:-1 ("timeout ms (25000)"), 10:"192.168.1.10" ("service name"), 11:u16 8889 ("port")) -> (0:w763:errorcluster)  [unwired: 1 in, 2 out]
              }
            }
            n568 = call-poly "Enqueue Message.vi"("error in (no error)"=w751, "Message"="Heave Main", "Message Queue"=w756) -> ("error out"=w750:errorcluster)  [unwired: 7 in, 1 out]
          }
          frame "Heave Main" {
            n569 = Unbundle By Name(w773) -> ("Heave AND Surge.Read Heave Temp"=w776:refnum<vi>)
            n570 = property class="Bool (strict)"(reference=w776) -> (reference out=w774:refnum<vi>, error out=w775:errorcluster, "Value"=w772:bool)  [unwired: 1 in]
            n571 = Close Reference(reference=w774, error in (no error)=w775) -> ()  [unwired: 1 out]
            n572 = case shown="True" w772 {
              tunnel: w781 -> [w785 w789]
              tunnel: [w785 w788] -> w777
              tunnel: w773 -> [_ w787]
              frame False {
              }
              frame True {
                n573 = call "HEAVE READ FGV.vi"("Enum - Menu"=Heave_Right_enum."READ", "error in (no error)"=w789, "main ref"=w787) -> ("error out"=w788:errorcluster)  [unwired: 7 in, 1 out]
              }
            }
            n574 = Unbundle By Name(w773) -> ("Main Home Screen.EXIT"=w782:refnum<vi>)
            n575 = property class="Bool (strict)"(reference=w782) -> (reference out=w779:refnum<vi>, error out=w780:errorcluster, "Value"=w778:bool)  [unwired: 1 in]
            n576 = call <vilib>:"Clear Errors.vi"("error in (no error)"=w777) -> ("error out"=w771:errorcluster)  [unwired: 5 in, 1 out]
            n577 = Close Reference(reference=w779, error in (no error)=w780) -> ()  [unwired: 1 out]
            n578 = case shown="False" w778 {
              tunnel: [w792 w796] -> w784
              tunnel: w783 -> [w791 w795]
              tunnel: w771 -> [w790 w794]
              frame True {
                n579 = call-poly "Enqueue Message.vi"("error in (no error)"=w790, "Message"="Confirm Quit", "Message Queue"=w791) -> ("error out"=w792:errorcluster)  [unwired: 7 in, 1 out]
              }
              frame False {
                n580 = call-poly "Enqueue Message.vi"("error in (no error)"=w794, "Message"="Heave Main", "Message Queue"=w795) -> ("error out"=w796:errorcluster)  [unwired: 7 in, 1 out]
              }
            }
          }
          frame "Error" {
            # "#CodeRecommended - If you ever change the name of this \"Error\" message, you'll need to update the name in the Check Loop Error.vi as well."
            # "#CodeRecommended - Consider creating a system for logging errors in some way. These errors are for notification purposes only. Handling of specific errors should be performed in the message frames that generated the error."
            # "Error - Display an error dialog. This message is sent by the \"Error Handler\" VIs at the end of other loops in this application."
            n581 = Variant To Data(error in=w804, type=errorcluster {"status"=FALSE, "code"=0, "source"=""} ("error constant"), Variant=w802) -> (data=w800:errorcluster, error out=w799:errorcluster)
            n582 = call <vilib>:"Simple Error Handler.vi"("error in (no error)"=w800) -> ()  [unwired: 4 in, 5 out]
            n583 = Merge Errors(w799) -> (w798:errorcluster)
          }
          frame "Confirm Quit" {
            # "#CodeNeeded - If you want to provide an \"Are you sure\" dialog (or some other notification) before the application exits, place that code here. This message is typically sent from a Panel Close? event."
            # "Confirm Quit - Message that can confirm whether or not the user wants to exit the application."
            n584 = call-poly "Enqueue Message.vi"("Priority Message? (F)"=TRUE, "error in (no error)"=w817, "Message"="Exit", "Message Queue"=w814) -> ("error out"=w815:errorcluster)  [unwired: 6 in, 1 out]
            n585 = Merge Errors(w815) -> (w816:errorcluster)
            n586 = call "HEAVE READ FGV.vi"("Enum - Menu"=Heave_Right_enum."CLOSE", "error in (no error)"=w816, "main ref"=w808) -> ("error out"=w811:errorcluster)  [unwired: 7 in, 1 out]
            n587 = call <vilib>:"Clear Errors.vi"("error in (no error)"=w811) -> ("error out"=w806:errorcluster)  [unwired: 5 in, 1 out]
            n588 = call "HEAVE WRITE FGV.vi"("Enum - Menu"=Heave_Write_enum."CLOSE", "error in (no error)"=w806, "main ref"=w808) -> ("error out"=w809:errorcluster)  [unwired: 8 in]
            n589 = call <vilib>:"Clear Errors.vi"("error in (no error)"=w809) -> ("error out"=w805:errorcluster)  [unwired: 5 in, 1 out]
          }
          frame "Exit" {
            # "Stop the VI"
            # "Release the message queue reference"
            # "#CodeNeeded - Add any required cleanup code here. Note that if 'Exit' was called as a result of an error, an error dialog will be displayed. Add any custom error handling for an 'Exit' condition here as well."
            # "Exit - Exit the application."
            n590 = call "Fire User Event - Stop.vi"("User Event - Stop"=w818) -> ("error out"=w820:errorcluster)  [unwired: 10 in]
            n591 = Release Queue(queue=w825, error in (no error)=w819) -> (error out=w822:errorcluster)  [unwired: 1 in, 2 out]
            n592 = Merge Errors(w820, w822) -> (w821:errorcluster)
          }
          frame Default {
            # "'Default' case only runs if there is a message that isn't defined in any of the other cases.  Output a programming error."
            n593 = xnode "Error Ring"("parameter 0"=w826) -> ("error out"=w827:errorcluster)
          }
        }
        n594 = call "LAB-IQ Error Handler - Message Handling Loop.vi"("error in (no error)"=w738, "Message Queue"=w740) -> ("dup error in"=w739:errorcluster)  [unwired: 8 in, 1 out]
      }
    }
    frame Enabled {
    }
  }
  n595 = while {
    tunnel: w63 -> [w850]
    shift-right: [w857] -> _
    shift-left: w6 -> [w858]
    tunnel: w25 -> [w855]
    tunnel: w56 -> [w854]
    tunnel: [w848] -> w64
    tunnel: w35 -> [w846]
    tunnel: w34 -> [w845]
    tunnel: w17 -> [w844]
    tunnel: w32 -> [w843]
    tunnel: w29 -> [w842]
    tunnel: w28 -> [w841]
    tunnel: w27 -> [w840]
    tunnel: w26 -> [w839]
    tunnel: w24 -> [w838]
    tunnel: w23 -> [w837]
    tunnel: w22 -> [w836]
    stop <- w856 stop-if-true
    # "Message Handling Loop"
    n596 = call "Dequeue Message.vi"("error in (no error)"=w854, "Message Queue"=w850) -> ("error out"=w853:errorcluster, "Message Data"=w851:variant, "Message"=w852:string, "dup Message Queue"=w849:refnum<queue>)  [unwired: 6 in]
    n597 = case "Message Cases" shown="\"init\"" w852 {
      selector: w852 -> [_ _ _ _ _ _ _ _ _ _ _ _ _ _ _ _ _ _ _ _ _ _ _ _ _ _ _ _ _ _ _ _ _ _ _ _ _ _ _ _ w1786]
      tunnel: w849 -> [_ w888 _ _ _ _ _ _ _ _ _ _ _ _ _ _ _ _ _ _ _ _ _ _ _ _ _ _ _ _ _ _ _ _ _ _ _ _ w1774 w1785 _]
      tunnel: w853 -> [w860 w890 w904 w933 w954 w971 w988 w1005 w1026 w1038 w1088 w1093 w1100 w1105 w1170 w1196 w1222 w1253 w1265 w1313 w1333 w1422 w1499 w1538 w1550 w1571 w1600 w1619 w1630 w1641 w1652 w1662 w1674 w1696 w1736 w1751 w1759 w1766 w1777 w1778 _]
      tunnel: [w861 w887 w903 w934 w949 w966 w983 w1000 w1021 w1030 w1066 w1091 w1098 w1109 w1166 w1192 w1218 w1254 w1266 w1277 w1324 w1413 w1498 w1537 w1549 w1570 w1587 w1621 w1632 w1643 w1654 w1664 w1673 w1695 w1734 w1749 w1757 w1760 w1769 w1781 w1787] -> w847
      tunnel: w858 -> [w859 w862 w905 w932 w940 w957 w974 w991 w1009 w1028 w1043 w1090 w1096 w1104 w1168 w1194 w1220 w1244 w1256 w1268 w1317 w1405 w1493 w1536 w1548 w1564 w1582 w1617 w1628 w1639 w1650 w1661 w1672 w1694 w1715 w1740 w1752 w1765 w1767 w1784 w1788]
      tunnel: [w859 w862 w905 w932 w940 w957 w974 w991 w1009 w1028 w1043 w1090 w1096 w1104 w1168 w1194 w1220 w1244 w1256 w1268 w1317 w1405 w1493 w1536 w1548 w1564 w1582 w1617 w1628 w1639 w1650 w1661 w1672 w1694 w1715 w1740 w1752 w1765 w1767 w1784 w1788] -> w857
      tunnel: [_ _ _ _ _ _ _ _ _ _ _ _ _ _ _ _ _ _ _ _ _ _ _ _ _ _ _ _ _ _ _ _ _ _ _ _ _ _ _ TRUE _] -> w856
      tunnel: w851 -> [_ _ _ _ _ _ _ _ _ _ _ _ _ _ _ _ _ _ _ _ _ _ _ _ _ _ _ _ _ _ _ _ _ _ _ _ _ w1764 _ _ _]
      tunnel: w855 -> [_ _ _ _ _ _ _ _ _ _ _ _ _ _ _ _ _ _ _ _ _ _ _ _ _ _ _ _ _ _ _ _ _ _ _ _ _ _ _ w1780 _]
      tunnel: w846 -> [_ _ w902 _ _ _ _ _ _ _ _ _ _ _ _ _ _ _ _ _ _ _ _ _ _ _ _ _ _ _ _ _ _ _ _ _ _ _ _ _ _]
      tunnel: w845 -> [_ _ w901 _ _ _ _ _ _ _ _ _ _ _ _ _ _ _ _ _ _ _ _ _ _ _ _ _ _ _ _ _ _ _ _ _ _ _ _ _ _]
      tunnel: w844 -> [_ _ w900 _ _ _ _ _ _ _ _ _ _ _ _ _ _ _ _ _ _ _ _ _ _ _ _ _ _ _ _ _ _ _ _ _ _ _ _ _ _]
      tunnel: w843 -> [_ _ w899 _ _ _ _ _ _ _ _ _ _ _ _ _ _ _ _ _ _ _ _ _ _ _ _ _ _ _ _ _ _ _ _ _ _ _ _ _ _]
      tunnel: w842 -> [_ _ w898 _ _ _ _ _ _ _ _ _ _ _ _ _ _ _ _ _ _ _ _ _ _ _ _ _ _ _ _ _ _ _ _ _ _ _ _ _ _]
      tunnel: w841 -> [_ _ w897 _ _ _ _ _ _ _ _ _ _ _ _ _ _ _ _ _ _ _ _ _ _ _ _ _ _ _ _ _ _ _ _ _ _ _ _ _ _]
      tunnel: w840 -> [_ _ w896 _ _ _ _ _ _ _ _ _ _ _ _ _ _ _ _ _ _ _ _ _ _ _ _ _ _ _ _ _ _ _ _ _ _ _ _ _ _]
      tunnel: w839 -> [_ _ w895 _ _ _ _ _ _ _ _ _ _ _ _ _ _ _ _ _ _ _ _ _ _ _ _ _ _ _ _ _ _ _ _ _ _ _ _ _ _]
      tunnel: w838 -> [_ _ w894 _ _ _ _ _ _ _ _ _ _ _ _ _ _ _ _ _ _ _ _ _ _ _ _ _ _ _ _ _ _ _ _ _ _ _ _ _ _]
      tunnel: w837 -> [_ _ w893 _ _ _ _ _ _ _ _ _ _ _ _ _ _ _ _ _ _ _ _ _ _ _ _ _ _ _ _ _ _ _ _ _ _ _ _ _ _]
      tunnel: w836 -> [_ _ w892 _ _ _ _ _ _ _ _ _ _ _ _ _ _ _ _ _ _ _ _ _ _ _ _ _ _ _ _ _ _ _ _ _ _ _ _ _ _]
      frame "Time Out" {
        n598 = call "Pulse_mm conversion loop.vi"("error in (no error)"=w860, "main ref"=w859) -> ("error out"=w861:errorcluster)  [unwired: 9 in]
        n599 = call "Load Commiunication Error.vi"("error in (no error)"=w860, "main ref"=w859) -> ()  [unwired: 9 in, 1 out]
      }
      frame "init" {
        # "Initialize - All initialization work should take place in this message, since other loops can potentially enqueue messages that execute immediately after this one."
        n600 = call-poly "Enqueue Message.vi"("error in (no error)"=w890, "Message"="Init Other Loop", "Message Queue"=w888) -> ("error out"=w891:errorcluster)  [unwired: 7 in, 1 out]
        n601 = Unbundle By Name(w862) -> ("Loading.Communication is established"=w863:refnum<vi>)
        n602 = Unbundle By Name(w862) -> ("Loading Com Port.Load Cell Temp"=w882:refnum<vi>)
        n603 = Unbundle By Name(w862) -> ("Loading.SSP 0.3"=w876:refnum<vi>)
        n604 = Unbundle By Name(w862) -> ("Loading.SSP 0.5"=w873:refnum<vi>)
        n605 = Unbundle By Name(w862) -> ("Loading.SSP 0.75"=w868:refnum<vi>)
        n606 = call "Read Config Unitest.vi"("error in (no error)"=w891, "main ref"=w862) -> ("error out"=w886:errorcluster)  [unwired: 9 in]
        n607 = call "Encrypt file path creation.vi"("error in (no error)"=w886) -> ("error out"=w885:errorcluster, "File Path"=w884:path)  [unwired: 9 in]
        n608 = property class="Bool (strict)"(reference=w882, "Value"=FALSE) -> (reference out=w880:refnum<vi>, error out=w881:errorcluster)  [unwired: 1 in]
        n609 = property class="Bool (strict)"(reference=w873, "Visible"=FALSE) -> (reference out=w871:refnum<vi>, error out=w872:errorcluster)  [unwired: 1 in]
        n610 = property class="Bool (strict)"(reference=w876, "Visible"=FALSE) -> (reference out=w878:refnum<vi>, error out=w877:errorcluster)  [unwired: 1 in]
        n611 = property class="Bool (strict)"(reference=w868, "Visible"=FALSE) -> (reference out=w870:refnum<vi>, error out=w869:errorcluster)  [unwired: 1 in]
        n612 = property class="Bool (strict)"(reference=w863, "Visible"=FALSE ("Value")) -> (reference out=w865:refnum<vi>, error out=w864:errorcluster)  [unwired: 1 in]
        n613 = call "DATA ENCRYPT STRING FILE WRITE.vi"("file path (dialog if empty)"=w884, "error in (no error)"=w885, "User Action"="System Booted", "main ref"=w862) -> ("error out"=w887:errorcluster)  [unwired: 5 in, 1 out]
        n614 = Close Reference(reference=w871, error in (no error)=w872) -> ()  [unwired: 1 out]
        n615 = Close Reference(reference=w878, error in (no error)=w877) -> ()  [unwired: 1 out]
        n616 = Close Reference(reference=w870, error in (no error)=w869) -> ()  [unwired: 1 out]
        n617 = Close Reference(reference=w880, error in (no error)=w881) -> ()  [unwired: 1 out]
        n618 = Close Reference(reference=w865, error in (no error)=w864) -> ()  [unwired: 1 out]
      }
      frame "Init Other Loop" {
        n619 = disable-structure shown="Disabled" {
          disable-tunnel: w904 -> [w929 w930]
          disable-tunnel: [w918 w930] -> w903
          disable-tunnel: w902 -> [w916 _]
          disable-tunnel: w901 -> [w915 _]
          disable-tunnel: w900 -> [w914 _]
          disable-tunnel: w899 -> [w913 _]
          disable-tunnel: w898 -> [w912 _]
          disable-tunnel: w897 -> [w911 _]
          disable-tunnel: w896 -> [w910 _]
          disable-tunnel: w895 -> [w909 _]
          disable-tunnel: w894 -> [w908 _]
          disable-tunnel: w893 -> [w907 _]
          disable-tunnel: w892 -> [w906 _]
          frame Disabled {
            w917 = "Init" ("Message")
            n620 = call-poly "Enqueue Message.vi"("error in (no error)"=w929, "Message"=w917, "Message Queue"=w916) -> ("error out"=w928:errorcluster)  [unwired: 7 in, 1 out]
            n621 = call-poly "Enqueue Message.vi"("error in (no error)"=w928, "Message"=w917, "Message Queue"=w915) -> ("error out"=w927:errorcluster)  [unwired: 7 in, 1 out]
            n622 = call-poly "Enqueue Message.vi"("error in (no error)"=w927, "Message"=w917, "Message Queue"=w914) -> ("error out"=w926:errorcluster)  [unwired: 7 in, 1 out]
            n623 = call-poly "Enqueue Message.vi"("error in (no error)"=w926, "Message"=w917, "Message Queue"=w913) -> ("error out"=w925:errorcluster)  [unwired: 7 in, 1 out]
            n624 = call-poly "Enqueue Message.vi"("error in (no error)"=w925, "Message"=w917, "Message Queue"=w912) -> ("error out"=w924:errorcluster)  [unwired: 7 in, 1 out]
            n625 = call-poly "Enqueue Message.vi"("error in (no error)"=w924, "Message"=w917, "Message Queue"=w911) -> ("error out"=w923:errorcluster)  [unwired: 7 in, 1 out]
            n626 = call-poly "Enqueue Message.vi"("error in (no error)"=w923, "Message"=w917, "Message Queue"=w910) -> ("error out"=w922:errorcluster)  [unwired: 7 in, 1 out]
            n627 = call-poly "Enqueue Message.vi"("error in (no error)"=w922, "Message"=w917, "Message Queue"=w909) -> ("error out"=w921:errorcluster)  [unwired: 7 in, 1 out]
            n628 = call-poly "Enqueue Message.vi"("error in (no error)"=w921, "Message"=w917, "Message Queue"=w908) -> ("error out"=w920:errorcluster)  [unwired: 7 in, 1 out]
            n629 = call-poly "Enqueue Message.vi"("error in (no error)"=w920, "Message"=w917, "Message Queue"=w907) -> ("error out"=w919:errorcluster)  [unwired: 7 in, 1 out]
            n630 = call-poly "Enqueue Message.vi"("error in (no error)"=w919, "Message"=w917, "Message Queue"=w906) -> ("error out"=w918:errorcluster)  [unwired: 7 in, 1 out]
          }
          frame Enabled {
          }
        }
      }
      frame "Service Save" {
        n631 = call "Write Config Unitest.vi"("error in (no error)"=w933, "main ref"=w932) -> ("error out"=w938:errorcluster)  [unwired: 9 in]
        n632 = call "Stall Data Flow.vim"("value in"=w938, "milliseconds to wait"=u32 2000) -> ("value out"=w937:errorcluster)  [unwired: 1 out]
        n633 = call "Read Config Unitest.vi"("error in (no error)"=w937, "main ref"=w932) -> ("error out"=w935:errorcluster)  [unwired: 9 in]
        n634 = call "DATA ENCRYPT STRING FILE WRITE.vi"("error in (no error)"=w935, "User Action"="Service Parameter Saved", "main ref"=w932) -> ("error out"=w934:errorcluster)  [unwired: 6 in, 1 out]
      }
      frame "HOME" {
        n635 = call "DATA ENCRYPT STRING FILE WRITE.vi"("error in (no error)"=w954, "User Action"="User Pressed Home", "main ref"=w940) -> ("error out"=w950:errorcluster)  [unwired: 6 in, 1 out]
        n636 = Unbundle By Name(w940) -> ("Main Home Screen.MainPage"=w945:refnum<vi>)
        n637 = Unbundle By Name(w940) -> ("Main Home Screen.Home"=w953:refnum<vi>)
        n638 = Unbundle By Name(w940) -> ("Main Home Screen.GUI"=w943:refnum<vi>)
        n639 = property class="Bool (strict)"(reference=w953, error in=w950, "Value"=FALSE) -> (reference out=w951:refnum<vi>, error out=w952:errorcluster)
        n640 = property class="TabCtl (strict)"(reference=w945, "Value"=T5."HOME") -> (reference out=w947:refnum<vi>, error out=w946:errorcluster)  [unwired: 1 in]
        n641 = property class="TabCtl (strict)"(reference=w943, "Value"=T4."Setup") -> (reference out=w941:refnum<vi>, error out=w942:errorcluster)  [unwired: 1 in]
        n642 = Close Reference(reference=w951, error in (no error)=w952) -> (error out=w949:errorcluster)
        n643 = Close Reference(reference=w947, error in (no error)=w946) -> ()  [unwired: 1 out]
        n644 = Close Reference(reference=w941, error in (no error)=w942) -> ()  [unwired: 1 out]
      }
      frame "Platform Setting" {
        n645 = call "DATA ENCRYPT STRING FILE WRITE.vi"("error in (no error)"=w971, "User Action"="User Pressed Platform Setting", "main ref"=w957) -> ("error out"=w967:errorcluster)  [unwired: 6 in, 1 out]
        n646 = Unbundle By Name(w957) -> ("Main Home Screen.Platform Settings"=w970:refnum<vi>)
        n647 = Unbundle By Name(w957) -> ("Main Home Screen.MainPage"=w962:refnum<vi>)
        n648 = Unbundle By Name(w957) -> ("Main Home Screen.GUI"=w960:refnum<vi>)
        n649 = property class="TabCtl (strict)"(reference=w962, "Value"=T5."PlatformSetting") -> (reference out=w964:refnum<vi>, error out=w963:errorcluster)  [unwired: 1 in]
        n650 = property class="TabCtl (strict)"(reference=w960, "Value"=T4."Setup") -> (reference out=w958:refnum<vi>, error out=w959:errorcluster)  [unwired: 1 in]
        n651 = property class="Bool (strict)"(reference=w970, error in=w967, "Value"=FALSE) -> (reference out=w968:refnum<vi>, error out=w969:errorcluster)
        n652 = Close Reference(reference=w964, error in (no error)=w963) -> ()  [unwired: 1 out]
        n653 = Close Reference(reference=w958, error in (no error)=w959) -> ()  [unwired: 1 out]
        n654 = Close Reference(reference=w968, error in (no error)=w969) -> (error out=w966:errorcluster)
      }
      frame "Configure" {
        n655 = call "DATA ENCRYPT STRING FILE WRITE.vi"("error in (no error)"=w988, "User Action"="User Pressed Configure", "main ref"=w974) -> ("error out"=w984:errorcluster)  [unwired: 6 in, 1 out]
        n656 = Unbundle By Name(w974) -> ("Main Home Screen.Configure"=w987:refnum<vi>)
        n657 = Unbundle By Name(w974) -> ("Main Home Screen.MainPage"=w979:refnum<vi>)
        n658 = Unbundle By Name(w974) -> ("Main Home Screen.GUI"=w977:refnum<vi>)
        n659 = property class="Bool (strict)"(reference=w987, error in=w984, "Value"=FALSE) -> (reference out=w985:refnum<vi>, error out=w986:errorcluster)
        n660 = property class="TabCtl (strict)"(reference=w979, "Value"=T5."Details") -> (reference out=w981:refnum<vi>, error out=w980:errorcluster)  [unwired: 1 in]
        n661 = property class="TabCtl (strict)"(reference=w977, "Value"=T4."Setup") -> (reference out=w975:refnum<vi>, error out=w976:errorcluster)  [unwired: 1 in]
        n662 = Close Reference(reference=w985, error in (no error)=w986) -> (error out=w983:errorcluster)
        n663 = Close Reference(reference=w981, error in (no error)=w980) -> ()  [unwired: 1 out]
        n664 = Close Reference(reference=w975, error in (no error)=w976) -> ()  [unwired: 1 out]
      }
      frame "Analysis" {
        n665 = call "DATA ENCRYPT STRING FILE WRITE.vi"("error in (no error)"=w1005, "User Action"="User Pressed Analysis", "main ref"=w991) -> ("error out"=w1001:errorcluster)  [unwired: 6 in, 1 out]
        n666 = Unbundle By Name(w991) -> ("Main Home Screen.MainPage"=w996:refnum<vi>)
        n667 = Unbundle By Name(w991) -> ("Main Home Screen.Analysis"=w1004:refnum<vi>)
        n668 = Unbundle By Name(w991) -> ("Main Home Screen.GUI"=w994:refnum<vi>)
        n669 = property class="Bool (strict)"(reference=w1004, error in=w1001, "Value"=FALSE) -> (reference out=w1002:refnum<vi>, error out=w1003:errorcluster)
        n670 = property class="TabCtl (strict)"(reference=w996, "Value"=T5."Analysis") -> (reference out=w998:refnum<vi>, error out=w997:errorcluster)  [unwired: 1 in]
        n671 = property class="TabCtl (strict)"(reference=w994, "Value"=T4."Setup") -> (reference out=w992:refnum<vi>, error out=w993:errorcluster)  [unwired: 1 in]
        n672 = Close Reference(reference=w1002, error in (no error)=w1003) -> (error out=w1000:errorcluster)
        n673 = Close Reference(reference=w998, error in (no error)=w997) -> ()  [unwired: 1 out]
        n674 = Close Reference(reference=w992, error in (no error)=w993) -> ()  [unwired: 1 out]
      }
      frame "service 2" {
        n675 = call "DATA ENCRYPT STRING FILE WRITE.vi"("error in (no error)"=w1026, "User Action"="User Pressed service", "main ref"=w1009) -> ("error out"=w1022:errorcluster)  [unwired: 6 in, 1 out]
        n676 = Unbundle By Name(w1009) -> ("Main Screen.Main Screen Tab"=w1010:refnum<vi>)
        n677 = Unbundle By Name(w1009) -> ("Main Home Screen.MainPage"=w1017:refnum<vi>)
        n678 = Unbundle By Name(w1009) -> ("Main Home Screen.Analysis"=w1025:refnum<vi>)
        n679 = Unbundle By Name(w1009) -> ("Main Home Screen.GUI"=w1015:refnum<vi>)
        n680 = property class="Bool (strict)"(reference=w1025, error in=w1022, "Value"=FALSE) -> (reference out=w1023:refnum<vi>, error out=w1024:errorcluster)
        n681 = property class="TabCtl (strict)"(reference=w1017, "Value"=T5."HOME") -> (reference out=w1019:refnum<vi>, error out=w1018:errorcluster)  [unwired: 1 in]
        n682 = property class="TabCtl (strict)"(reference=w1015, "Value"=T4."Begin") -> (reference out=w1013:refnum<vi>, error out=w1014:errorcluster)  [unwired: 1 in]
        n683 = property class="TabCtl (strict)"(reference=w1010, "Value"=T8."About") -> (reference out=w1007:refnum<vi>, error out=w1011:errorcluster)  [unwired: 1 in]
        n684 = Close Reference(reference=w1023, error in (no error)=w1024) -> (error out=w1021:errorcluster)
        n685 = Close Reference(reference=w1019, error in (no error)=w1018) -> ()  [unwired: 1 out]
        n686 = Close Reference(reference=w1013, error in (no error)=w1014) -> ()  [unwired: 1 out]
        n687 = Close Reference(reference=w1007, error in (no error)=w1011) -> ()  [unwired: 1 out]
      }
      frame "Auto" {
        n688 = call "DATA ENCRYPT STRING FILE WRITE.vi"("error in (no error)"=w1038, "User Action"="User Pressed Auto File Name", "main ref"=w1028) -> ("error out"=w1035:errorcluster)  [unwired: 6 in, 1 out]
        n689 = Get Date/Time In Seconds() -> (seconds since 1Jan1904=w1036:timestamp)
        n690 = Format Into String(format string="%<%I_%M_%S_%p_%d_%B_%Y>T", error in=w1035, w1036) -> (resulting string=w1029:string, error out=w1031:errorcluster)  [unwired: 1 in]
        n691 = Unbundle By Name(w1028) -> ("Config Screen.FILE"=w1034:refnum<vi>)
        n692 = property class="Str"(reference=w1034, error in=w1031, "Value"=w1029) -> (reference out=w1032:refnum<vi>, error out=w1033:errorcluster)
        n693 = Close Reference(reference=w1032, error in (no error)=w1033) -> (error out=w1030:errorcluster)
      }
      frame "Select Load Head" {
        n694 = Unbundle By Name(w1043) -> ("Loading.Enter the Loading Rate (N/min)"=w1064:refnum<vi>)
        n695 = Unbundle By Name(w1043) -> ("Loading.Communication is established"=w1049:refnum<vi>)
        n696 = call "DATA ENCRYPT STRING FILE WRITE.vi"("error in (no error)"=w1088, "User Action"="User Pressed Select Load Head", "main ref"=w1043) -> ("error out"=w1084:errorcluster)  [unwired: 6 in, 1 out]
        n697 = Unbundle By Name(w1043) -> ("Loading.Enter the Final Load (N)"=w1059:refnum<vi>)
        n698 = Unbundle By Name(w1043) -> ("Loading.DecaForce COM Status"=w1045:refnum<vi>)
        n699 = Unbundle By Name(w1043) -> ("Loading.Loading Mode"=w1087:refnum<vi>)
        n700 = Unbundle By Name(w1043) -> ("Config Screen.Select Load Head"=w1071:refnum<vi>)
        n701 = Unbundle By Name(w1043) -> ("Loading.Warning"=w1054:refnum<vi>)
        n702 = Unbundle By Name(w1043) -> ("Loading.Load Selection"=w1080:refnum<vi>)
        n703 = property class="Bool (strict)"(reference=w1071, "Value"=FALSE) -> (reference out=w1069:refnum<vi>, error out=w1070:errorcluster)  [unwired: 1 in]
        n704 = property class="TabCtl (strict)"(reference=w1080, "Value"=T6."Constant") -> (reference out=w1082:refnum<vi>, error out=w1081:errorcluster)  [unwired: 1 in]
        n705 = property class="Ring (strict)"(reference=w1087, error in=w1084, "Value"=u16 0) -> (reference out=w1085:refnum<vi>, error out=w1086:errorcluster)
        n706 = property class="DigNum (strict)"(reference=w1064, "DisabledEnum"=T15."Disabled and Grayed Out" ("Disabled")) -> (reference out=w1063:refnum<vi>, error out=w1065:errorcluster)  [unwired: 1 in]
        n707 = property class="DigNum (strict)"(reference=w1059, "DisabledEnum"=T15."Disabled and Grayed Out" ("Disabled")) -> (reference out=w1060:refnum<vi>, error out=w1058:errorcluster)  [unwired: 1 in]
        n708 = property class="TabCtl (strict)"(reference=w1054, "Visible"=FALSE) -> (reference out=w1053:refnum<vi>, error out=w1055:errorcluster)  [unwired: 1 in]
        n709 = property class="Bool (strict)"(reference=w1049, "Visible"=FALSE) -> (reference out=w1047:refnum<vi>, error out=w1048:errorcluster)  [unwired: 1 in]
        n710 = property class="Bool (strict)"(reference=w1045, "Visible"=FALSE) -> (reference out=w1040:refnum<vi>, error out=w1046:errorcluster)  [unwired: 1 in]
        n711 = Close Reference(reference=w1069, error in (no error)=w1070) -> (error out=w1067:errorcluster)
        n712 = Close Reference(reference=w1082, error in (no error)=w1081) -> (error out=w1073:errorcluster)
        n713 = Close Reference(reference=w1085, error in (no error)=w1086) -> (error out=w1075:errorcluster)
        n714 = Close Reference(reference=w1063, error in (no error)=w1065) -> (error out=w1057:errorcluster)
        n715 = Close Reference(reference=w1060, error in (no error)=w1058) -> (error out=w1056:errorcluster)
        n716 = Close Reference(reference=w1053, error in (no error)=w1055) -> (error out=w1052:errorcluster)
        n717 = Close Reference(reference=w1047, error in (no error)=w1048) -> (error out=w1042:errorcluster)
        n718 = Close Reference(reference=w1040, error in (no error)=w1046) -> (error out=w1041:errorcluster)
        n719 = Merge Errors(w1075, w1073, w1067, w1057, w1056, w1052, w1042, w1041) -> (w1074:errorcluster)
        n720 = Unbundle By Name(w1043) -> ("Main Home Screen.GUI"=w1076:refnum<vi>)
        n721 = property class="TabCtl (strict)"(reference=w1076, error in=w1074, "Value"=T4."Load Head") -> (reference out=w1078:refnum<vi>, error out=w1077:errorcluster)
        n722 = Close Reference(reference=w1078, error in (no error)=w1077) -> (error out=w1066:errorcluster)
      }
      frame "com 3" {
        n723 = call "DATA ENCRYPT STRING FILE WRITE.vi"("error in (no error)"=w1093, "User Action"="User Pressed Check Load Communication", "main ref"=w1090) -> ("error out"=w1092:errorcluster)  [unwired: 6 in, 1 out]
        n724 = call "SET LOAD PARAMETERS.vi"("error in (no error)"=w1092, "main ref"=w1090) -> ("error out"=w1091:errorcluster)  [unwired: 9 in]
      }
      frame "ZeroAll" {
        n725 = call "DATA ENCRYPT STRING FILE WRITE.vi"("error in (no error)"=w1100, "User Action"="User Pressed Zero All", "main ref"=w1096) -> ("error out"=w1099:errorcluster)  [unwired: 6 in, 1 out]
        n726 = local write "ZeroAll"(FALSE ("ZeroAll")) -> ()
        n727 = call "LOAD CELL FGV MAIN.vi"("Enum"=T16."ZEROALL", "error in (no error)"=w1099, "main ref"=w1096) -> ("error IO"=w1098:errorcluster)  [unwired: 8 in]
      }
      frame "Loading Mode" {
        n728 = Unbundle By Name(w1104) -> ("Loading.Loading Mode"=w1106:refnum<vi>)
        n729 = property class="Ring (strict)"(reference=w1106, error in=w1105) -> (reference out=w1108:refnum<vi>, error out=w1107:errorcluster, "Value"=w1102:u16)
        n730 = Close Reference(reference=w1108, error in (no error)=w1107) -> (error out=w1103:errorcluster)
        n731 = case shown="1" w1102 {
          tunnel: [w1123 w1140 w1152 w1164] -> w1109
          tunnel: w1104 -> [w1110 w1126 w1144 w1156]
          tunnel: w1103 -> [w1124 w1139 w1151 w1163]
          frame 0, Default {
            n732 = Unbundle By Name(w1110) -> ("Loading.Enter the Loading Rate (N/min)"=w1117:refnum<vi>)
            n733 = Unbundle By Name(w1110) -> ("Loading.Load Selection"=w1120:refnum<vi>)
            n734 = Unbundle By Name(w1110) -> ("Loading.Enter the Final Load (N)"=w1112:refnum<vi>)
            n735 = property class="TabCtl (strict)"(reference=w1120, "Value"=T6."Constant") -> (reference out=w1122:refnum<vi>, error out=w1121:errorcluster)  [unwired: 1 in]
            n736 = property class="DigNum (strict)"(reference=w1117, "DisabledEnum"=T15."Disabled and Grayed Out" ("Disabled")) -> (reference out=w1116:refnum<vi>, error out=w1118:errorcluster)  [unwired: 1 in]
            n737 = property class="DigNum (strict)"(reference=w1112, "DisabledEnum"=T15."Disabled and Grayed Out" ("Disabled")) -> (reference out=w1113:refnum<vi>, error out=w1111:errorcluster)  [unwired: 1 in]
            n738 = call "DATA ENCRYPT STRING FILE WRITE.vi"("error in (no error)"=w1124, "User Action"="User selected Constant Mode", "main ref"=w1110) -> ("error out"=w1123:errorcluster)  [unwired: 6 in, 1 out]
            n739 = Close Reference(reference=w1122, error in (no error)=w1121) -> ()  [unwired: 1 out]
            n740 = Close Reference(reference=w1116, error in (no error)=w1118) -> ()  [unwired: 1 out]
            n741 = Close Reference(reference=w1113, error in (no error)=w1111) -> ()  [unwired: 1 out]
          }
          frame 1 {
            n742 = Unbundle By Name(w1126) -> ("Loading.Enter the Loading Rate (N/min)"=w1137:refnum<vi>)
            n743 = Unbundle By Name(w1126) -> ("Loading.Enter the Final Load (N)"=w1132:refnum<vi>)
            n744 = Unbundle By Name(w1126) -> ("Loading.Load Selection"=w1128:refnum<vi>)
            n745 = property class="TabCtl (strict)"(reference=w1128, "Value"=T6."Constant") -> (reference out=w1130:refnum<vi>, error out=w1129:errorcluster)  [unwired: 1 in]
            n746 = property class="DigNum (strict)"(reference=w1137, "DisabledEnum"=T15."Enabled" ("Disabled")) -> (reference out=w1136:refnum<vi>, error out=w1138:errorcluster)  [unwired: 1 in]
            n747 = property class="DigNum (strict)"(reference=w1132, "DisabledEnum"=T15."Enabled" ("Disabled")) -> (reference out=w1133:refnum<vi>, error out=w1131:errorcluster)  [unwired: 1 in]
            n748 = call "DATA ENCRYPT STRING FILE WRITE.vi"("error in (no error)"=w1139, "User Action"="User selected Ramp Mode", "main ref"=w1126) -> ("error out"=w1140:errorcluster)  [unwired: 6 in, 1 out]
            n749 = Close Reference(reference=w1130, error in (no error)=w1129) -> ()  [unwired: 1 out]
            n750 = Close Reference(reference=w1136, error in (no error)=w1138) -> ()  [unwired: 1 out]
            n751 = Close Reference(reference=w1133, error in (no error)=w1131) -> ()  [unwired: 1 out]
          }
          frame 2 {
            n752 = Unbundle By Name(w1144) -> ("Loading.Load Selection"=w1148:refnum<vi>)
            n753 = Unbundle By Name(w1144) -> ("Loading.Warning 2"=w1146:refnum<vi>)
            n754 = property class="TabCtl (strict)"(reference=w1148, "Value"=T6."Step") -> (reference out=w1150:refnum<vi>, error out=w1149:errorcluster)  [unwired: 1 in]
            n755 = property class="Bool (strict)"(reference=w1146, "Visible"=FALSE) -> (reference out=w1142:refnum<vi>, error out=w1145:errorcluster)  [unwired: 1 in]
            n756 = call "DATA ENCRYPT STRING FILE WRITE.vi"("error in (no error)"=w1151, "User Action"="User selected Step Mode", "main ref"=w1144) -> ("error out"=w1152:errorcluster)  [unwired: 6 in, 1 out]
            n757 = Close Reference(reference=w1150, error in (no error)=w1149) -> ()  [unwired: 1 out]
            n758 = Close Reference(reference=w1142, error in (no error)=w1145) -> ()  [unwired: 1 out]
          }
          frame 3 {
            n759 = Unbundle By Name(w1156) -> ("Loading.Load Selection"=w1160:refnum<vi>)
            n760 = Unbundle By Name(w1156) -> ("Loading.Warning 2"=w1158:refnum<vi>)
            n761 = property class="TabCtl (strict)"(reference=w1160, "Value"=T6."Indentation") -> (reference out=w1162:refnum<vi>, error out=w1161:errorcluster)  [unwired: 1 in]
            n762 = property class="Bool (strict)"(reference=w1158, "Visible"=FALSE) -> (reference out=w1154:refnum<vi>, error out=w1157:errorcluster)  [unwired: 1 in]
            n763 = call "DATA ENCRYPT STRING FILE WRITE.vi"("error in (no error)"=w1163, "User Action"="User selected Indentation Mode", "main ref"=w1156) -> ("error out"=w1164:errorcluster)  [unwired: 6 in, 1 out]
            n764 = Close Reference(reference=w1162, error in (no error)=w1161) -> ()  [unwired: 1 out]
            n765 = Close Reference(reference=w1154, error in (no error)=w1157) -> ()  [unwired: 1 out]
          }
        }
      }
      frame "SSP 0.3" {
        n766 = Unbundle By Name(w1168) -> ("Loading.SSP 0.3"=w1171:refnum<vi>)
        n767 = property class="Bool (strict)"(reference=w1171, error in=w1170) -> (reference out=w1173:refnum<vi>, error out=w1172:errorcluster, "Value"=w1169:bool)
        n768 = Close Reference(reference=w1173, error in (no error)=w1172) -> (error out=w1167:errorcluster)
        n769 = case shown="True" w1169 {
          tunnel: w1168 -> [_ w1175]
          tunnel: w1167 -> [w1174 w1183]
          tunnel: [w1174 w1182] -> w1166
          frame False {
          }
          frame True {
            w1185 = FALSE ("Value")
            n770 = Unbundle By Name(w1175) -> ("Loading.Enter the Load  (N)"=w1181:refnum<vi>)
            n771 = Unbundle By Name(w1175) -> ("Loading.SSP 0.75"=w1186:refnum<vi>)
            n772 = Unbundle By Name(w1175) -> ("Loading.SSP 0.5"=w1191:refnum<vi>)
            n773 = property class="Bool (strict)"(reference=w1186, "Value"=w1185) -> (reference out=w1188:refnum<vi>, error out=w1187:errorcluster)  [unwired: 1 in]
            n774 = property class="Bool (strict)"(reference=w1191, "Value"=w1185) -> (reference out=w1189:refnum<vi>, error out=w1190:errorcluster)  [unwired: 1 in]
            n775 = property class="DigNum (strict)"(reference=w1181, "Minimum"=2.0 ("Data Entry Limits:Minimum"), "Maximum"=50.0 ("Data Entry Limits:Maximum"), "Increment"=0.1 ("Data Entry Limits:Increment")) -> (reference out=w1179:refnum<vi>, error out=w1180:errorcluster)  [unwired: 1 in]
            n776 = call "DATA ENCRYPT STRING FILE WRITE.vi"("error in (no error)"=w1183, "User Action"="User selected 0.3 SSP", "main ref"=w1175) -> ("error out"=w1182:errorcluster)  [unwired: 6 in, 1 out]
            n777 = Close Reference(reference=w1188, error in (no error)=w1187) -> ()  [unwired: 1 out]
            n778 = Close Reference(reference=w1189, error in (no error)=w1190) -> ()  [unwired: 1 out]
            n779 = Close Reference(reference=w1179, error in (no error)=w1180) -> ()  [unwired: 1 out]
          }
        }
      }
      frame "SSP 0.5" {
        n780 = Unbundle By Name(w1194) -> ("Loading.SSP 0.5"=w1197:refnum<vi>)
        n781 = property class="Bool (strict)"(reference=w1197, error in=w1196) -> (reference out=w1199:refnum<vi>, error out=w1198:errorcluster, "Value"=w1195:bool)
        n782 = Close Reference(reference=w1199, error in (no error)=w1198) -> (error out=w1193:errorcluster)
        n783 = case shown="True" w1195 {
          tunnel: w1194 -> [_ w1201]
          tunnel: w1193 -> [w1200 w1209]
          tunnel: [w1200 w1208] -> w1192
          frame False {
          }
          frame True {
            w1211 = FALSE ("Value")
            n784 = Unbundle By Name(w1201) -> ("Loading.Enter the Load  (N)"=w1207:refnum<vi>)
            n785 = Unbundle By Name(w1201) -> ("Loading.SSP 0.75"=w1217:refnum<vi>)
            n786 = Unbundle By Name(w1201) -> ("Loading.SSP 0.3"=w1212:refnum<vi>)
            n787 = property class="Bool (strict)"(reference=w1212, "Value"=w1211) -> (reference out=w1214:refnum<vi>, error out=w1213:errorcluster)  [unwired: 1 in]
            n788 = property class="Bool (strict)"(reference=w1217, "Value"=w1211) -> (reference out=w1215:refnum<vi>, error out=w1216:errorcluster)  [unwired: 1 in]
            n789 = property class="DigNum (strict)"(reference=w1207, "Minimum"=2.0 ("Data Entry Limits:Minimum"), "Maximum"=200.0 ("Data Entry Limits:Maximum"), "Increment"=0.1 ("Data Entry Limits:Increment")) -> (reference out=w1205:refnum<vi>, error out=w1206:errorcluster)  [unwired: 1 in]
            n790 = call "DATA ENCRYPT STRING FILE WRITE.vi"("error in (no error)"=w1209, "User Action"="User selected 0.5 SSP", "main ref"=w1201) -> ("error out"=w1208:errorcluster)  [unwired: 6 in, 1 out]
            n791 = Close Reference(reference=w1214, error in (no error)=w1213) -> ()  [unwired: 1 out]
            n792 = Close Reference(reference=w1215, error in (no error)=w1216) -> ()  [unwired: 1 out]
            n793 = Close Reference(reference=w1205, error in (no error)=w1206) -> ()  [unwired: 1 out]
          }
        }
      }
      frame "SSP 0.75" {
        n794 = Unbundle By Name(w1220) -> ("Loading.SSP 0.75"=w1223:refnum<vi>)
        n795 = property class="Bool (strict)"(reference=w1223, error in=w1222) -> (reference out=w1225:refnum<vi>, error out=w1224:errorcluster, "Value"=w1221:bool)
        n796 = Close Reference(reference=w1225, error in (no error)=w1224) -> (error out=w1219:errorcluster)
        n797 = case shown="True" w1221 {
          tunnel: w1220 -> [_ w1227]
          tunnel: w1219 -> [w1226 w1235]
          tunnel: [w1226 w1234] -> w1218
          frame False {
          }
          frame True {
            w1237 = FALSE ("Value")
            n798 = Unbundle By Name(w1227) -> ("Loading.SSP 0.3"=w1238:refnum<vi>)
            n799 = Unbundle By Name(w1227) -> ("Loading.SSP 0.5"=w1243:refnum<vi>)
            n800 = Unbundle By Name(w1227) -> ("Loading.Enter the Load  (N)"=w1233:refnum<vi>)
            n801 = property class="Bool (strict)"(reference=w1238, "Value"=w1237) -> (reference out=w1240:refnum<vi>, error out=w1239:errorcluster)  [unwired: 1 in]
            n802 = property class="Bool (strict)"(reference=w1243, "Value"=w1237) -> (reference out=w1241:refnum<vi>, error out=w1242:errorcluster)  [unwired: 1 in]
            n803 = property class="DigNum (strict)"(reference=w1233, "Minimum"=200.0 ("Data Entry Limits:Minimum"), "Maximum"=500.0 ("Data Entry Limits:Maximum"), "Increment"=0.1 ("Data Entry Limits:Increment")) -> (reference out=w1231:refnum<vi>, error out=w1232:errorcluster)  [unwired: 1 in]
            n804 = call "DATA ENCRYPT STRING FILE WRITE.vi"("error in (no error)"=w1235, "User Action"="User selected 0.75 SSP", "main ref"=w1227) -> ("error out"=w1234:errorcluster)  [unwired: 6 in, 1 out]
            n805 = Close Reference(reference=w1240, error in (no error)=w1239) -> ()  [unwired: 1 out]
            n806 = Close Reference(reference=w1241, error in (no error)=w1242) -> ()  [unwired: 1 out]
            n807 = Close Reference(reference=w1231, error in (no error)=w1232) -> ()  [unwired: 1 out]
          }
        }
      }
      frame "LHBack" {
        # "Back to Configure"
        n808 = Unbundle By Name(w1244) -> ("Main Home Screen.GUI"=w1250:refnum<vi>)
        n809 = Unbundle By Name(w1244) -> ("Main Home Screen.MainPage"=w1246:refnum<vi>)
        n810 = property class="TabCtl (strict)"(reference=w1246, "Value"=T5."HOME") -> (reference out=w1248:refnum<vi>, error out=w1247:errorcluster)  [unwired: 1 in]
        n811 = property class="TabCtl (strict)"(reference=w1250, "Value"=T4."Setup") -> (reference out=w1252:refnum<vi>, error out=w1251:errorcluster)  [unwired: 1 in]
        n812 = Close Reference(reference=w1248, error in (no error)=w1247) -> ()  [unwired: 1 out]
        n813 = Close Reference(reference=w1252, error in (no error)=w1251) -> ()  [unwired: 1 out]
        n814 = call "DATA ENCRYPT STRING FILE WRITE.vi"("error in (no error)"=w1253, "User Action"="User selected Back to Configure", "main ref"=w1244) -> ("error out"=w1254:errorcluster)  [unwired: 6 in, 1 out]
      }
      frame "MMBack" {
        # "Back to Configure"
        n815 = Unbundle By Name(w1256) -> ("Main Home Screen.GUI"=w1262:refnum<vi>)
        n816 = Unbundle By Name(w1256) -> ("Main Home Screen.MainPage"=w1258:refnum<vi>)
        n817 = property class="TabCtl (strict)"(reference=w1258, "Value"=T5."HOME") -> (reference out=w1260:refnum<vi>, error out=w1259:errorcluster)  [unwired: 1 in]
        n818 = property class="TabCtl (strict)"(reference=w1262, "Value"=T4."Load Head") -> (reference out=w1264:refnum<vi>, error out=w1263:errorcluster)  [unwired: 1 in]
        n819 = Close Reference(reference=w1260, error in (no error)=w1259) -> ()  [unwired: 1 out]
        n820 = Close Reference(reference=w1264, error in (no error)=w1263) -> ()  [unwired: 1 out]
        n821 = call "DATA ENCRYPT STRING FILE WRITE.vi"("error in (no error)"=w1265, "User Action"="User selected Back to Load Selection", "main ref"=w1256) -> ("error out"=w1266:errorcluster)  [unwired: 6 in, 1 out]
      }
      frame "LHNext" {
        w1298 = FALSE ("Visible")
        n822 = Unbundle By Name(w1268) -> ("Motion Module.HomeRot"=w1304:refnum<vi>)
        n823 = Unbundle By Name(w1268) -> ("Motion Module.HomeScratch"=w1299:refnum<vi>)
        n824 = Unbundle By Name(w1268) -> ("Motion Module.PlaceModule"=w1297:refnum<vi>)
        n825 = Unbundle By Name(w1268) -> ("Motion Module.Motion Mode:"=w1290:refnum<vi>)
        n826 = Unbundle By Name(w1268) -> ("Motion Module.Motion Direction:  3"=w1289:refnum<vi>)
        n827 = Unbundle By Name(w1268) -> ("Motion Module.Wear Track Diameter (mm)"=w1283:refnum<vi>)
        n828 = Unbundle By Name(w1268) -> ("Motion Module.Set WTD"=w1280:refnum<vi>)
        n829 = Unbundle By Name(w1268) -> ("Motion Module.Rotary Module Selection"=w1274:refnum<vi>)
        n830 = call "DATA ENCRYPT STRING FILE WRITE.vi"("error in (no error)"=w1313, "User Action"="User selected Select Module", "main ref"=w1268) -> ("error out"=w1277:errorcluster)  [unwired: 6 in, 1 out]
        n831 = property class="TabCtl (strict)"(reference=w1274, "Visible"=FALSE) -> (reference out=w1273:refnum<vi>, error out=w1275:errorcluster)  [unwired: 1 in]
        n832 = property class="Bool (strict)"(reference=w1304, error in=w1277, "Visible"=w1298) -> (reference out=w1302:refnum<vi>, error out=w1303:errorcluster)
        n833 = property class="Bool (strict)"(reference=w1299, error in=w1277, "Visible"=w1298) -> (reference out=w1301:refnum<vi>, error out=w1300:errorcluster)
        n834 = property class="Bool (strict)"(reference=w1297, error in=w1277, "Visible"=TRUE) -> (reference out=w1295:refnum<vi>, error out=w1296:errorcluster)
        n835 = property class="Ring (strict)"(reference=w1290, error in=w1277, "Visible"=FALSE) -> (reference out=w1292:refnum<vi>, error out=w1291:errorcluster)
        n836 = property class="Ring (strict)"(reference=w1289, error in=w1277, "Visible"=FALSE) -> (reference out=w1286:refnum<vi>, error out=w1288:errorcluster)
        n837 = property class="DigNum (strict)"(reference=w1283, "Visible"=FALSE) -> (reference out=w1282:refnum<vi>, error out=w1284:errorcluster)  [unwired: 1 in]
        n838 = property class="Bool (strict)"(reference=w1280, "Visible"=FALSE) -> (reference out=w1281:refnum<vi>, error out=w1279:errorcluster)  [unwired: 1 in]
        n839 = Close Reference(reference=w1302, error in (no error)=w1303) -> ()  [unwired: 1 out]
        n840 = Close Reference(reference=w1301, error in (no error)=w1300) -> ()  [unwired: 1 out]
        n841 = Close Reference(reference=w1295, error in (no error)=w1296) -> ()  [unwired: 1 out]
        n842 = Close Reference(reference=w1292, error in (no error)=w1291) -> ()  [unwired: 1 out]
        n843 = Close Reference(reference=w1286, error in (no error)=w1288) -> ()  [unwired: 1 out]
        n844 = Close Reference(reference=w1282, error in (no error)=w1284) -> ()  [unwired: 1 out]
        n845 = Close Reference(reference=w1273, error in (no error)=w1275) -> ()  [unwired: 1 out]
        n846 = Close Reference(reference=w1281, error in (no error)=w1279) -> ()  [unwired: 1 out]
        n847 = Unbundle By Name(w1268) -> ("Motion Module.M3 Image"=w1272:refnum<vi>)
        n848 = Unbundle By Name(w1268) -> ("Main Home Screen.GUI"=w1310:refnum<vi>)
        n849 = Unbundle By Name(w1268) -> ("Main Home Screen.MainPage"=w1306:refnum<vi>)
        n850 = property class="TabCtl (strict)"(reference=w1272, "Value"=enum32{"Page 1", "Page 2"}."Page 2") -> (reference out=w1270:refnum<vi>, error out=w1271:errorcluster)  [unwired: 1 in]
        n851 = property class="TabCtl (strict)"(reference=w1306, "Value"=T5."HOME") -> (reference out=w1308:refnum<vi>, error out=w1307:errorcluster)  [unwired: 1 in]
        n852 = property class="TabCtl (strict)"(reference=w1310, "Value"=T4."Motion Module") -> (reference out=w1312:refnum<vi>, error out=w1311:errorcluster)  [unwired: 1 in]
        n853 = Close Reference(reference=w1270, error in (no error)=w1271) -> ()  [unwired: 1 out]
        n854 = Close Reference(reference=w1308, error in (no error)=w1307) -> ()  [unwired: 1 out]
        n855 = Close Reference(reference=w1312, error in (no error)=w1311) -> ()  [unwired: 1 out]
      }
      frame "Rot Ver" {
        # "Rot Ver"
        n856 = Unbundle By Name(w1317) -> ("Motion Module.Rot Ver"=w1316:refnum<vi>)
        n857 = property class="Bool (strict)"(reference=w1316) -> (reference out=w1319:refnum<vi>, error out=w1318:errorcluster, "Value"=w1315:bool)  [unwired: 1 in]
        n858 = Close Reference(reference=w1319, error in (no error)=w1318) -> ()  [unwired: 1 out]
        n859 = case shown="True" w1315 {
          tunnel: w1333 -> [w1368 w1403]
          tunnel: [w1340 w1403] -> w1324
          tunnel: w1317 -> [w1334 w1370]
          frame True {
            n860 = Unbundle By Name(w1334) -> ("Motion Module.HomeRot"=w1367:refnum<vi>)
            n861 = Unbundle By Name(w1334) -> ("Motion Module.HomeScratch"=w1362:refnum<vi>)
            n862 = Unbundle By Name(w1334) -> ("Motion Module.PlaceModule"=w1360:refnum<vi>)
            n863 = Unbundle By Name(w1334) -> ("Motion Module.Motion Mode:"=w1353:refnum<vi>)
            n864 = Unbundle By Name(w1334) -> ("Motion Module.Motion Direction:  3"=w1352:refnum<vi>)
            n865 = Unbundle By Name(w1334) -> ("Motion Module.Wear Track Diameter (mm)"=w1346:refnum<vi>)
            n866 = Unbundle By Name(w1334) -> ("Motion Module.Set WTD"=w1343:refnum<vi>)
            n867 = Unbundle By Name(w1334) -> ("Motion Module.Rotary Module Selection"=w1337:refnum<vi>)
            n868 = call "DATA ENCRYPT STRING FILE WRITE.vi"("error in (no error)"=w1368, "User Action"="User selected Rot Vertical Module", "main ref"=w1334) -> ("error out"=w1340:errorcluster)  [unwired: 6 in, 1 out]
            n869 = property class="TabCtl (strict)"(reference=w1337, "Visible"=TRUE) -> (reference out=w1336:refnum<vi>, error out=w1338:errorcluster)  [unwired: 1 in]
            n870 = property class="Bool (strict)"(reference=w1367, error in=w1340, "Visible"=TRUE) -> (reference out=w1365:refnum<vi>, error out=w1366:errorcluster)
            n871 = property class="Bool (strict)"(reference=w1362, error in=w1340, "Visible"=FALSE) -> (reference out=w1364:refnum<vi>, error out=w1363:errorcluster)
            n872 = property class="Bool (strict)"(reference=w1360, error in=w1340, "Visible"=FALSE) -> (reference out=w1358:refnum<vi>, error out=w1359:errorcluster)
            n873 = property class="Ring (strict)"(reference=w1353, error in=w1340, "Visible"=TRUE) -> (reference out=w1355:refnum<vi>, error out=w1354:errorcluster)
            n874 = property class="Ring (strict)"(reference=w1352, error in=w1340, "Visible"=TRUE) -> (reference out=w1349:refnum<vi>, error out=w1351:errorcluster)
            n875 = property class="DigNum (strict)"(reference=w1346, "Visible"=TRUE) -> (reference out=w1345:refnum<vi>, error out=w1347:errorcluster)  [unwired: 1 in]
            n876 = property class="Bool (strict)"(reference=w1343, "Visible"=TRUE) -> (reference out=w1344:refnum<vi>, error out=w1342:errorcluster)  [unwired: 1 in]
            n877 = Close Reference(reference=w1365, error in (no error)=w1366) -> ()  [unwired: 1 out]
            n878 = Close Reference(reference=w1364, error in (no error)=w1363) -> ()  [unwired: 1 out]
            n879 = Close Reference(reference=w1358, error in (no error)=w1359) -> ()  [unwired: 1 out]
            n880 = Close Reference(reference=w1355, error in (no error)=w1354) -> ()  [unwired: 1 out]
            n881 = Close Reference(reference=w1349, error in (no error)=w1351) -> ()  [unwired: 1 out]
            n882 = Close Reference(reference=w1345, error in (no error)=w1347) -> ()  [unwired: 1 out]
            n883 = Close Reference(reference=w1336, error in (no error)=w1338) -> ()  [unwired: 1 out]
            n884 = Close Reference(reference=w1344, error in (no error)=w1342) -> ()  [unwired: 1 out]
          }
          frame False {
            n885 = Unbundle By Name(w1370) -> ("Motion Module.HomeRot"=w1402:refnum<vi>)
            n886 = Unbundle By Name(w1370) -> ("Motion Module.HomeScratch"=w1397:refnum<vi>)
            n887 = Unbundle By Name(w1370) -> ("Motion Module.PlaceModule"=w1395:refnum<vi>)
            n888 = Unbundle By Name(w1370) -> ("Motion Module.Motion Mode:"=w1388:refnum<vi>)
            n889 = Unbundle By Name(w1370) -> ("Motion Module.Motion Direction:  3"=w1387:refnum<vi>)
            n890 = Unbundle By Name(w1370) -> ("Motion Module.Wear Track Diameter (mm)"=w1381:refnum<vi>)
            n891 = Unbundle By Name(w1370) -> ("Motion Module.Set WTD"=w1378:refnum<vi>)
            n892 = Unbundle By Name(w1370) -> ("Motion Module.Rotary Module Selection"=w1373:refnum<vi>)
            n893 = property class="TabCtl (strict)"(reference=w1373, "Visible"=FALSE) -> (reference out=w1372:refnum<vi>, error out=w1374:errorcluster)  [unwired: 1 in]
            n894 = property class="Bool (strict)"(reference=w1402, error in=w1403, "Visible"=FALSE) -> (reference out=w1400:refnum<vi>, error out=w1401:errorcluster)
            n895 = property class="Bool (strict)"(reference=w1397, error in=w1403, "Visible"=FALSE) -> (reference out=w1399:refnum<vi>, error out=w1398:errorcluster)
            n896 = property class="Bool (strict)"(reference=w1395, error in=w1403, "Visible"=TRUE) -> (reference out=w1393:refnum<vi>, error out=w1394:errorcluster)
            n897 = property class="Ring (strict)"(reference=w1388, error in=w1403, "Visible"=FALSE) -> (reference out=w1390:refnum<vi>, error out=w1389:errorcluster)
            n898 = property class="Ring (strict)"(reference=w1387, error in=w1403, "Visible"=FALSE) -> (reference out=w1384:refnum<vi>, error out=w1386:errorcluster)
            n899 = property class="DigNum (strict)"(reference=w1381, "Visible"=FALSE) -> (reference out=w1380:refnum<vi>, error out=w1382:errorcluster)  [unwired: 1 in]
            n900 = property class="Bool (strict)"(reference=w1378, "Visible"=FALSE) -> (reference out=w1379:refnum<vi>, error out=w1377:errorcluster)  [unwired: 1 in]
            n901 = Close Reference(reference=w1400, error in (no error)=w1401) -> ()  [unwired: 1 out]
            n902 = Close Reference(reference=w1399, error in (no error)=w1398) -> ()  [unwired: 1 out]
            n903 = Close Reference(reference=w1393, error in (no error)=w1394) -> ()  [unwired: 1 out]
            n904 = Close Reference(reference=w1390, error in (no error)=w1389) -> ()  [unwired: 1 out]
            n905 = Close Reference(reference=w1384, error in (no error)=w1386) -> ()  [unwired: 1 out]
            n906 = Close Reference(reference=w1380, error in (no error)=w1382) -> ()  [unwired: 1 out]
            n907 = Close Reference(reference=w1372, error in (no error)=w1374) -> ()  [unwired: 1 out]
            n908 = Close Reference(reference=w1379, error in (no error)=w1377) -> ()  [unwired: 1 out]
          }
        }
        n909 = Unbundle By Name(w1317) -> ("Motion Module.M3 Image"=w1323:refnum<vi>)
        n910 = Unbundle By Name(w1317) -> ("Main Home Screen.GUI"=w1330:refnum<vi>)
        n911 = Unbundle By Name(w1317) -> ("Main Home Screen.MainPage"=w1326:refnum<vi>)
        n912 = property class="TabCtl (strict)"(reference=w1323, "Value"=enum32{"Page 1", "Page 2"}."Page 1") -> (reference out=w1321:refnum<vi>, error out=w1322:errorcluster)  [unwired: 1 in]
        n913 = property class="TabCtl (strict)"(reference=w1326, "Value"=T5."HOME") -> (reference out=w1328:refnum<vi>, error out=w1327:errorcluster)  [unwired: 1 in]
        n914 = property class="TabCtl (strict)"(reference=w1330, "Value"=T4."Motion Module") -> (reference out=w1332:refnum<vi>, error out=w1331:errorcluster)  [unwired: 1 in]
        n915 = Close Reference(reference=w1321, error in (no error)=w1322) -> ()  [unwired: 1 out]
        n916 = Close Reference(reference=w1328, error in (no error)=w1327) -> ()  [unwired: 1 out]
        n917 = Close Reference(reference=w1332, error in (no error)=w1331) -> ()  [unwired: 1 out]
      }
      frame "Scratch" {
        n918 = Unbundle By Name(w1405) -> ("Motion Module.Scratch"=w1406:refnum<vi>)
        n919 = property class="Bool (strict)"(reference=w1406) -> (reference out=w1408:refnum<vi>, error out=w1407:errorcluster, "Value"=w1404:bool)  [unwired: 1 in]
        n920 = Close Reference(reference=w1408, error in (no error)=w1407) -> ()  [unwired: 1 out]
        n921 = case shown="True" w1404 {
          tunnel: w1422 -> [w1457 w1492]
          tunnel: [w1429 w1492] -> w1413
          tunnel: w1405 -> [w1423 w1459]
          frame True {
            n922 = Unbundle By Name(w1423) -> ("Motion Module.HomeRot"=w1456:refnum<vi>)
            n923 = Unbundle By Name(w1423) -> ("Motion Module.HomeScratch"=w1451:refnum<vi>)
            n924 = Unbundle By Name(w1423) -> ("Motion Module.PlaceModule"=w1449:refnum<vi>)
            n925 = Unbundle By Name(w1423) -> ("Motion Module.Motion Mode:"=w1442:refnum<vi>)
            n926 = Unbundle By Name(w1423) -> ("Motion Module.Motion Direction:  3"=w1441:refnum<vi>)
            n927 = Unbundle By Name(w1423) -> ("Motion Module.Wear Track Diameter (mm)"=w1435:refnum<vi>)
            n928 = Unbundle By Name(w1423) -> ("Motion Module.Set WTD"=w1432:refnum<vi>)
            n929 = Unbundle By Name(w1423) -> ("Motion Module.Rotary Module Selection"=w1426:refnum<vi>)
            n930 = call "DATA ENCRYPT STRING FILE WRITE.vi"("error in (no error)"=w1457, "User Action"="User selected Scratch Module", "main ref"=w1423) -> ("error out"=w1429:errorcluster)  [unwired: 6 in, 1 out]
            n931 = property class="TabCtl (strict)"(reference=w1426, "Visible"=FALSE) -> (reference out=w1425:refnum<vi>, error out=w1427:errorcluster)  [unwired: 1 in]
            n932 = property class="Bool (strict)"(reference=w1456, error in=w1429, "Visible"=FALSE) -> (reference out=w1454:refnum<vi>, error out=w1455:errorcluster)
            n933 = property class="Bool (strict)"(reference=w1451, error in=w1429, "Visible"=TRUE) -> (reference out=w1453:refnum<vi>, error out=w1452:errorcluster)
            n934 = property class="Bool (strict)"(reference=w1449, error in=w1429, "Visible"=FALSE) -> (reference out=w1447:refnum<vi>, error out=w1448:errorcluster)
            n935 = property class="Ring (strict)"(reference=w1442, error in=w1429, "Visible"=FALSE) -> (reference out=w1444:refnum<vi>, error out=w1443:errorcluster)
            n936 = property class="Ring (strict)"(reference=w1441, error in=w1429, "Visible"=FALSE) -> (reference out=w1438:refnum<vi>, error out=w1440:errorcluster)
            n937 = property class="DigNum (strict)"(reference=w1435, "Visible"=FALSE) -> (reference out=w1434:refnum<vi>, error out=w1436:errorcluster)  [unwired: 1 in]
            n938 = property class="Bool (strict)"(reference=w1432, "Visible"=FALSE) -> (reference out=w1433:refnum<vi>, error out=w1431:errorcluster)  [unwired: 1 in]
            n939 = Close Reference(reference=w1454, error in (no error)=w1455) -> ()  [unwired: 1 out]
            n940 = Close Reference(reference=w1453, error in (no error)=w1452) -> ()  [unwired: 1 out]
            n941 = Close Reference(reference=w1447, error in (no error)=w1448) -> ()  [unwired: 1 out]
            n942 = Close Reference(reference=w1444, error in (no error)=w1443) -> ()  [unwired: 1 out]
            n943 = Close Reference(reference=w1438, error in (no error)=w1440) -> ()  [unwired: 1 out]
            n944 = Close Reference(reference=w1434, error in (no error)=w1436) -> ()  [unwired: 1 out]
            n945 = Close Reference(reference=w1425, error in (no error)=w1427) -> ()  [unwired: 1 out]
            n946 = Close Reference(reference=w1433, error in (no error)=w1431) -> ()  [unwired: 1 out]
          }
          frame False {
            n947 = Unbundle By Name(w1459) -> ("Motion Module.HomeRot"=w1491:refnum<vi>)
            n948 = Unbundle By Name(w1459) -> ("Motion Module.HomeScratch"=w1486:refnum<vi>)
            n949 = Unbundle By Name(w1459) -> ("Motion Module.PlaceModule"=w1484:refnum<vi>)
            n950 = Unbundle By Name(w1459) -> ("Motion Module.Motion Mode:"=w1477:refnum<vi>)
            n951 = Unbundle By Name(w1459) -> ("Motion Module.Motion Direction:  3"=w1476:refnum<vi>)
            n952 = Unbundle By Name(w1459) -> ("Motion Module.Wear Track Diameter (mm)"=w1470:refnum<vi>)
            n953 = Unbundle By Name(w1459) -> ("Motion Module.Set WTD"=w1467:refnum<vi>)
            n954 = Unbundle By Name(w1459) -> ("Motion Module.Rotary Module Selection"=w1462:refnum<vi>)
            n955 = property class="TabCtl (strict)"(reference=w1462, "Visible"=FALSE) -> (reference out=w1461:refnum<vi>, error out=w1463:errorcluster)  [unwired: 1 in]
            n956 = property class="Bool (strict)"(reference=w1491, error in=w1492, "Visible"=FALSE) -> (reference out=w1489:refnum<vi>, error out=w1490:errorcluster)
            n957 = property class="Bool (strict)"(reference=w1486, error in=w1492, "Visible"=FALSE) -> (reference out=w1488:refnum<vi>, error out=w1487:errorcluster)
            n958 = property class="Bool (strict)"(reference=w1484, error in=w1492, "Visible"=TRUE) -> (reference out=w1482:refnum<vi>, error out=w1483:errorcluster)
            n959 = property class="Ring (strict)"(reference=w1477, error in=w1492, "Visible"=FALSE) -> (reference out=w1479:refnum<vi>, error out=w1478:errorcluster)
            n960 = property class="Ring (strict)"(reference=w1476, error in=w1492, "Visible"=FALSE) -> (reference out=w1473:refnum<vi>, error out=w1475:errorcluster)
            n961 = property class="DigNum (strict)"(reference=w1470, "Visible"=FALSE) -> (reference out=w1469:refnum<vi>, error out=w1471:errorcluster)  [unwired: 1 in]
            n962 = property class="Bool (strict)"(reference=w1467, "Visible"=FALSE) -> (reference out=w1468:refnum<vi>, error out=w1466:errorcluster)  [unwired: 1 in]
            n963 = Close Reference(reference=w1489, error in (no error)=w1490) -> ()  [unwired: 1 out]
            n964 = Close Reference(reference=w1488, error in (no error)=w1487) -> ()  [unwired: 1 out]
            n965 = Close Reference(reference=w1482, error in (no error)=w1483) -> ()  [unwired: 1 out]
            n966 = Close Reference(reference=w1479, error in (no error)=w1478) -> ()  [unwired: 1 out]
            n967 = Close Reference(reference=w1473, error in (no error)=w1475) -> ()  [unwired: 1 out]
            n968 = Close Reference(reference=w1469, error in (no error)=w1471) -> ()  [unwired: 1 out]
            n969 = Close Reference(reference=w1461, error in (no error)=w1463) -> ()  [unwired: 1 out]
            n970 = Close Reference(reference=w1468, error in (no error)=w1466) -> ()  [unwired: 1 out]
          }
        }
        n971 = Unbundle By Name(w1405) -> ("Main Home Screen.GUI"=w1419:refnum<vi>)
        n972 = Unbundle By Name(w1405) -> ("Main Home Screen.MainPage"=w1415:refnum<vi>)
        n973 = Unbundle By Name(w1405) -> ("Motion Module.M3 Image"=w1412:refnum<vi>)
        n974 = property class="TabCtl (strict)"(reference=w1415, "Value"=T5."HOME") -> (reference out=w1417:refnum<vi>, error out=w1416:errorcluster)  [unwired: 1 in]
        n975 = property class="TabCtl (strict)"(reference=w1412, "Value"=enum32{"Page 1", "Page 2"}."Page 2") -> (reference out=w1410:refnum<vi>, error out=w1411:errorcluster)  [unwired: 1 in]
        n976 = property class="TabCtl (strict)"(reference=w1419, "Value"=T4."Motion Module") -> (reference out=w1421:refnum<vi>, error out=w1420:errorcluster)  [unwired: 1 in]
        n977 = Close Reference(reference=w1417, error in (no error)=w1416) -> ()  [unwired: 1 out]
        n978 = Close Reference(reference=w1410, error in (no error)=w1411) -> ()  [unwired: 1 out]
        n979 = Close Reference(reference=w1421, error in (no error)=w1420) -> ()  [unwired: 1 out]
      }
      frame "Motion Mode:" {
        n980 = Unbundle By Name(w1493) -> ("Motion Module.Motion Mode:"=w1495:refnum<vi>)
        n981 = property class="Ring (strict)"(reference=w1495) -> (reference out=w1497:refnum<vi>, error out=w1496:errorcluster, "Value"=w1494:u16)  [unwired: 1 in]
        n982 = Close Reference(reference=w1497, error in (no error)=w1496) -> ()  [unwired: 1 out]
        n983 = case shown="3" w1494 {
          tunnel: w1499 -> [w1508 w1517 w1526 w1535]
          tunnel: [w1507 w1516 w1525 w1534] -> w1498
          tunnel: w1493 -> [w1506 w1515 w1524 w1533]
          tunnel: w1493 -> [w1501 w1510 w1519 w1528]
          frame 0, Default {
            n984 = Unbundle By Name(w1501) -> ("Motion Module.Rotary Module Selection"=w1502:refnum<vi>)
            n985 = property class="TabCtl (strict)"(reference=w1502, "Value"=T7."Uniform Rotation") -> (reference out=w1504:refnum<vi>, error out=w1503:errorcluster)  [unwired: 1 in]
            n986 = Close Reference(reference=w1504, error in (no error)=w1503) -> ()  [unwired: 1 out]
            n987 = call "DATA ENCRYPT STRING FILE WRITE.vi"("error in (no error)"=w1508, "User Action"="User Selected Uniform Rotation", "main ref"=w1506) -> ("error out"=w1507:errorcluster)  [unwired: 6 in, 1 out]
          }
          frame 1 {
            n988 = Unbundle By Name(w1510) -> ("Motion Module.Rotary Module Selection"=w1511:refnum<vi>)
            n989 = property class="TabCtl (strict)"(reference=w1511, "Value"=T7."Angular Oscillation") -> (reference out=w1513:refnum<vi>, error out=w1512:errorcluster)  [unwired: 1 in]
            n990 = Close Reference(reference=w1513, error in (no error)=w1512) -> ()  [unwired: 1 out]
            n991 = call "DATA ENCRYPT STRING FILE WRITE.vi"("error in (no error)"=w1517, "User Action"="User Selected Angular Oscillation", "main ref"=w1515) -> ("error out"=w1516:errorcluster)  [unwired: 6 in, 1 out]
          }
          frame 2 {
            n992 = Unbundle By Name(w1519) -> ("Motion Module.Rotary Module Selection"=w1520:refnum<vi>)
            n993 = property class="TabCtl (strict)"(reference=w1520, "Value"=T7."Speed Ramp") -> (reference out=w1522:refnum<vi>, error out=w1521:errorcluster)  [unwired: 1 in]
            n994 = Close Reference(reference=w1522, error in (no error)=w1521) -> ()  [unwired: 1 out]
            n995 = call "DATA ENCRYPT STRING FILE WRITE.vi"("error in (no error)"=w1526, "User Action"="User Selected Ramp Mode", "main ref"=w1524) -> ("error out"=w1525:errorcluster)  [unwired: 6 in, 1 out]
          }
          frame 3 {
            n996 = Unbundle By Name(w1528) -> ("Motion Module.Rotary Module Selection"=w1529:refnum<vi>)
            n997 = property class="TabCtl (strict)"(reference=w1529, "Value"=T7."Speed Step") -> (reference out=w1531:refnum<vi>, error out=w1530:errorcluster)  [unwired: 1 in]
            n998 = Close Reference(reference=w1531, error in (no error)=w1530) -> ()  [unwired: 1 out]
            n999 = call "DATA ENCRYPT STRING FILE WRITE.vi"("error in (no error)"=w1535, "User Action"="User Selected Step Mode", "main ref"=w1533) -> ("error out"=w1534:errorcluster)  [unwired: 6 in, 1 out]
          }
        }
      }
      frame "MMNext" {
        n1000 = Unbundle By Name(w1536) -> ("Motion Module.MMNext"=w1543:refnum<vi>)
        n1001 = Unbundle By Name(w1536) -> ("Main Home Screen.GUI"=w1545:refnum<vi>)
        n1002 = property class="TabCtl (strict)"(reference=w1545, "Value"=T4."Environment") -> (reference out=w1547:refnum<vi>, error out=w1546:errorcluster)  [unwired: 1 in]
        n1003 = property class="Bool (strict)"(reference=w1543, "Value"=FALSE) -> (reference out=w1541:refnum<vi>, error out=w1542:errorcluster)  [unwired: 1 in]
        n1004 = Close Reference(reference=w1541, error in (no error)=w1542) -> ()  [unwired: 1 out]
        n1005 = Close Reference(reference=w1547, error in (no error)=w1546) -> ()  [unwired: 1 out]
        n1006 = call "DATA ENCRYPT STRING FILE WRITE.vi"("error in (no error)"=w1538, "User Action"="User Selected SetUp Module", "main ref"=w1536) -> ("error out"=w1537:errorcluster)  [unwired: 6 in, 1 out]
      }
      frame "APBack" {
        n1007 = Unbundle By Name(w1548) -> ("Environmental control.APBack"=w1555:refnum<vi>)
        n1008 = Unbundle By Name(w1548) -> ("Main Home Screen.GUI"=w1557:refnum<vi>)
        n1009 = property class="TabCtl (strict)"(reference=w1557, "Value"=T4."Motion Module") -> (reference out=w1559:refnum<vi>, error out=w1558:errorcluster)  [unwired: 1 in]
        n1010 = property class="Bool (strict)"(reference=w1555, "Value"=FALSE) -> (reference out=w1553:refnum<vi>, error out=w1554:errorcluster)  [unwired: 1 in]
        n1011 = Close Reference(reference=w1553, error in (no error)=w1554) -> ()  [unwired: 1 out]
        n1012 = Close Reference(reference=w1559, error in (no error)=w1558) -> ()  [unwired: 1 out]
        n1013 = call "DATA ENCRYPT STRING FILE WRITE.vi"("error in (no error)"=w1550, "User Action"="User Selected Back to Module", "main ref"=w1548) -> ("error out"=w1549:errorcluster)  [unwired: 6 in, 1 out]
      }
      frame "SNext" {
        w1563 = FALSE ("Value")
        n1014 = Unbundle By Name(w1564) -> ("Main Screen.Start Test"=w1567:refnum<vi>)
        n1015 = Unbundle By Name(w1564) -> ("Main Screen.STOP"=w1566:refnum<vi>)
        n1016 = Unbundle By Name(w1564) -> ("Environmental control.SNext"=w1576:refnum<vi>)
        n1017 = Unbundle By Name(w1564) -> ("Main Home Screen.GUI"=w1578:refnum<vi>)
        n1018 = property class="Bool (strict)"(reference=w1567, "Visible"=TRUE ("Value"), "Value"=FALSE) -> (reference out=w1561:refnum<vi>, error out=w1568:errorcluster)  [unwired: 1 in]
        n1019 = property class="Bool (strict)"(reference=w1566, "Value"=w1563, "Visible"=w1563) -> (reference out=w1560:refnum<vi>, error out=w1565:errorcluster)  [unwired: 1 in]
        n1020 = property class="TabCtl (strict)"(reference=w1578, "Value"=T4."Begin") -> (reference out=w1580:refnum<vi>, error out=w1579:errorcluster)  [unwired: 1 in]
        n1021 = property class="Bool (strict)"(reference=w1576, "Value"=FALSE) -> (reference out=w1574:refnum<vi>, error out=w1575:errorcluster)  [unwired: 1 in]
        n1022 = Close Reference(reference=w1561, error in (no error)=w1568) -> ()  [unwired: 1 out]
        n1023 = Close Reference(reference=w1560, error in (no error)=w1565) -> ()  [unwired: 1 out]
        n1024 = Close Reference(reference=w1574, error in (no error)=w1575) -> ()  [unwired: 1 out]
        n1025 = Close Reference(reference=w1580, error in (no error)=w1579) -> ()  [unwired: 1 out]
        n1026 = call "DATA ENCRYPT STRING FILE WRITE.vi"("error in (no error)"=w1571, "User Action"="User Pressed Setup", "main ref"=w1564) -> ("error out"=w1570:errorcluster)  [unwired: 6 in, 1 out]
      }
      frame "Enable Platform" {
        n1027 = Unbundle By Name(w1582) -> ("Heave AND Surge.Sequence ID"=w1584:refnum<vi>)
        n1028 = Unbundle By Name(w1582) -> ("Heave AND Surge.Mode Command"=w1608:refnum<vi>)
        n1029 = Unbundle By Name(w1582) -> ("Heave AND Surge.Distance"=w1605:refnum<vi>)
        n1030 = Unbundle By Name(w1582) -> ("Heave AND Surge.SPEED"=w1602:refnum<vi>)
        n1031 = Unbundle By Name(w1582) -> ("Platform Settings.Enable Platform"=w1616:refnum<vi>)
        n1032 = property class="DigNum (strict)"(reference=w1584, "Value"=u16 0) -> (reference out=w1583:refnum<vi>, error out=w1585:errorcluster)  [unwired: 1 in]
        n1033 = property class="DigNum (strict)"(reference=w1605, error in=w1600, "Value"=sgl 0.0) -> (reference out=w1606:refnum<vi>, error out=w1604:errorcluster)
        n1034 = property class="DigNum (strict)"(reference=w1602, error in=w1600, "Value"=sgl 0.0) -> (reference out=w1603:refnum<vi>, error out=w1601:errorcluster)
        n1035 = property class="DigNum (strict)"(reference=w1608, error in=w1600, "Value"=u8 1) -> (reference out=w1607:refnum<vi>, error out=w1609:errorcluster)
        n1036 = Close Reference(reference=w1583, error in (no error)=w1585) -> (error out=w1581:errorcluster)
        n1037 = Close Reference(reference=w1606, error in (no error)=w1604) -> (error out=w1597:errorcluster)
        n1038 = Close Reference(reference=w1603, error in (no error)=w1601) -> (error out=w1596:errorcluster)
        n1039 = Close Reference(reference=w1607, error in (no error)=w1609) -> (error out=w1598:errorcluster)
        n1040 = property class="Bool (strict)"(reference=w1616, "Value"=FALSE) -> (reference out=w1614:refnum<vi>, error out=w1615:errorcluster)  [unwired: 1 in]
        n1041 = Close Reference(reference=w1614, error in (no error)=w1615) -> ()  [unwired: 1 out]
        n1042 = Merge Errors(w1600, w1598, w1597, w1596, w1581) -> (w1599:errorcluster)
        n1043 = call "DATA ENCRYPT STRING FILE WRITE.vi"("error in (no error)"=w1599, "User Action"="User Pressed Enable Platform", "main ref"=w1582) -> ("error out"=w1611:errorcluster)  [unwired: 6 in, 1 out]
        n1044 = call "HEAVE WRITE FGV.vi"("Enum - Menu"=Heave_Write_enum."WRITE", "error in (no error)"=w1611, "main ref"=w1582) -> ("error out"=w1588:errorcluster)  [unwired: 8 in]
        n1045 = Unbundle By Name(w1582) -> ("Heave AND Surge.Read Heave Temp"=w1592:refnum<vi>)
        n1046 = property class="Bool (strict)"(reference=w1592, error in=w1588, "Value"=TRUE) -> (reference out=w1590:refnum<vi>, error out=w1591:errorcluster)
        n1047 = Close Reference(reference=w1590, error in (no error)=w1591) -> (error out=w1587:errorcluster)
      }
      frame "Heave Up main" {
        n1048 = Unbundle By Name(w1617) -> ("Platform Settings.Heave Up main"=w1627:refnum<vi>)
        n1049 = call "Heave Up Main.vi"("error in (no error)"=w1619, "main ref"=w1617) -> ("error out"=w1618:errorcluster)  [unwired: 9 in]
        n1050 = property class="Bool (strict)"(reference=w1627, "Value"=FALSE) -> (reference out=w1625:refnum<vi>, error out=w1626:errorcluster)  [unwired: 1 in]
        n1051 = Close Reference(reference=w1625, error in (no error)=w1626) -> ()  [unwired: 1 out]
        n1052 = call "DATA ENCRYPT STRING FILE WRITE.vi"("error in (no error)"=w1618, "User Action"="User Pressed Heave UP", "main ref"=w1617) -> ("error out"=w1622:errorcluster)  [unwired: 6 in, 1 out]
        n1053 = call "HEAVE WRITE FGV.vi"("Enum - Menu"=Heave_Write_enum."WRITE", "error in (no error)"=w1622, "main ref"=w1617) -> ("error out"=w1621:errorcluster)  [unwired: 8 in]
      }
      frame "Heave Down Main" {
        n1054 = call "Heave Down Main.vi"("error in (no error)"=w1630, "main ref"=w1628) -> ("error out"=w1629:errorcluster)  [unwired: 9 in]
        n1055 = Unbundle By Name(w1628) -> ("Platform Settings.Heave Down Main"=w1638:refnum<vi>)
        n1056 = property class="Bool (strict)"(reference=w1638, "Value"=FALSE) -> (reference out=w1636:refnum<vi>, error out=w1637:errorcluster)  [unwired: 1 in]
        n1057 = Close Reference(reference=w1636, error in (no error)=w1637) -> ()  [unwired: 1 out]
        n1058 = call "DATA ENCRYPT STRING FILE WRITE.vi"("error in (no error)"=w1629, "User Action"="User Pressed Heave DOWN", "main ref"=w1628) -> ("error out"=w1633:errorcluster)  [unwired: 6 in, 1 out]
        n1059 = call "HEAVE WRITE FGV.vi"("Enum - Menu"=Heave_Write_enum."WRITE", "error in (no error)"=w1633, "main ref"=w1628) -> ("error out"=w1632:errorcluster)  [unwired: 8 in]
      }
      frame "Surge Backward Main" {
        n1060 = Unbundle By Name(w1639) -> ("Platform Settings.Surge Backward Main"=w1649:refnum<vi>)
        n1061 = call "Surge Backward Main.vi"("error in (no error)"=w1641, "main ref"=w1639) -> ("error out"=w1640:errorcluster)  [unwired: 9 in]
        n1062 = property class="Bool (strict)"(reference=w1649, "Value"=FALSE) -> (reference out=w1647:refnum<vi>, error out=w1648:errorcluster)  [unwired: 1 in]
        n1063 = Close Reference(reference=w1647, error in (no error)=w1648) -> ()  [unwired: 1 out]
        n1064 = call "DATA ENCRYPT STRING FILE WRITE.vi"("error in (no error)"=w1640, "User Action"="User Pressed Surge Backward", "main ref"=w1639) -> ("error out"=w1644:errorcluster)  [unwired: 6 in, 1 out]
        n1065 = call "HEAVE WRITE FGV.vi"("Enum - Menu"=Heave_Write_enum."WRITE", "error in (no error)"=w1644, "main ref"=w1639) -> ("error out"=w1643:errorcluster)  [unwired: 8 in]
      }
      frame "Surge Forward Main" {
        n1066 = Unbundle By Name(w1650) -> ("Platform Settings.Surge Forward Main"=w1660:refnum<vi>)
        n1067 = call "Surge Forward Main.vi"("error in (no error)"=w1652, "main ref"=w1650) -> ("error out"=w1651:errorcluster)  [unwired: 9 in]
        n1068 = property class="Bool (strict)"(reference=w1660, "Value"=FALSE) -> (reference out=w1658:refnum<vi>, error out=w1659:errorcluster)  [unwired: 1 in]
        n1069 = Close Reference(reference=w1658, error in (no error)=w1659) -> ()  [unwired: 1 out]
        n1070 = call "DATA ENCRYPT STRING FILE WRITE.vi"("error in (no error)"=w1651, "User Action"="User Pressed Surge Forward", "main ref"=w1650) -> ("error out"=w1655:errorcluster)  [unwired: 6 in, 1 out]
        n1071 = call "HEAVE WRITE FGV.vi"("Enum - Menu"=Heave_Write_enum."WRITE", "error in (no error)"=w1655, "main ref"=w1650) -> ("error out"=w1654:errorcluster)  [unwired: 8 in]
      }
      frame "Manual Write Heave & Surge" {
        n1072 = Unbundle By Name(w1661) -> ("Heave AND Surge.Manual Write"=w1670:refnum<vi>)
        n1073 = property class="Bool (strict)"(reference=w1670, "Value"=FALSE) -> (reference out=w1668:refnum<vi>, error out=w1669:errorcluster)  [unwired: 1 in]
        n1074 = Close Reference(reference=w1668, error in (no error)=w1669) -> ()  [unwired: 1 out]
        n1075 = call "DATA ENCRYPT STRING FILE WRITE.vi"("error in (no error)"=w1662, "User Action"="User Pressed Manual Write Heave and Surge", "main ref"=w1661) -> ("error out"=w1665:errorcluster)  [unwired: 6 in, 1 out]
        n1076 = call "HEAVE WRITE FGV.vi"("Enum - Menu"=Heave_Write_enum."WRITE", "error in (no error)"=w1665, "main ref"=w1661) -> ("error out"=w1664:errorcluster)  [unwired: 8 in]
      }
      frame "Load En" {
        n1077 = Unbundle By Name(w1672) -> ("Main Screen.Load En"=w1677:refnum<vi>)
        n1078 = property class="Bool (strict)"(reference=w1677) -> (reference out=w1675:refnum<vi>, error out=w1676:errorcluster, "Value"=w1671:bool)  [unwired: 1 in]
        n1079 = Close Reference(reference=w1675, error in (no error)=w1676) -> ()  [unwired: 1 out]
        n1080 = case shown="False" w1671 {
          tunnel: [w1684 w1691] -> w1673
          tunnel: w1674 -> [w1687 w1690]
          tunnel: w1672 -> [w1686 w1689]
          tunnel: w1672 -> [w1681 _]
          tunnel: w1672 -> [w1680 _]
          frame False {
            n1081 = call "DATA ENCRYPT STRING FILE WRITE.vi"("error in (no error)"=w1687, "User Action"="User Pressed UnLoad on Main Screen", "main ref"=w1686) -> ("error out"=w1683:errorcluster)  [unwired: 6 in, 1 out]
            n1082 = call "Stall Data Flow.vim"("value in"=w1683, "milliseconds to wait"=u32 2000) -> ("value out"=w1679:errorcluster)  [unwired: 1 out]
            n1083 = call "PID UNLOAD.vi"("error in (no error)"=w1679, "main ref"=w1680) -> ("error out"=w1682:errorcluster)  [unwired: 9 in]
            n1084 = call "HEAVE WRITE FGV.vi"("Enum - Menu"=Heave_Write_enum."WRITE", "error in (no error)"=w1682, "main ref"=w1681) -> ("error out"=w1684:errorcluster)  [unwired: 8 in]
          }
          frame True {
            n1085 = call "DATA ENCRYPT STRING FILE WRITE.vi"("error in (no error)"=w1690, "User Action"="User Pressed Load on Main Screen", "main ref"=w1689) -> ("error out"=w1691:errorcluster)  [unwired: 6 in, 1 out]
          }
        }
      }
      frame "apply load" {
        n1086 = Unbundle By Name(w1694) -> ("Main Screen.Load En"=w1699:refnum<vi>)
        n1087 = property class="Bool (strict)"(reference=w1699) -> (reference out=w1697:refnum<vi>, error out=w1698:errorcluster, "Value"=w1693:bool)  [unwired: 1 in]
        n1088 = Close Reference(reference=w1697, error in (no error)=w1698) -> ()  [unwired: 1 out]
        n1089 = case shown="False" w1693 {
          tunnel: [w1706 w1713] -> w1695
          tunnel: w1696 -> [w1709 w1712]
          tunnel: w1694 -> [w1708 w1711]
          tunnel: w1694 -> [w1703 _]
          tunnel: w1694 -> [w1702 _]
          frame False {
            n1090 = call "DATA ENCRYPT STRING FILE WRITE.vi"("error in (no error)"=w1709, "User Action"="User Pressed UnLoad on Service Screen", "main ref"=w1708) -> ("error out"=w1705:errorcluster)  [unwired: 6 in, 1 out]
            n1091 = call "Stall Data Flow.vim"("value in"=w1705, "milliseconds to wait"=u32 2000) -> ("value out"=w1701:errorcluster)  [unwired: 1 out]
            n1092 = call "PID UNLOAD.vi"("error in (no error)"=w1701, "main ref"=w1702) -> ("error out"=w1704:errorcluster)  [unwired: 9 in]
            n1093 = call "HEAVE WRITE FGV.vi"("Enum - Menu"=Heave_Write_enum."WRITE", "error in (no error)"=w1704, "main ref"=w1703) -> ("error out"=w1706:errorcluster)  [unwired: 8 in]
          }
          frame True {
            n1094 = call "DATA ENCRYPT STRING FILE WRITE.vi"("error in (no error)"=w1712, "User Action"="User Pressed Load on Service Screen", "main ref"=w1711) -> ("error out"=w1713:errorcluster)  [unwired: 6 in, 1 out]
          }
        }
      }
      frame "BACK" {
        w1719 = FALSE ("Value")
        n1095 = Unbundle By Name(w1715) -> ("Main Screen.BACK"=w1739:refnum<vi>)
        n1096 = property class="Bool (strict)"(reference=w1739, "Value"=FALSE) -> (reference out=w1737:refnum<vi>, error out=w1738:errorcluster)  [unwired: 1 in]
        n1097 = Close Reference(reference=w1737, error in (no error)=w1738) -> ()  [unwired: 1 out]
        n1098 = call "DATA ENCRYPT STRING FILE WRITE.vi"("error in (no error)"=w1736, "User Action"="User Pressed Back on Main Screen", "main ref"=w1715) -> ("error out"=w1734:errorcluster)  [unwired: 6 in, 1 out]
        n1099 = Unbundle By Name(w1715) -> ("Main Home Screen.MainPage"=w1726:refnum<vi>)
        n1100 = Unbundle By Name(w1715) -> ("Main Screen.Start Test"=w1722:refnum<vi>)
        n1101 = Unbundle By Name(w1715) -> ("Main Screen.STOP"=w1721:refnum<vi>)
        n1102 = Unbundle By Name(w1715) -> ("Main Home Screen.GUI"=w1730:refnum<vi>)
        n1103 = property class="TabCtl (strict)"(reference=w1726, "Value"=T5."HOME") -> (reference out=w1728:refnum<vi>, error out=w1727:errorcluster)  [unwired: 1 in]
        n1104 = property class="TabCtl (strict)"(reference=w1730, "Value"=T4."Setup") -> (reference out=w1732:refnum<vi>, error out=w1731:errorcluster)  [unwired: 1 in]
        n1105 = property class="Bool (strict)"(reference=w1722, "Visible"=TRUE ("Value"), "Value"=FALSE) -> (reference out=w1717:refnum<vi>, error out=w1723:errorcluster)  [unwired: 1 in]
        n1106 = property class="Bool (strict)"(reference=w1721, "Value"=w1719, "Visible"=w1719) -> (reference out=w1716:refnum<vi>, error out=w1720:errorcluster)  [unwired: 1 in]
        n1107 = Close Reference(reference=w1732, error in (no error)=w1731) -> ()  [unwired: 1 out]
        n1108 = Close Reference(reference=w1728, error in (no error)=w1727) -> ()  [unwired: 1 out]
        n1109 = Close Reference(reference=w1717, error in (no error)=w1723) -> ()  [unwired: 1 out]
        n1110 = Close Reference(reference=w1716, error in (no error)=w1720) -> ()  [unwired: 1 out]
      }
      frame "Start Test" {
        n1111 = call "DATA ENCRYPT STRING FILE WRITE.vi"("error in (no error)"=w1751, "User Action"="User Pressed Start Test on Main Screen", "main ref"=w1740) -> ("error out"=w1749:errorcluster)  [unwired: 6 in, 1 out]
        n1112 = Unbundle By Name(w1740) -> ("Main Screen.Start Test Temp"=w1748:refnum<vi>)
        n1113 = Unbundle By Name(w1740) -> ("Main Screen.Depthz"=w1741:refnum<vi>)
        n1114 = property class="Bool (strict)"(reference=w1741, "Value"=TRUE) -> (reference out=w1743:refnum<vi>, error out=w1742:errorcluster)  [unwired: 1 in]
        n1115 = property class="Bool (strict)"(reference=w1748, "Value"=TRUE) -> (reference out=w1746:refnum<vi>, error out=w1747:errorcluster)  [unwired: 1 in]
        n1116 = Close Reference(reference=w1743, error in (no error)=w1742) -> ()  [unwired: 1 out]
        n1117 = Close Reference(reference=w1746, error in (no error)=w1747) -> ()  [unwired: 1 out]
      }
      frame "STOP" {
        n1118 = call "DATA ENCRYPT STRING FILE WRITE.vi"("error in (no error)"=w1759, "User Action"="User Pressed Stop Test on Main Screen", "main ref"=w1752) -> ("error out"=w1757:errorcluster)  [unwired: 6 in, 1 out]
        n1119 = Unbundle By Name(w1752) -> ("Main Screen.Start Test Temp"=w1756:refnum<vi>)
        n1120 = property class="Bool (strict)"(reference=w1756, "Value"=FALSE) -> (reference out=w1754:refnum<vi>, error out=w1755:errorcluster)  [unwired: 1 in]
        n1121 = Close Reference(reference=w1754, error in (no error)=w1755) -> ()  [unwired: 1 out]
      }
      frame "Error" {
        # "#CodeRecommended - If you ever change the name of this \"Error\" message, you'll need to update the name in the Check Loop Error.vi as well."
        # "#CodeRecommended - Consider creating a system for logging errors in some way. These errors are for notification purposes only. Handling of specific errors should be performed in the message frames that generated the error."
        # "Error - Display an error dialog. This message is sent by the \"Error Handler\" VIs at the end of other loops in this application."
        n1122 = Variant To Data(error in=w1766, type=errorcluster {"status"=FALSE, "code"=0, "source"=""} ("error constant"), Variant=w1764) -> (data=w1762:errorcluster, error out=w1761:errorcluster)
        n1123 = call <vilib>:"Simple Error Handler.vi"("error in (no error)"=w1762) -> ()  [unwired: 4 in, 5 out]
        n1124 = Merge Errors(w1761) -> (w1760:errorcluster)
      }
      frame "Confirm Quit" {
        # "#CodeNeeded - If you want to provide an \"Are you sure\" dialog (or some other notification) before the application exits, place that code here. This message is typically sent from a Panel Close? event."
        # "Confirm Quit - Message that can confirm whether or not the user wants to exit the application."
        n1125 = call-poly "Enqueue Message.vi"("Priority Message? (F)"=TRUE, "error in (no error)"=w1777, "Message"="Exit", "Message Queue"=w1774) -> ("error out"=w1775:errorcluster)  [unwired: 6 in, 1 out]
        n1126 = Merge Errors(w1775) -> (w1776:errorcluster)
        n1127 = call "LOAD CELL FGV MAIN.vi"("Enum"=T16."UNINITIAL", "error in (no error)"=w1776, "main ref"=w1767) -> ("error IO"=w1771:errorcluster)  [unwired: 8 in]
        n1128 = call "LOAD CELL FGV MAIN.vi"("Enum"=T16."DELETEHANDLE", "error in (no error)"=w1771, "main ref"=w1767) -> ("error IO"=w1769:errorcluster)  [unwired: 8 in]
      }
      frame "Exit" {
        # "Stop the VI"
        # "Release the message queue reference"
        # "#CodeNeeded - Add any required cleanup code here. Note that if 'Exit' was called as a result of an error, an error dialog will be displayed. Add any custom error handling for an 'Exit' condition here as well."
        # "Exit - Exit the application."
        n1129 = call "Fire User Event - Stop.vi"("User Event - Stop"=w1780) -> ("error out"=w1779:errorcluster)  [unwired: 10 in]
        n1130 = Release Queue(queue=w1785, error in (no error)=w1778) -> (error out=w1782:errorcluster)  [unwired: 1 in, 2 out]
        n1131 = Merge Errors(w1779, w1782) -> (w1781:errorcluster)
      }
      frame Default {
        # "'Default' case only runs if there is a message that isn't defined in any of the other cases.  Output a programming error."
        n1132 = xnode "Error Ring"("parameter 0"=w1786) -> ("error out"=w1787:errorcluster)
      }
    }
    n1133 = call "LAB-IQ Error Handler - Message Handling Loop.vi"("error in (no error)"=w847, "Message Queue"=w849) -> ("dup error in"=w848:errorcluster)  [unwired: 8 in, 1 out]
  }
  n1134 = while {
    shift-right: [w1806] -> _
    shift-left: w6 -> [w1807]
    tunnel: [w1800] -> w36
    tunnel: w35 -> [w1798]
    tunnel: w13 -> [w1797]
    tunnel: w25 -> [w1796]
    stop <- w1805 stop-if-true
    # "Load  Handling Loop"
    n1135 = call "Dequeue Message.vi"("error in (no error)"=w1797, "Message Queue"=w1798) -> ("error out"=w1804:errorcluster, "Message Data"=w1802:variant, "Message"=w1803:string, "dup Message Queue"=w1801:refnum<queue>)  [unwired: 6 in]
    n1136 = case "Message Cases" shown="\"Load Main\"" w1803 {
      selector: w1803 -> [_ _ _ _ _ w1852]
      tunnel: w1801 -> [w1808 w1820 _ w1839 w1851 _]
      tunnel: w1804 -> [w1811 w1818 w1836 w1843 w1845 _]
      tunnel: [w1812 w1821 w1830 w1841 w1847 w1853] -> w1799
      tunnel: w1807 -> [w1810 w1813 w1835 w1842 w1850 w1854]
      tunnel: [w1810 w1813 w1835 w1842 w1850 w1854] -> w1806
      tunnel: [_ _ _ _ TRUE _] -> w1805
      tunnel: w1802 -> [_ _ w1834 _ _ _]
      tunnel: w1796 -> [_ _ _ _ w1844 _]
      frame "init" {
        # "Bundle control references and a sample string value."
        # "Initialize - All initialization work should take place in this message, since other loops can potentially enqueue messages that execute immediately after this one."
        n1137 = call-poly "Enqueue Message.vi"("error in (no error)"=w1811, "Message"="Load Main", "Message Queue"=w1808) -> ("error out"=w1812:errorcluster)  [unwired: 7 in, 1 out]
      }
      frame "Load Main" {
        n1138 = call "LOAD CELL READ.vi"("error in (no error)"=w1818, "main ref"=w1813) -> ("error out"=w1814:errorcluster)  [unwired: 9 in]
        n1139 = Unbundle By Name(w1813) -> ("Main Home Screen.EXIT"=w1819:refnum<vi>)
        n1140 = property class="Bool (strict)"(reference=w1819) -> (reference out=w1816:refnum<vi>, error out=w1817:errorcluster, "Value"=w1815:bool)  [unwired: 1 in]
        n1141 = Close Reference(reference=w1816, error in (no error)=w1817) -> ()  [unwired: 1 out]
        n1142 = case shown="False" w1815 {
          tunnel: [w1824 w1828] -> w1821
          tunnel: w1820 -> [w1823 w1827]
          tunnel: w1814 -> [w1822 w1826]
          frame True {
            n1143 = call-poly "Enqueue Message.vi"("error in (no error)"=w1822, "Message"="Confirm Quit", "Message Queue"=w1823) -> ("error out"=w1824:errorcluster)  [unwired: 7 in, 1 out]
          }
          frame False {
            n1144 = call-poly "Enqueue Message.vi"("error in (no error)"=w1826, "Message"="Load Main", "Message Queue"=w1827) -> ("error out"=w1828:errorcluster)  [unwired: 7 in, 1 out]
          }
        }
      }
      frame "Error" {
        # "#CodeRecommended - If you ever change the name of this \"Error\" message, you'll need to update the name in the Check Loop Error.vi as well."
        # "#CodeRecommended - Consider creating a system for logging errors in some way. These errors are for notification purposes only. Handling of specific errors should be performed in the message frames that generated the error."
        # "Error - Display an error dialog. This message is sent by the \"Error Handler\" VIs at the end of other loops in this application."
        n1145 = Variant To Data(error in=w1836, type=errorcluster {"status"=FALSE, "code"=0, "source"=""} ("error constant"), Variant=w1834) -> (data=w1832:errorcluster, error out=w1831:errorcluster)
        n1146 = call <vilib>:"Simple Error Handler.vi"("error in (no error)"=w1832) -> ()  [unwired: 4 in, 5 out]
        n1147 = Merge Errors(w1831) -> (w1830:errorcluster)
      }
      frame "Confirm Quit" {
        # "#CodeNeeded - If you want to provide an \"Are you sure\" dialog (or some other notification) before the application exits, place that code here. This message is typically sent from a Panel Close? event."
        # "Confirm Quit - Message that can confirm whether or not the user wants to exit the application."
        n1148 = call-poly "Enqueue Message.vi"("Priority Message? (F)"=TRUE, "error in (no error)"=w1843, "Message"="Exit", "Message Queue"=w1839) -> ("error out"=w1840:errorcluster)  [unwired: 6 in, 1 out]
        n1149 = Merge Errors(w1840) -> (w1841:errorcluster)
      }
      frame "Exit" {
        # "Stop the VI"
        # "Release the message queue reference"
        # "#CodeNeeded - Add any required cleanup code here. Note that if 'Exit' was called as a result of an error, an error dialog will be displayed. Add any custom error handling for an 'Exit' condition here as well."
        # "Exit - Exit the application."
        n1150 = call "Fire User Event - Stop.vi"("User Event - Stop"=w1844) -> ("error out"=w1846:errorcluster)  [unwired: 10 in]
        n1151 = Release Queue(queue=w1851, error in (no error)=w1845) -> (error out=w1848:errorcluster)  [unwired: 1 in, 2 out]
        n1152 = Merge Errors(w1846, w1848) -> (w1847:errorcluster)
      }
      frame Default {
        # "'Default' case only runs if there is a message that isn't defined in any of the other cases.  Output a programming error."
        n1153 = xnode "Error Ring"("parameter 0"=w1852) -> ("error out"=w1853:errorcluster)
      }
    }
    n1154 = call "LAB-IQ Error Handler - Message Handling Loop.vi"("error in (no error)"=w1799, "Message Queue"=w1801) -> ("dup error in"=w1800:errorcluster)  [unwired: 8 in, 1 out]
  }
  n1155 = while {
    shift-right: [w1872] -> _
    shift-left: w6 -> [w1873]
    tunnel: [w1866] -> w33
    tunnel: w34 -> [w1864]
    tunnel: w13 -> [w1863]
    tunnel: w25 -> [w1862]
    stop <- w1871 stop-if-true
    # "Sway Motor  Handling Loop"
    n1156 = call "Dequeue Message.vi"("error in (no error)"=w1863, "Message Queue"=w1864) -> ("error out"=w1870:errorcluster, "Message Data"=w1868:variant, "Message"=w1869:string, "dup Message Queue"=w1867:refnum<queue>)  [unwired: 6 in]
    n1157 = case "Message Cases" shown="\"Exit\"" w1869 {
      selector: w1869 -> [_ _ _ _ _ w1917]
      tunnel: w1867 -> [w1874 w1885 _ w1904 w1916 _]
      tunnel: w1870 -> [w1877 w1882 w1901 w1908 w1910 _]
      tunnel: [w1878 w1886 w1895 w1906 w1912 w1918] -> w1865
      tunnel: w1873 -> [w1876 w1884 w1900 w1907 w1915 w1919]
      tunnel: [w1876 w1884 w1900 w1907 w1915 w1919] -> w1872
      tunnel: [_ _ _ _ TRUE _] -> w1871
      tunnel: w1868 -> [_ _ w1899 _ _ _]
      tunnel: w1862 -> [_ _ _ _ w1909 _]
      frame "init" {
        # "Bundle control references and a sample string value."
        # "Initialize - All initialization work should take place in this message, since other loops can potentially enqueue messages that execute immediately after this one."
        n1158 = call-poly "Enqueue Message.vi"("error in (no error)"=w1877, "Message"="Sway Main", "Message Queue"=w1874) -> ("error out"=w1878:errorcluster)  [unwired: 7 in, 1 out]
      }
      frame "Sway Main" {
        n1159 = Unbundle By Name(w1884) -> ("Main Home Screen.EXIT"=w1883:refnum<vi>)
        n1160 = property class="Bool (strict)"(reference=w1883) -> (reference out=w1880:refnum<vi>, error out=w1881:errorcluster, "Value"=w1879:bool)  [unwired: 1 in]
        n1161 = Close Reference(reference=w1880, error in (no error)=w1881) -> ()  [unwired: 1 out]
        n1162 = case shown="False" w1879 {
          tunnel: [w1889 w1893] -> w1886
          tunnel: w1885 -> [w1888 w1892]
          tunnel: w1882 -> [w1887 w1891]
          frame True {
            n1163 = call-poly "Enqueue Message.vi"("error in (no error)"=w1887, "Message"="Confirm Quit", "Message Queue"=w1888) -> ("error out"=w1889:errorcluster)  [unwired: 7 in, 1 out]
          }
          frame False {
            n1164 = call-poly "Enqueue Message.vi"("error in (no error)"=w1891, "Message"="Sway Main", "Message Queue"=w1892) -> ("error out"=w1893:errorcluster)  [unwired: 7 in, 1 out]
          }
        }
      }
      frame "Error" {
        # "#CodeRecommended - If you ever change the name of this \"Error\" message, you'll need to update the name in the Check Loop Error.vi as well."
        # "#CodeRecommended - Consider creating a system for logging errors in some way. These errors are for notification purposes only. Handling of specific errors should be performed in the message frames that generated the error."
        # "Error - Display an error dialog. This message is sent by the \"Error Handler\" VIs at the end of other loops in this application."
        n1165 = Variant To Data(error in=w1901, type=errorcluster {"status"=FALSE, "code"=0, "source"=""} ("error constant"), Variant=w1899) -> (data=w1897:errorcluster, error out=w1896:errorcluster)
        n1166 = call <vilib>:"Simple Error Handler.vi"("error in (no error)"=w1897) -> ()  [unwired: 4 in, 5 out]
        n1167 = Merge Errors(w1896) -> (w1895:errorcluster)
      }
      frame "Confirm Quit" {
        # "#CodeNeeded - If you want to provide an \"Are you sure\" dialog (or some other notification) before the application exits, place that code here. This message is typically sent from a Panel Close? event."
        # "Confirm Quit - Message that can confirm whether or not the user wants to exit the application."
        n1168 = call-poly "Enqueue Message.vi"("Priority Message? (F)"=TRUE, "error in (no error)"=w1908, "Message"="Exit", "Message Queue"=w1904) -> ("error out"=w1905:errorcluster)  [unwired: 6 in, 1 out]
        n1169 = Merge Errors(w1905) -> (w1906:errorcluster)
      }
      frame "Exit" {
        # "Stop the VI"
        # "Release the message queue reference"
        # "#CodeNeeded - Add any required cleanup code here. Note that if 'Exit' was called as a result of an error, an error dialog will be displayed. Add any custom error handling for an 'Exit' condition here as well."
        # "Exit - Exit the application."
        n1170 = call "Fire User Event - Stop.vi"("User Event - Stop"=w1909) -> ("error out"=w1911:errorcluster)  [unwired: 10 in]
        n1171 = Release Queue(queue=w1916, error in (no error)=w1910) -> (error out=w1913:errorcluster)  [unwired: 1 in, 2 out]
        n1172 = Merge Errors(w1911, w1913) -> (w1912:errorcluster)
      }
      frame Default {
        # "'Default' case only runs if there is a message that isn't defined in any of the other cases.  Output a programming error."
        n1173 = xnode "Error Ring"("parameter 0"=w1917) -> ("error out"=w1918:errorcluster)
      }
    }
    n1174 = call "LAB-IQ Error Handler - Message Handling Loop.vi"("error in (no error)"=w1865, "Message Queue"=w1867) -> ("dup error in"=w1866:errorcluster)  [unwired: 8 in, 1 out]
  }
  n1175 = while {
    shift-right: [w1937] -> _
    shift-left: w6 -> [w1938]
    tunnel: [w1931] -> w30
    tunnel: w32 -> [w1929]
    tunnel: w13 -> [w1928]
    tunnel: w25 -> [w1927]
    stop <- w1936 stop-if-true
    # "Temperature  Handling Loop"
    n1176 = call "Dequeue Message.vi"("error in (no error)"=w1928, "Message Queue"=w1929) -> ("error out"=w1935:errorcluster, "Message Data"=w1933:variant, "Message"=w1934:string, "dup Message Queue"=w1932:refnum<queue>)  [unwired: 6 in]
    n1177 = case "Message Cases" shown="\"Temperature Main\"" w1934 {
      selector: w1934 -> [_ _ _ _ _ w1982]
      tunnel: w1932 -> [w1939 w1950 _ w1969 w1981 _]
      tunnel: w1935 -> [w1942 w1947 w1966 w1973 w1975 _]
      tunnel: [w1943 w1951 w1960 w1971 w1977 w1983] -> w1930
      tunnel: w1938 -> [w1941 w1949 w1965 w1972 w1980 w1984]
      tunnel: [w1941 w1949 w1965 w1972 w1980 w1984] -> w1937
      tunnel: [_ _ _ _ TRUE _] -> w1936
      tunnel: w1933 -> [_ _ w1964 _ _ _]
      tunnel: w1927 -> [_ _ _ _ w1974 _]
      frame "init" {
        # "Initialize - All initialization work should take place in this message, since other loops can potentially enqueue messages that execute immediately after this one."
        n1178 = call-poly "Enqueue Message.vi"("error in (no error)"=w1942, "Message"="Temperature Main", "Message Queue"=w1939) -> ("error out"=w1943:errorcluster)  [unwired: 7 in, 1 out]
      }
      frame "Temperature Main" {
        n1179 = Unbundle By Name(w1949) -> ("Main Home Screen.EXIT"=w1948:refnum<vi>)
        n1180 = property class="Bool (strict)"(reference=w1948) -> (reference out=w1945:refnum<vi>, error out=w1946:errorcluster, "Value"=w1944:bool)  [unwired: 1 in]
        n1181 = case shown="False" w1944 {
          tunnel: [w1954 w1958] -> w1951
          tunnel: w1950 -> [w1953 w1957]
          tunnel: w1947 -> [w1952 w1956]
          frame True {
            n1182 = call-poly "Enqueue Message.vi"("error in (no error)"=w1952, "Message"="Confirm Quit", "Message Queue"=w1953) -> ("error out"=w1954:errorcluster)  [unwired: 7 in, 1 out]
          }
          frame False {
            n1183 = call-poly "Enqueue Message.vi"("error in (no error)"=w1956, "Message"="Temperature Main", "Message Queue"=w1957) -> ("error out"=w1958:errorcluster)  [unwired: 7 in, 1 out]
          }
        }
        n1184 = Close Reference(reference=w1945, error in (no error)=w1946) -> ()  [unwired: 1 out]
      }
      frame "Error" {
        # "#CodeRecommended - If you ever change the name of this \"Error\" message, you'll need to update the name in the Check Loop Error.vi as well."
        # "#CodeRecommended - Consider creating a system for logging errors in some way. These errors are for notification purposes only. Handling of specific errors should be performed in the message frames that generated the error."
        # "Error - Display an error dialog. This message is sent by the \"Error Handler\" VIs at the end of other loops in this application."
        n1185 = Variant To Data(error in=w1966, type=errorcluster {"status"=FALSE, "code"=0, "source"=""} ("error constant"), Variant=w1964) -> (data=w1962:errorcluster, error out=w1961:errorcluster)
        n1186 = call <vilib>:"Simple Error Handler.vi"("error in (no error)"=w1962) -> ()  [unwired: 4 in, 5 out]
        n1187 = Merge Errors(w1961) -> (w1960:errorcluster)
      }
      frame "Confirm Quit" {
        # "#CodeNeeded - If you want to provide an \"Are you sure\" dialog (or some other notification) before the application exits, place that code here. This message is typically sent from a Panel Close? event."
        # "Confirm Quit - Message that can confirm whether or not the user wants to exit the application."
        n1188 = call-poly "Enqueue Message.vi"("Priority Message? (F)"=TRUE, "error in (no error)"=w1973, "Message"="Exit", "Message Queue"=w1969) -> ("error out"=w1970:errorcluster)  [unwired: 6 in, 1 out]
        n1189 = Merge Errors(w1970) -> (w1971:errorcluster)
      }
      frame "Exit" {
        # "Stop the VI"
        # "Release the message queue reference"
        # "#CodeNeeded - Add any required cleanup code here. Note that if 'Exit' was called as a result of an error, an error dialog will be displayed. Add any custom error handling for an 'Exit' condition here as well."
        # "Exit - Exit the application."
        n1190 = call "Fire User Event - Stop.vi"("User Event - Stop"=w1974) -> ("error out"=w1976:errorcluster)  [unwired: 10 in]
        n1191 = Release Queue(queue=w1981, error in (no error)=w1975) -> (error out=w1978:errorcluster)  [unwired: 1 in, 2 out]
        n1192 = Merge Errors(w1976, w1978) -> (w1977:errorcluster)
      }
      frame Default {
        # "'Default' case only runs if there is a message that isn't defined in any of the other cases.  Output a programming error."
        n1193 = xnode "Error Ring"("parameter 0"=w1982) -> ("error out"=w1983:errorcluster)
      }
    }
    n1194 = call "LAB-IQ Error Handler - Message Handling Loop.vi"("error in (no error)"=w1930, "Message Queue"=w1932) -> ("dup error in"=w1931:errorcluster)  [unwired: 8 in, 1 out]
  }
  n1195 = while {
    shift-right: [w2002] -> _
    shift-left: w6 -> [w2003]
    tunnel: [w1996] -> _
    tunnel: w29 -> [w1994]
    tunnel: w13 -> [w1993]
    tunnel: w25 -> [w1992]
    stop <- w2001 stop-if-true
    # "Ramp Motor  Handling Loop"
    n1196 = call "Dequeue Message.vi"("error in (no error)"=w1993, "Message Queue"=w1994) -> ("error out"=w2000:errorcluster, "Message Data"=w1998:variant, "Message"=w1999:string, "dup Message Queue"=w1997:refnum<queue>)  [unwired: 6 in]
    n1197 = case "Message Cases" shown="\"Ramp Main\"" w1999 {
      selector: w1999 -> [_ _ _ _ _ w2047]
      tunnel: w1997 -> [w2004 w2015 _ w2034 w2046 _]
      tunnel: w2000 -> [w2007 w2012 w2031 w2038 w2040 _]
      tunnel: [w2008 w2016 w2025 w2036 w2042 w2048] -> w1995
      tunnel: w2003 -> [w2006 w2014 w2030 w2037 w2045 w2049]
      tunnel: [w2006 w2014 w2030 w2037 w2045 w2049] -> w2002
      tunnel: [_ _ _ _ TRUE _] -> w2001
      tunnel: w1998 -> [_ _ w2029 _ _ _]
      tunnel: w1992 -> [_ _ _ _ w2039 _]
      frame "init" {
        # "Initialize - All initialization work should take place in this message, since other loops can potentially enqueue messages that execute immediately after this one."
        n1198 = call-poly "Enqueue Message.vi"("error in (no error)"=w2007, "Message"="Ramp Main", "Message Queue"=w2004) -> ("error out"=w2008:errorcluster)  [unwired: 7 in, 1 out]
      }
      frame "Ramp Main" {
        n1199 = Unbundle By Name(w2014) -> ("Main Home Screen.EXIT"=w2013:refnum<vi>)
        n1200 = property class="Bool (strict)"(reference=w2013) -> (reference out=w2010:refnum<vi>, error out=w2011:errorcluster, "Value"=w2009:bool)  [unwired: 1 in]
        n1201 = case shown="False" w2009 {
          tunnel: [w2019 w2023] -> w2016
          tunnel: w2015 -> [w2018 w2022]
          tunnel: w2012 -> [w2017 w2021]
          frame True {
            n1202 = call-poly "Enqueue Message.vi"("error in (no error)"=w2017, "Message"="Confirm Quit", "Message Queue"=w2018) -> ("error out"=w2019:errorcluster)  [unwired: 7 in, 1 out]
          }
          frame False {
            n1203 = call-poly "Enqueue Message.vi"("error in (no error)"=w2021, "Message"="Ramp Main", "Message Queue"=w2022) -> ("error out"=w2023:errorcluster)  [unwired: 7 in, 1 out]
          }
        }
        n1204 = Close Reference(reference=w2010, error in (no error)=w2011) -> ()  [unwired: 1 out]
      }
      frame "Error" {
        # "#CodeRecommended - If you ever change the name of this \"Error\" message, you'll need to update the name in the Check Loop Error.vi as well."
        # "#CodeRecommended - Consider creating a system for logging errors in some way. These errors are for notification purposes only. Handling of specific errors should be performed in the message frames that generated the error."
        # "Error - Display an error dialog. This message is sent by the \"Error Handler\" VIs at the end of other loops in this application."
        n1205 = Variant To Data(error in=w2031, type=errorcluster {"status"=FALSE, "code"=0, "source"=""} ("error constant"), Variant=w2029) -> (data=w2027:errorcluster, error out=w2026:errorcluster)
        n1206 = call <vilib>:"Simple Error Handler.vi"("error in (no error)"=w2027) -> ()  [unwired: 4 in, 5 out]
        n1207 = Merge Errors(w2026) -> (w2025:errorcluster)
      }
      frame "Confirm Quit" {
        # "#CodeNeeded - If you want to provide an \"Are you sure\" dialog (or some other notification) before the application exits, place that code here. This message is typically sent from a Panel Close? event."
        # "Confirm Quit - Message that can confirm whether or not the user wants to exit the application."
        n1208 = call-poly "Enqueue Message.vi"("Priority Message? (F)"=TRUE, "error in (no error)"=w2038, "Message"="Exit", "Message Queue"=w2034) -> ("error out"=w2035:errorcluster)  [unwired: 6 in, 1 out]
        n1209 = Merge Errors(w2035) -> (w2036:errorcluster)
      }
      frame "Exit" {
        # "Stop the VI"
        # "Release the message queue reference"
        # "#CodeNeeded - Add any required cleanup code here. Note that if 'Exit' was called as a result of an error, an error dialog will be displayed. Add any custom error handling for an 'Exit' condition here as well."
        # "Exit - Exit the application."
        n1210 = call "Fire User Event - Stop.vi"("User Event - Stop"=w2039) -> ("error out"=w2041:errorcluster)  [unwired: 10 in]
        n1211 = Release Queue(queue=w2046, error in (no error)=w2040) -> (error out=w2043:errorcluster)  [unwired: 1 in, 2 out]
        n1212 = Merge Errors(w2041, w2043) -> (w2042:errorcluster)
      }
      frame Default {
        # "'Default' case only runs if there is a message that isn't defined in any of the other cases.  Output a programming error."
        n1213 = xnode "Error Ring"("parameter 0"=w2047) -> ("error out"=w2048:errorcluster)
      }
    }
    n1214 = call "LAB-IQ Error Handler - Message Handling Loop.vi"("error in (no error)"=w1995, "Message Queue"=w1997) -> ("dup error in"=w1996:errorcluster)  [unwired: 8 in, 1 out]
  }
  n1215 = while {
    shift-right: [w2067] -> _
    shift-left: w6 -> [w2068]
    tunnel: [w2061] -> _
    tunnel: w28 -> [w2059]
    tunnel: w13 -> [w2058]
    tunnel: w25 -> [w2057]
    stop <- w2066 stop-if-true
    # "ECR  Handling Loop"
    n1216 = call "Dequeue Message.vi"("error in (no error)"=w2058, "Message Queue"=w2059) -> ("error out"=w2065:errorcluster, "Message Data"=w2063:variant, "Message"=w2064:string, "dup Message Queue"=w2062:refnum<queue>)  [unwired: 6 in]
    n1217 = case "Message Cases" shown="\"ECR Main\"" w2064 {
      selector: w2064 -> [_ _ _ _ _ w2112]
      tunnel: w2062 -> [w2069 w2080 _ w2099 w2111 _]
      tunnel: w2065 -> [w2072 w2077 w2096 w2103 w2105 _]
      tunnel: [w2073 w2081 w2090 w2101 w2107 w2113] -> w2060
      tunnel: w2068 -> [w2071 w2079 w2095 w2102 w2110 w2114]
      tunnel: [w2071 w2079 w2095 w2102 w2110 w2114] -> w2067
      tunnel: [_ _ _ _ TRUE _] -> w2066
      tunnel: w2063 -> [_ _ w2094 _ _ _]
      tunnel: w2057 -> [_ _ _ _ w2104 _]
      frame "init" {
        # "Initialize - All initialization work should take place in this message, since other loops can potentially enqueue messages that execute immediately after this one."
        n1218 = call-poly "Enqueue Message.vi"("error in (no error)"=w2072, "Message"="ECR Main", "Message Queue"=w2069) -> ("error out"=w2073:errorcluster)  [unwired: 7 in, 1 out]
      }
      frame "ECR Main" {
        n1219 = Unbundle By Name(w2079) -> ("Main Home Screen.EXIT"=w2078:refnum<vi>)
        n1220 = property class="Bool (strict)"(reference=w2078) -> (reference out=w2075:refnum<vi>, error out=w2076:errorcluster, "Value"=w2074:bool)  [unwired: 1 in]
        n1221 = case shown="False" w2074 {
          tunnel: [w2084 w2088] -> w2081
          tunnel: w2080 -> [w2083 w2087]
          tunnel: w2077 -> [w2082 w2086]
          frame True {
            n1222 = call-poly "Enqueue Message.vi"("error in (no error)"=w2082, "Message"="Confirm Quit", "Message Queue"=w2083) -> ("error out"=w2084:errorcluster)  [unwired: 7 in, 1 out]
          }
          frame False {
            n1223 = call-poly "Enqueue Message.vi"("error in (no error)"=w2086, "Message"="ECR Main", "Message Queue"=w2087) -> ("error out"=w2088:errorcluster)  [unwired: 7 in, 1 out]
          }
        }
        n1224 = Close Reference(reference=w2075, error in (no error)=w2076) -> ()  [unwired: 1 out]
      }
      frame "Error" {
        # "#CodeRecommended - If you ever change the name of this \"Error\" message, you'll need to update the name in the Check Loop Error.vi as well."
        # "#CodeRecommended - Consider creating a system for logging errors in some way. These errors are for notification purposes only. Handling of specific errors should be performed in the message frames that generated the error."
        # "Error - Display an error dialog. This message is sent by the \"Error Handler\" VIs at the end of other loops in this application."
        n1225 = Variant To Data(error in=w2096, type=errorcluster {"status"=FALSE, "code"=0, "source"=""} ("error constant"), Variant=w2094) -> (data=w2092:errorcluster, error out=w2091:errorcluster)
        n1226 = call <vilib>:"Simple Error Handler.vi"("error in (no error)"=w2092) -> ()  [unwired: 4 in, 5 out]
        n1227 = Merge Errors(w2091) -> (w2090:errorcluster)
      }
      frame "Confirm Quit" {
        # "#CodeNeeded - If you want to provide an \"Are you sure\" dialog (or some other notification) before the application exits, place that code here. This message is typically sent from a Panel Close? event."
        # "Confirm Quit - Message that can confirm whether or not the user wants to exit the application."
        n1228 = call-poly "Enqueue Message.vi"("Priority Message? (F)"=TRUE, "error in (no error)"=w2103, "Message"="Exit", "Message Queue"=w2099) -> ("error out"=w2100:errorcluster)  [unwired: 6 in, 1 out]
        n1229 = Merge Errors(w2100) -> (w2101:errorcluster)
      }
      frame "Exit" {
        # "Stop the VI"
        # "Release the message queue reference"
        # "#CodeNeeded - Add any required cleanup code here. Note that if 'Exit' was called as a result of an error, an error dialog will be displayed. Add any custom error handling for an 'Exit' condition here as well."
        # "Exit - Exit the application."
        n1230 = call "Fire User Event - Stop.vi"("User Event - Stop"=w2104) -> ("error out"=w2106:errorcluster)  [unwired: 10 in]
        n1231 = Release Queue(queue=w2111, error in (no error)=w2105) -> (error out=w2108:errorcluster)  [unwired: 1 in, 2 out]
        n1232 = Merge Errors(w2106, w2108) -> (w2107:errorcluster)
      }
      frame Default {
        # "'Default' case only runs if there is a message that isn't defined in any of the other cases.  Output a programming error."
        n1233 = xnode "Error Ring"("parameter 0"=w2112) -> ("error out"=w2113:errorcluster)
      }
    }
    n1234 = call "LAB-IQ Error Handler - Message Handling Loop.vi"("error in (no error)"=w2060, "Message Queue"=w2062) -> ("dup error in"=w2061:errorcluster)  [unwired: 8 in, 1 out]
  }
  n1235 = while {
    shift-right: [w2132] -> _
    shift-left: w6 -> [w2133]
    tunnel: [w2126] -> _
    tunnel: w27 -> [w2124]
    tunnel: w13 -> [w2123]
    tunnel: w25 -> [w2122]
    stop <- w2131 stop-if-true
    # "Humidity  Handling Loop"
    n1236 = call "Dequeue Message.vi"("error in (no error)"=w2123, "Message Queue"=w2124) -> ("error out"=w2130:errorcluster, "Message Data"=w2128:variant, "Message"=w2129:string, "dup Message Queue"=w2127:refnum<queue>)  [unwired: 6 in]
    n1237 = case "Message Cases" shown="\"Humidity Main\"" w2129 {
      selector: w2129 -> [_ _ _ _ _ w2177]
      tunnel: w2127 -> [w2134 w2145 _ w2164 w2176 _]
      tunnel: w2130 -> [w2137 w2142 w2161 w2168 w2170 _]
      tunnel: [w2138 w2146 w2155 w2166 w2172 w2178] -> w2125
      tunnel: w2133 -> [w2136 w2144 w2160 w2167 w2175 w2179]
      tunnel: [w2136 w2144 w2160 w2167 w2175 w2179] -> w2132
      tunnel: [_ _ _ _ TRUE _] -> w2131
      tunnel: w2128 -> [_ _ w2159 _ _ _]
      tunnel: w2122 -> [_ _ _ _ w2169 _]
      frame "init" {
        # "Initialize - All initialization work should take place in this message, since other loops can potentially enqueue messages that execute immediately after this one."
        n1238 = call-poly "Enqueue Message.vi"("error in (no error)"=w2137, "Message"="Humidity Main", "Message Queue"=w2134) -> ("error out"=w2138:errorcluster)  [unwired: 7 in, 1 out]
      }
      frame "Humidity Main" {
        n1239 = Unbundle By Name(w2144) -> ("Main Home Screen.EXIT"=w2143:refnum<vi>)
        n1240 = property class="Bool (strict)"(reference=w2143) -> (reference out=w2140:refnum<vi>, error out=w2141:errorcluster, "Value"=w2139:bool)  [unwired: 1 in]
        n1241 = case shown="False" w2139 {
          tunnel: [w2149 w2153] -> w2146
          tunnel: w2145 -> [w2148 w2152]
          tunnel: w2142 -> [w2147 w2151]
          frame True {
            n1242 = call-poly "Enqueue Message.vi"("error in (no error)"=w2147, "Message"="Confirm Quit", "Message Queue"=w2148) -> ("error out"=w2149:errorcluster)  [unwired: 7 in, 1 out]
          }
          frame False {
            n1243 = call-poly "Enqueue Message.vi"("error in (no error)"=w2151, "Message"="Humidity Main", "Message Queue"=w2152) -> ("error out"=w2153:errorcluster)  [unwired: 7 in, 1 out]
          }
        }
        n1244 = Close Reference(reference=w2140, error in (no error)=w2141) -> ()  [unwired: 1 out]
      }
      frame "Error" {
        # "#CodeRecommended - If you ever change the name of this \"Error\" message, you'll need to update the name in the Check Loop Error.vi as well."
        # "#CodeRecommended - Consider creating a system for logging errors in some way. These errors are for notification purposes only. Handling of specific errors should be performed in the message frames that generated the error."
        # "Error - Display an error dialog. This message is sent by the \"Error Handler\" VIs at the end of other loops in this application."
        n1245 = Variant To Data(error in=w2161, type=errorcluster {"status"=FALSE, "code"=0, "source"=""} ("error constant"), Variant=w2159) -> (data=w2157:errorcluster, error out=w2156:errorcluster)
        n1246 = call <vilib>:"Simple Error Handler.vi"("error in (no error)"=w2157) -> ()  [unwired: 4 in, 5 out]
        n1247 = Merge Errors(w2156) -> (w2155:errorcluster)
      }
      frame "Confirm Quit" {
        # "#CodeNeeded - If you want to provide an \"Are you sure\" dialog (or some other notification) before the application exits, place that code here. This message is typically sent from a Panel Close? event."
        # "Confirm Quit - Message that can confirm whether or not the user wants to exit the application."
        n1248 = call-poly "Enqueue Message.vi"("Priority Message? (F)"=TRUE, "error in (no error)"=w2168, "Message"="Exit", "Message Queue"=w2164) -> ("error out"=w2165:errorcluster)  [unwired: 6 in, 1 out]
        n1249 = Merge Errors(w2165) -> (w2166:errorcluster)
      }
      frame "Exit" {
        # "Stop the VI"
        # "Release the message queue reference"
        # "#CodeNeeded - Add any required cleanup code here. Note that if 'Exit' was called as a result of an error, an error dialog will be displayed. Add any custom error handling for an 'Exit' condition here as well."
        # "Exit - Exit the application."
        n1250 = call "Fire User Event - Stop.vi"("User Event - Stop"=w2169) -> ("error out"=w2171:errorcluster)  [unwired: 10 in]
        n1251 = Release Queue(queue=w2176, error in (no error)=w2170) -> (error out=w2173:errorcluster)  [unwired: 1 in, 2 out]
        n1252 = Merge Errors(w2171, w2173) -> (w2172:errorcluster)
      }
      frame Default {
        # "'Default' case only runs if there is a message that isn't defined in any of the other cases.  Output a programming error."
        n1253 = xnode "Error Ring"("parameter 0"=w2177) -> ("error out"=w2178:errorcluster)
      }
    }
    n1254 = call "LAB-IQ Error Handler - Message Handling Loop.vi"("error in (no error)"=w2125, "Message Queue"=w2127) -> ("dup error in"=w2126:errorcluster)  [unwired: 8 in, 1 out]
  }
  n1255 = while {
    shift-right: [w2197] -> _
    shift-left: w6 -> [w2198]
    tunnel: [w2191] -> _
    tunnel: w26 -> [w2189]
    tunnel: w13 -> [w2188]
    tunnel: w25 -> [w2187]
    stop <- w2196 stop-if-true
    # "Program  Handling Loop"
    n1256 = call "Dequeue Message.vi"("error in (no error)"=w2188, "Message Queue"=w2189) -> ("error out"=w2195:errorcluster, "Message Data"=w2193:variant, "Message"=w2194:string, "dup Message Queue"=w2192:refnum<queue>)  [unwired: 6 in]
    n1257 = case "Message Cases" shown="Default" w2194 {
      selector: w2194 -> [_ _ _ _ _ w2242]
      tunnel: w2192 -> [w2199 w2210 _ w2229 w2241 _]
      tunnel: w2195 -> [w2202 w2207 w2226 w2233 w2235 _]
      tunnel: [w2203 w2211 w2220 w2231 w2237 w2243] -> w2190
      tunnel: w2198 -> [w2201 w2209 w2225 w2232 w2240 w2244]
      tunnel: [w2201 w2209 w2225 w2232 w2240 w2244] -> w2197
      tunnel: [_ _ _ _ TRUE _] -> w2196
      tunnel: w2193 -> [_ _ w2224 _ _ _]
      tunnel: w2187 -> [_ _ _ _ w2234 _]
      frame "init" {
        # "Initialize - All initialization work should take place in this message, since other loops can potentially enqueue messages that execute immediately after this one."
        n1258 = call-poly "Enqueue Message.vi"("error in (no error)"=w2202, "Message"="Program Main", "Message Queue"=w2199) -> ("error out"=w2203:errorcluster)  [unwired: 7 in, 1 out]
      }
      frame "Program Main" {
        n1259 = Unbundle By Name(w2209) -> ("Main Home Screen.EXIT"=w2208:refnum<vi>)
        n1260 = property class="Bool (strict)"(reference=w2208) -> (reference out=w2205:refnum<vi>, error out=w2206:errorcluster, "Value"=w2204:bool)  [unwired: 1 in]
        n1261 = case shown="False" w2204 {
          tunnel: [w2214 w2218] -> w2211
          tunnel: w2210 -> [w2213 w2217]
          tunnel: w2207 -> [w2212 w2216]
          frame True {
            n1262 = call-poly "Enqueue Message.vi"("error in (no error)"=w2212, "Message"="Confirm Quit", "Message Queue"=w2213) -> ("error out"=w2214:errorcluster)  [unwired: 7 in, 1 out]
          }
          frame False {
            n1263 = call-poly "Enqueue Message.vi"("error in (no error)"=w2216, "Message"="Program Main", "Message Queue"=w2217) -> ("error out"=w2218:errorcluster)  [unwired: 7 in, 1 out]
          }
        }
        n1264 = Close Reference(reference=w2205, error in (no error)=w2206) -> ()  [unwired: 1 out]
      }
      frame "Error" {
        # "#CodeRecommended - If you ever change the name of this \"Error\" message, you'll need to update the name in the Check Loop Error.vi as well."
        # "#CodeRecommended - Consider creating a system for logging errors in some way. These errors are for notification purposes only. Handling of specific errors should be performed in the message frames that generated the error."
        # "Error - Display an error dialog. This message is sent by the \"Error Handler\" VIs at the end of other loops in this application."
        n1265 = Variant To Data(error in=w2226, type=errorcluster {"status"=FALSE, "code"=0, "source"=""} ("error constant"), Variant=w2224) -> (data=w2222:errorcluster, error out=w2221:errorcluster)
        n1266 = call <vilib>:"Simple Error Handler.vi"("error in (no error)"=w2222) -> ()  [unwired: 4 in, 5 out]
        n1267 = Merge Errors(w2221) -> (w2220:errorcluster)
      }
      frame "Confirm Quit" {
        # "#CodeNeeded - If you want to provide an \"Are you sure\" dialog (or some other notification) before the application exits, place that code here. This message is typically sent from a Panel Close? event."
        # "Confirm Quit - Message that can confirm whether or not the user wants to exit the application."
        n1268 = call-poly "Enqueue Message.vi"("Priority Message? (F)"=TRUE, "error in (no error)"=w2233, "Message"="Exit", "Message Queue"=w2229) -> ("error out"=w2230:errorcluster)  [unwired: 6 in, 1 out]
        n1269 = Merge Errors(w2230) -> (w2231:errorcluster)
      }
      frame "Exit" {
        # "Stop the VI"
        # "Release the message queue reference"
        # "#CodeNeeded - Add any required cleanup code here. Note that if 'Exit' was called as a result of an error, an error dialog will be displayed. Add any custom error handling for an 'Exit' condition here as well."
        # "Exit - Exit the application."
        n1270 = call "Fire User Event - Stop.vi"("User Event - Stop"=w2234) -> ("error out"=w2236:errorcluster)  [unwired: 10 in]
        n1271 = Release Queue(queue=w2241, error in (no error)=w2235) -> (error out=w2238:errorcluster)  [unwired: 1 in, 2 out]
        n1272 = Merge Errors(w2236, w2238) -> (w2237:errorcluster)
      }
      frame Default {
        # "'Default' case only runs if there is a message that isn't defined in any of the other cases.  Output a programming error."
        n1273 = xnode "Error Ring"("parameter 0"=w2242) -> ("error out"=w2243:errorcluster)
      }
    }
    n1274 = call "LAB-IQ Error Handler - Message Handling Loop.vi"("error in (no error)"=w2190, "Message Queue"=w2192) -> ("dup error in"=w2191:errorcluster)  [unwired: 8 in, 1 out]
  }
  n1275 = while {
    shift-right: [w2262] -> _
    shift-left: w6 -> [w2263]
    tunnel: [w2256] -> _
    tunnel: w24 -> [w2254]
    tunnel: w13 -> [w2253]
    tunnel: w25 -> [w2252]
    stop <- w2261 stop-if-true
    # "Monitor  Handling Loop"
    n1276 = call "Dequeue Message.vi"("error in (no error)"=w2253, "Message Queue"=w2254) -> ("error out"=w2260:errorcluster, "Message Data"=w2258:variant, "Message"=w2259:string, "dup Message Queue"=w2257:refnum<queue>)  [unwired: 6 in]
    n1277 = case "Message Cases" shown="\"Monitor Main\"" w2259 {
      selector: w2259 -> [_ _ _ _ _ w2308]
      tunnel: w2257 -> [w2264 w2276 _ w2295 w2307 _]
      tunnel: w2260 -> [w2267 w2274 w2292 w2299 w2301 _]
      tunnel: [w2268 w2277 w2286 w2297 w2303 w2309] -> w2255
      tunnel: w2263 -> [w2266 w2269 w2291 w2298 w2306 w2310]
      tunnel: [w2266 w2269 w2291 w2298 w2306 w2310] -> w2262
      tunnel: [_ _ _ _ TRUE _] -> w2261
      tunnel: w2258 -> [_ _ w2290 _ _ _]
      tunnel: w2252 -> [_ _ _ _ w2300 _]
      frame "init" {
        # "Initialize - All initialization work should take place in this message, since other loops can potentially enqueue messages that execute immediately after this one."
        n1278 = call-poly "Enqueue Message.vi"("error in (no error)"=w2267, "Message"="Monitor Main", "Message Queue"=w2264) -> ("error out"=w2268:errorcluster)  [unwired: 7 in, 1 out]
      }
      frame "Monitor Main" {
        n1279 = call "Main Monitor Loop.vi"("error in (no error)"=w2274, "main ref"=w2269) -> ("error out"=w2270:errorcluster)  [unwired: 9 in]
        n1280 = Unbundle By Name(w2269) -> ("Main Home Screen.EXIT"=w2275:refnum<vi>)
        n1281 = property class="Bool (strict)"(reference=w2275) -> (reference out=w2272:refnum<vi>, error out=w2273:errorcluster, "Value"=w2271:bool)  [unwired: 1 in]
        n1282 = case shown="False" w2271 {
          tunnel: [w2280 w2284] -> w2277
          tunnel: w2276 -> [w2279 w2283]
          tunnel: w2270 -> [w2278 w2282]
          frame True {
            n1283 = call-poly "Enqueue Message.vi"("error in (no error)"=w2278, "Message"="Confirm Quit", "Message Queue"=w2279) -> ("error out"=w2280:errorcluster)  [unwired: 7 in, 1 out]
          }
          frame False {
            n1284 = call-poly "Enqueue Message.vi"("error in (no error)"=w2282, "Message"="Monitor Main", "Message Queue"=w2283) -> ("error out"=w2284:errorcluster)  [unwired: 7 in, 1 out]
          }
        }
        n1285 = Close Reference(reference=w2272, error in (no error)=w2273) -> ()  [unwired: 1 out]
      }
      frame "Error" {
        # "#CodeRecommended - If you ever change the name of this \"Error\" message, you'll need to update the name in the Check Loop Error.vi as well."
        # "#CodeRecommended - Consider creating a system for logging errors in some way. These errors are for notification purposes only. Handling of specific errors should be performed in the message frames that generated the error."
        # "Error - Display an error dialog. This message is sent by the \"Error Handler\" VIs at the end of other loops in this application."
        n1286 = Variant To Data(error in=w2292, type=errorcluster {"status"=FALSE, "code"=0, "source"=""} ("error constant"), Variant=w2290) -> (data=w2288:errorcluster, error out=w2287:errorcluster)
        n1287 = call <vilib>:"Simple Error Handler.vi"("error in (no error)"=w2288) -> ()  [unwired: 4 in, 5 out]
        n1288 = Merge Errors(w2287) -> (w2286:errorcluster)
      }
      frame "Confirm Quit" {
        # "#CodeNeeded - If you want to provide an \"Are you sure\" dialog (or some other notification) before the application exits, place that code here. This message is typically sent from a Panel Close? event."
        # "Confirm Quit - Message that can confirm whether or not the user wants to exit the application."
        n1289 = call-poly "Enqueue Message.vi"("Priority Message? (F)"=TRUE, "error in (no error)"=w2299, "Message"="Exit", "Message Queue"=w2295) -> ("error out"=w2296:errorcluster)  [unwired: 6 in, 1 out]
        n1290 = Merge Errors(w2296) -> (w2297:errorcluster)
      }
      frame "Exit" {
        # "Stop the VI"
        # "Release the message queue reference"
        # "#CodeNeeded - Add any required cleanup code here. Note that if 'Exit' was called as a result of an error, an error dialog will be displayed. Add any custom error handling for an 'Exit' condition here as well."
        # "Exit - Exit the application."
        n1291 = call "Fire User Event - Stop.vi"("User Event - Stop"=w2300) -> ("error out"=w2302:errorcluster)  [unwired: 10 in]
        n1292 = Release Queue(queue=w2307, error in (no error)=w2301) -> (error out=w2304:errorcluster)  [unwired: 1 in, 2 out]
        n1293 = Merge Errors(w2302, w2304) -> (w2303:errorcluster)
      }
      frame Default {
        # "'Default' case only runs if there is a message that isn't defined in any of the other cases.  Output a programming error."
        n1294 = xnode "Error Ring"("parameter 0"=w2308) -> ("error out"=w2309:errorcluster)
      }
    }
    n1295 = call "LAB-IQ Error Handler - Message Handling Loop.vi"("error in (no error)"=w2255, "Message Queue"=w2257) -> ("dup error in"=w2256:errorcluster)  [unwired: 8 in, 1 out]
  }
  n1296 = while {
    shift-right: [w2328] -> _
    shift-left: w6 -> [w2329]
    tunnel: [w2322] -> _
    tunnel: w23 -> [w2320]
    tunnel: w13 -> [w2319]
    tunnel: w25 -> [w2318]
    stop <- w2327 stop-if-true
    # "Load Pid  Handling Loop"
    n1297 = call "Dequeue Message.vi"("error in (no error)"=w2319, "Message Queue"=w2320) -> ("error out"=w2326:errorcluster, "Message Data"=w2324:variant, "Message"=w2325:string, "dup Message Queue"=w2323:refnum<queue>)  [unwired: 6 in]
    n1298 = case "Message Cases" shown="\"Load Pid Main\"" w2325 {
      selector: w2325 -> [_ _ _ _ _ w2394]
      tunnel: w2323 -> [w2330 w2351 _ w2381 w2393 _]
      tunnel: w2326 -> [w2333 w2349 w2378 w2385 w2387 _]
      tunnel: [w2334 w2352 w2372 w2383 w2389 w2395] -> w2321
      tunnel: w2329 -> [w2332 w2338 w2377 w2384 w2392 w2396]
      tunnel: [w2332 w2338 w2377 w2384 w2392 w2396] -> w2328
      tunnel: [_ _ _ _ TRUE _] -> w2327
      tunnel: w2324 -> [_ _ w2376 _ _ _]
      tunnel: w2318 -> [_ _ _ _ w2386 _]
      frame "init" {
        # "Initialize - All initialization work should take place in this message, since other loops can potentially enqueue messages that execute immediately after this one."
        n1299 = call-poly "Enqueue Message.vi"("error in (no error)"=w2333, "Message"="Load Pid Main", "Message Queue"=w2330) -> ("error out"=w2334:errorcluster)  [unwired: 7 in, 1 out]
      }
      frame "Load Pid Main" {
        n1300 = Unbundle By Name(w2338) -> ("Main Screen.Load En"=w2344:refnum<vi>)
        n1301 = Unbundle By Name(w2338) -> ("PID.apply load"=w2339:refnum<vi>)
        n1302 = property class="Bool (strict)"(reference=w2344) -> (reference out=w2342:refnum<vi>, error out=w2343:errorcluster, "Value"=w2337:bool)  [unwired: 1 in]
        n1303 = property class="Bool (strict)"(reference=w2339) -> (reference out=w2341:refnum<vi>, error out=w2340:errorcluster, "Value"=w2336:bool)  [unwired: 1 in]
        n1304 = Close Reference(reference=w2342, error in (no error)=w2343) -> ()  [unwired: 1 out]
        n1305 = Close Reference(reference=w2341, error in (no error)=w2340) -> ()  [unwired: 1 out]
        n1306 = Or(x=w2337, y=w2336) -> (x .or. y?=w2335:bool)
        n1307 = case shown="True" w2335 {
          tunnel: w2349 -> [w2353 w2356]
          tunnel: [w2353 w2355] -> w2345
          tunnel: w2338 -> [_ w2354]
          frame False {
          }
          frame True {
            n1308 = disable-structure shown="Enabled" {
              disable-tunnel: w2356 -> [w2359 w2363]
              disable-tunnel: [w2358 w2362] -> w2355
              disable-tunnel: w2354 -> [w2357 w2361]
              frame Disabled {
                n1309 = call "load pid.vi"("error in (no error)"=w2359, "main ref"=w2357) -> ("error out"=w2358:errorcluster)  [unwired: 9 in]
              }
              frame Enabled {
                n1310 = call "NEW LOAD CELL PID.vi"("error in (no error)"=w2363, "Checkbox"=TRUE, "main ref"=w2361) -> ("error out"=w2362:errorcluster)  [unwired: 8 in]
              }
            }
          }
        }
        n1311 = Unbundle By Name(w2338) -> ("Main Home Screen.EXIT"=w2350:refnum<vi>)
        n1312 = property class="Bool (strict)"(reference=w2350) -> (reference out=w2347:refnum<vi>, error out=w2348:errorcluster, "Value"=w2346:bool)  [unwired: 1 in]
        n1313 = case shown="False" w2346 {
          tunnel: [w2366 w2370] -> w2352
          tunnel: w2351 -> [w2365 w2369]
          tunnel: w2345 -> [w2364 w2368]
          frame True {
            n1314 = call-poly "Enqueue Message.vi"("error in (no error)"=w2364, "Message"="Confirm Quit", "Message Queue"=w2365) -> ("error out"=w2366:errorcluster)  [unwired: 7 in, 1 out]
          }
          frame False {
            n1315 = call-poly "Enqueue Message.vi"("error in (no error)"=w2368, "Message"="Load Pid Main", "Message Queue"=w2369) -> ("error out"=w2370:errorcluster)  [unwired: 7 in, 1 out]
          }
        }
        n1316 = Close Reference(reference=w2347, error in (no error)=w2348) -> ()  [unwired: 1 out]
      }
      frame "Error" {
        # "#CodeRecommended - If you ever change the name of this \"Error\" message, you'll need to update the name in the Check Loop Error.vi as well."
        # "#CodeRecommended - Consider creating a system for logging errors in some way. These errors are for notification purposes only. Handling of specific errors should be performed in the message frames that generated the error."
        # "Error - Display an error dialog. This message is sent by the \"Error Handler\" VIs at the end of other loops in this application."
        n1317 = Variant To Data(error in=w2378, type=errorcluster {"status"=FALSE, "code"=0, "source"=""} ("error constant"), Variant=w2376) -> (data=w2374:errorcluster, error out=w2373:errorcluster)
        n1318 = call <vilib>:"Simple Error Handler.vi"("error in (no error)"=w2374) -> ()  [unwired: 4 in, 5 out]
        n1319 = Merge Errors(w2373) -> (w2372:errorcluster)
      }
      frame "Confirm Quit" {
        # "#CodeNeeded - If you want to provide an \"Are you sure\" dialog (or some other notification) before the application exits, place that code here. This message is typically sent from a Panel Close? event."
        # "Confirm Quit - Message that can confirm whether or not the user wants to exit the application."
        n1320 = call-poly "Enqueue Message.vi"("Priority Message? (F)"=TRUE, "error in (no error)"=w2385, "Message"="Exit", "Message Queue"=w2381) -> ("error out"=w2382:errorcluster)  [unwired: 6 in, 1 out]
        n1321 = Merge Errors(w2382) -> (w2383:errorcluster)
      }
      frame "Exit" {
        # "Stop the VI"
        # "Release the message queue reference"
        # "#CodeNeeded - Add any required cleanup code here. Note that if 'Exit' was called as a result of an error, an error dialog will be displayed. Add any custom error handling for an 'Exit' condition here as well."
        # "Exit - Exit the application."
        n1322 = call "Fire User Event - Stop.vi"("User Event - Stop"=w2386) -> ("error out"=w2388:errorcluster)  [unwired: 10 in]
        n1323 = Release Queue(queue=w2393, error in (no error)=w2387) -> (error out=w2390:errorcluster)  [unwired: 1 in, 2 out]
        n1324 = Merge Errors(w2388, w2390) -> (w2389:errorcluster)
      }
      frame Default {
        # "'Default' case only runs if there is a message that isn't defined in any of the other cases.  Output a programming error."
        n1325 = xnode "Error Ring"("parameter 0"=w2394) -> ("error out"=w2395:errorcluster)
      }
    }
    n1326 = call "LAB-IQ Error Handler - Message Handling Loop.vi"("error in (no error)"=w2321, "Message Queue"=w2323) -> ("dup error in"=w2322:errorcluster)  [unwired: 8 in, 1 out]
  }
  n1327 = while {
    shift-right: [w2414] -> _
    shift-left: w6 -> [w2415]
    tunnel: [w2408] -> _
    tunnel: w22 -> [w2406]
    tunnel: w13 -> [w2405]
    tunnel: w25 -> [w2404]
    stop <- w2413 stop-if-true
    # "Report  Handling Loop"
    n1328 = call "Dequeue Message.vi"("error in (no error)"=w2405, "Message Queue"=w2406) -> ("error out"=w2412:errorcluster, "Message Data"=w2410:variant, "Message"=w2411:string, "dup Message Queue"=w2409:refnum<queue>)  [unwired: 6 in]
    n1329 = case "Message Cases" shown="\"Report Main\"" w2411 {
      selector: w2411 -> [_ _ _ _ _ w2459]
      tunnel: w2409 -> [w2416 w2427 _ w2446 w2458 _]
      tunnel: w2412 -> [w2419 w2424 w2443 w2450 w2452 _]
      tunnel: [w2420 w2428 w2437 w2448 w2454 w2460] -> w2407
      tunnel: w2415 -> [w2418 w2426 w2442 w2449 w2457 w2461]
      tunnel: [w2418 w2426 w2442 w2449 w2457 w2461] -> w2414
      tunnel: [_ _ _ _ TRUE _] -> w2413
      tunnel: w2410 -> [_ _ w2441 _ _ _]
      tunnel: w2404 -> [_ _ _ _ w2451 _]
      frame "init" {
        # "Initialize - All initialization work should take place in this message, since other loops can potentially enqueue messages that execute immediately after this one."
        n1330 = call-poly "Enqueue Message.vi"("error in (no error)"=w2419, "Message"="Report Main", "Message Queue"=w2416) -> ("error out"=w2420:errorcluster)  [unwired: 7 in, 1 out]
      }
      frame "Report Main" {
        n1331 = Unbundle By Name(w2426) -> ("Main Home Screen.EXIT"=w2425:refnum<vi>)
        n1332 = property class="Bool (strict)"(reference=w2425) -> (reference out=w2422:refnum<vi>, error out=w2423:errorcluster, "Value"=w2421:bool)  [unwired: 1 in]
        n1333 = case shown="False" w2421 {
          tunnel: [w2431 w2435] -> w2428
          tunnel: w2427 -> [w2430 w2434]
          tunnel: w2424 -> [w2429 w2433]
          frame True {
            n1334 = call-poly "Enqueue Message.vi"("error in (no error)"=w2429, "Message"="Confirm Quit", "Message Queue"=w2430) -> ("error out"=w2431:errorcluster)  [unwired: 7 in, 1 out]
          }
          frame False {
            n1335 = call-poly "Enqueue Message.vi"("error in (no error)"=w2433, "Message"="Report Main", "Message Queue"=w2434) -> ("error out"=w2435:errorcluster)  [unwired: 7 in, 1 out]
          }
        }
        n1336 = Close Reference(reference=w2422, error in (no error)=w2423) -> ()  [unwired: 1 out]
      }
      frame "Error" {
        # "#CodeRecommended - If you ever change the name of this \"Error\" message, you'll need to update the name in the Check Loop Error.vi as well."
        # "#CodeRecommended - Consider creating a system for logging errors in some way. These errors are for notification purposes only. Handling of specific errors should be performed in the message frames that generated the error."
        # "Error - Display an error dialog. This message is sent by the \"Error Handler\" VIs at the end of other loops in this application."
        n1337 = Variant To Data(error in=w2443, type=errorcluster {"status"=FALSE, "code"=0, "source"=""} ("error constant"), Variant=w2441) -> (data=w2439:errorcluster, error out=w2438:errorcluster)
        n1338 = call <vilib>:"Simple Error Handler.vi"("error in (no error)"=w2439) -> ()  [unwired: 4 in, 5 out]
        n1339 = Merge Errors(w2438) -> (w2437:errorcluster)
      }
      frame "Confirm Quit" {
        # "#CodeNeeded - If you want to provide an \"Are you sure\" dialog (or some other notification) before the application exits, place that code here. This message is typically sent from a Panel Close? event."
        # "Confirm Quit - Message that can confirm whether or not the user wants to exit the application."
        n1340 = call-poly "Enqueue Message.vi"("Priority Message? (F)"=TRUE, "error in (no error)"=w2450, "Message"="Exit", "Message Queue"=w2446) -> ("error out"=w2447:errorcluster)  [unwired: 6 in, 1 out]
        n1341 = Merge Errors(w2447) -> (w2448:errorcluster)
      }
      frame "Exit" {
        # "Stop the VI"
        # "Release the message queue reference"
        # "#CodeNeeded - Add any required cleanup code here. Note that if 'Exit' was called as a result of an error, an error dialog will be displayed. Add any custom error handling for an 'Exit' condition here as well."
        # "Exit - Exit the application."
        n1342 = call "Fire User Event - Stop.vi"("User Event - Stop"=w2451) -> ("error out"=w2453:errorcluster)  [unwired: 10 in]
        n1343 = Release Queue(queue=w2458, error in (no error)=w2452) -> (error out=w2455:errorcluster)  [unwired: 1 in, 2 out]
        n1344 = Merge Errors(w2453, w2455) -> (w2454:errorcluster)
      }
      frame Default {
        # "'Default' case only runs if there is a message that isn't defined in any of the other cases.  Output a programming error."
        n1345 = xnode "Error Ring"("parameter 0"=w2459) -> ("error out"=w2460:errorcluster)
      }
    }
    n1346 = call "LAB-IQ Error Handler - Message Handling Loop.vi"("error in (no error)"=w2407, "Message Queue"=w2409) -> ("dup error in"=w2408:errorcluster)  [unwired: 8 in, 1 out]
  }
  n1347 = Obtain Queue(max queue size (-1, unlimited)=w14, name (unnamed)=w7, element data type=w7, error in (no error)=w13) -> (queue out=w15:refnum<queue>, error out=w8:errorcluster)  [unwired: 1 in, 1 out]
  n1348 = call "HEAVE WRITE FGV.vi"("Enum - Menu"=Heave_Write_enum."INIT", "error in (no error)"=w8, "main ref"=w6) -> ("error out"=w12:errorcluster)  [unwired: 8 in]
  n1349 = call "Stall Data Flow.vim"("value in"=w12, "milliseconds to wait"=u32 1000) -> ("value out"=w10:errorcluster)  [unwired: 1 out]
  n1350 = UDP Open(8:w10, 9:-1 ("timeout ms (25000)"), 10:"192.168.1.10" ("service name"), 11:u16 8889 ("port")) -> (port=w4:refnum<k16>, 0:w5:errorcluster)  [unwired: 1 in, 1 out]
  n1351 = Unregister For Events(event registration refnum=w60, error in=w58) -> (error out=w61:errorcluster)
  n1352 = while {
    tunnel: w15 -> [w2477]
    tunnel: w8 -> [w2476]
    tunnel: w6 -> [w2471]
    stop <- w2470 stop-if-true
    # "Dequeue Loop"
    n1353 = Unbundle By Name(w2471) -> ("Main Home Screen.EXIT"=w2472:refnum<vi>)
    n1354 = Dequeue Element(queue=w2477, error in (no error)=w2476) -> (element=w2475:string)  [unwired: 4 out]
    "Heave and Surge Read" <- w2475
    n1355 = property class="Bool (strict)"(reference=w2472) -> (reference out=w2474:refnum<vi>, error out=w2473:errorcluster, "Value"=w2470:bool)  [unwired: 1 in]
    n1356 = call "HEAVE READ.vi"("Heave and Surge Read in"=w2475, "Data Cluster"=w2471) -> ()  [unwired: 9 in, 1 out]
    n1357 = local read "seconds to wait"() -> (w2469:dbl)
    n1358 = Close Reference(reference=w2474, error in (no error)=w2473) -> ()  [unwired: 1 out]
    n1359 = call <vilib>:"High Resolution Polling Wait.vi"("seconds to wait"=w2469) -> ()  [unwired: 10 in, 1 out]
  }
  n1360 = while {
    tunnel: w15 -> [w2493]
    tunnel: w5 -> [w2492]
    tunnel: w6 -> [w2482]
    tunnel: w4 -> [w2479]
    tunnel: [w2478] -> _
    stop <- w2486 stop-if-true
    # "Enqueue Loop"
    n1361 = Unbundle By Name(w2482) -> ("Heave AND Surge.Read Heave Temp"=w2485:refnum<vi>)
    n1362 = Unbundle By Name(w2482) -> ("Main Home Screen.EXIT"=w2489:refnum<vi>)
    n1363 = property class="Bool (strict)"(reference=w2485) -> (reference out=w2483:refnum<vi>, error out=w2484:errorcluster, "Value"=w2481:bool)  [unwired: 1 in]
    n1364 = property class="Bool (strict)"(reference=w2489) -> (reference out=w2487:refnum<vi>, error out=w2488:errorcluster, "Value"=w2486:bool)  [unwired: 1 in]
    n1365 = case shown="True" w2481 {
      tunnel: w2492 -> [w2495 w2502]
      tunnel: [w2495 w2506] -> w2491
      tunnel: ["" ("HEAVE OUT") w2505] -> w2490
      tunnel: w2482 -> [_ _]
      tunnel: w2479 -> [w2494 w2500]
      tunnel: [w2494 w2497] -> w2478
      frame False {
      }
      frame True {
        n1366 = UDP Read(connection ID=w2500, max size (548)=100, timeout ms (25000)=-1, 8:w2502) -> (data out=w2499:string, error out=w2501:errorcluster, 3:w2498:refnum<k16>)  [unwired: 2 out]
        n1367 = case shown="No Error" w2501 {
          tunnel: w2501 -> [_ w2519]
          tunnel: [_ w2518] -> w2506
          tunnel: [w2508 w2517] -> w2505
          tunnel: w2499 -> [w2508 w2517]
          tunnel: w2498 -> [w2507 w2510]
          tunnel: [w2507 w2509] -> w2497
          frame No Error {
          }
          frame Error {
            n1368 = call <vilib>:"Clear Errors.vi"("error in (no error)"=w2519) -> ("error out"=w2512:errorcluster)  [unwired: 5 in, 1 out]
            n1369 = UDP Close(connection ID=w2510, 8:w2512) -> (error out=w2516:errorcluster)  [unwired: 1 out]
            n1370 = call "Stall Data Flow.vim"("value in"=w2516, "milliseconds to wait"=u32 1000) -> ("value out"=w2513:errorcluster)  [unwired: 1 out]
            n1371 = UDP Open(8:w2513, 11:u16 8888 ("port")) -> (port=w2509:refnum<k16>, 0:w2511:errorcluster)  [unwired: 3 in, 1 out]
            n1372 = call <vilib>:"Clear Errors.vi"("error in (no error)"=w2511) -> ("error out"=w2518:errorcluster)  [unwired: 5 in, 1 out]
          }
        }
      }
    }
    n1373 = Close Reference(reference=w2483, error in (no error)=w2484) -> ()  [unwired: 1 out]
    n1374 = Close Reference(reference=w2487, error in (no error)=w2488) -> ()  [unwired: 1 out]
    n1375 = call <vilib>:"High Resolution Polling Wait.vi"("seconds to wait"="seconds to wait") -> ()  [unwired: 10 in, 1 out]
    n1376 = Enqueue Element(queue=w2493, element=w2490, error in (no error)=w2491) -> ()  [unwired: 4 out]
  }
  n1377 = Merge Errors(w61, w64, w36, w33, w31, w30) -> (w62:errorcluster)
  n1378 = call "Destroy User Event - Stop.vi"("error in (no error)"=w62, "User Event - Stop"=w25) -> ("error out"=w59:errorcluster)  [unwired: 9 in]
  n1379 = disable-structure shown="RUN_TIME_ENGINE==True" {
    disable-tunnel: w59 -> [_ _]
    frame condition #0 (active) {
    }
    frame condition #1 {
      # "Call Quit LabVIEW if running as a built application."
      n1380 = Quit LabVIEW() -> ()  [unwired: 1 in]
    }
  }
